vi "4 en linea.vi"() -> ()   [LabVIEW 2021]
panel:
  in  "Restet Marcador":bool
  out "Player Verde":dbl
  out "Player Rojo":dbl
  in  "OK Button":bool
  out "verde":bool
  in  "col7":bool
  in  "col6":bool
  in  "col5":bool
  in  "col4":bool
  in  "col3":bool
  in  "col2":bool
  in  "col1":bool
  in  "Ring 42":u16(ring)
  in  "Ring 41":u16(ring)
  in  "Ring 40":u16(ring)
  in  "Ring 39":u16(ring)
  in  "Ring 38":u16(ring)
  in  "Ring 37":u16(ring)
  in  "Ring 36":u16(ring)
  in  "Ring 35":u16(ring)
  in  "Ring 34":u16(ring)
  in  "Ring 33":u16(ring)
  in  "Ring 32":u16(ring)
  in  "Ring 31":u16(ring)
  in  "Ring 30":u16(ring)
  in  "Ring 29":u16(ring)
  in  "Ring 28":u16(ring)
  in  "Ring 27":u16(ring)
  in  "Ring 26":u16(ring)
  in  "Ring 25":u16(ring)
  in  "Ring 24":u16(ring)
  in  "Ring 23":u16(ring)
  in  "Ring 22":u16(ring)
  in  "Ring 21":u16(ring)
  in  "Ring 20":u16(ring)
  in  "Ring 19":u16(ring)
  in  "Ring 18":u16(ring)
  in  "Ring 17":u16(ring)
  in  "Ring 16":u16(ring)
  in  "Ring 15":u16(ring)
  in  "Ring 14":u16(ring)
  in  "Ring 13":u16(ring)
  in  "Ring 12":u16(ring)
  in  "Ring 11":u16(ring)
  in  "Ring 10":u16(ring)
  in  "Ring 9":u16(ring)
  in  "Ring 8":u16(ring)
  in  "Ring 7":u16(ring)
  in  "Ring 6":u16(ring)
  in  "Ring 5":u16(ring)
  in  "Ring 4":u16(ring)
  in  "Ring 3":u16(ring)
  in  "Ring 2":u16(ring)
  in  "Ring 1":u16(ring)
  # "4 EN LINEA"
  # "TURNO"
  # "MARCADOR"
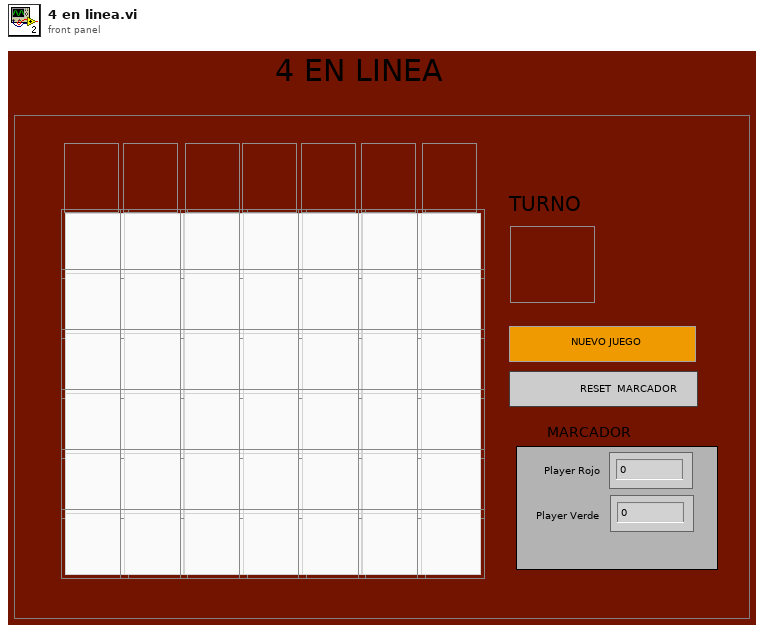
[diagram p1: front panel]
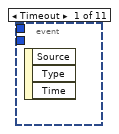
[diagram p12: hidden frame]
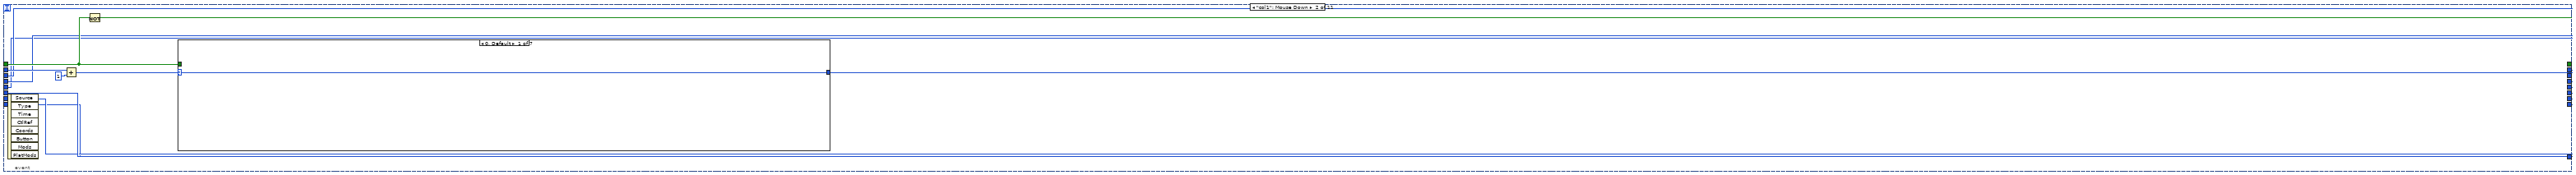
[diagram p13: hidden frame]
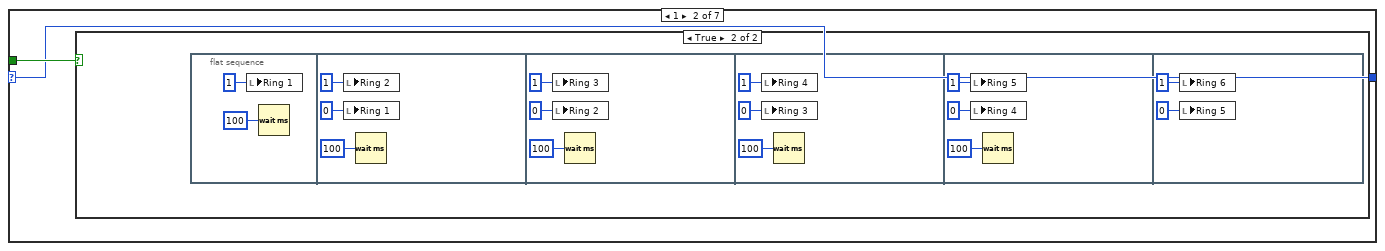
[diagram p14: hidden frame]
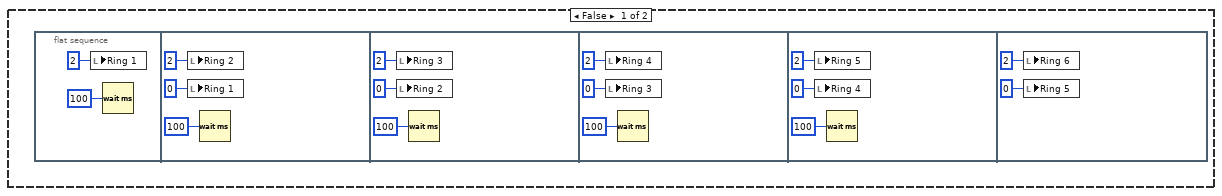
[diagram p15: hidden frame]
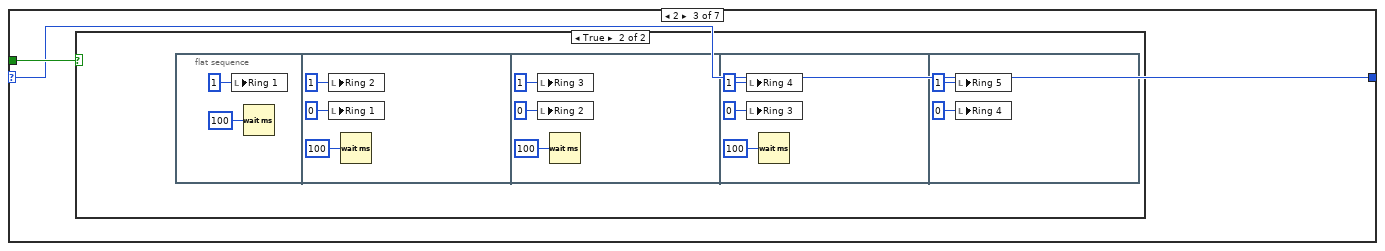
[diagram p16: hidden frame]
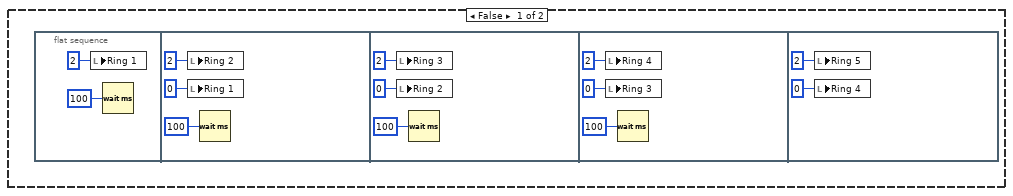
[diagram p17: hidden frame]
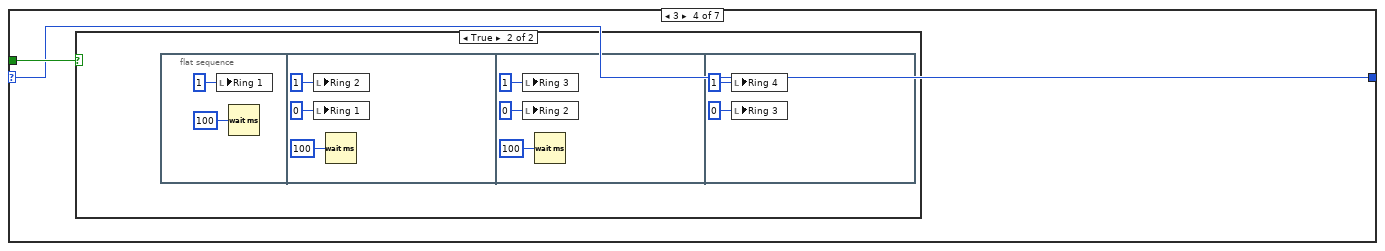
[diagram p18: hidden frame]
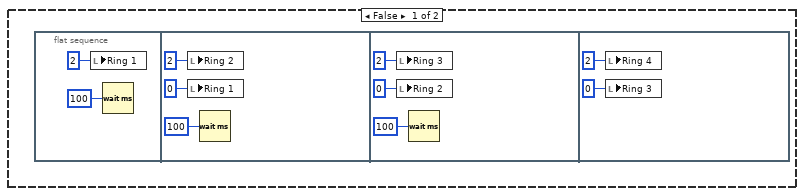
[diagram p19: hidden frame]
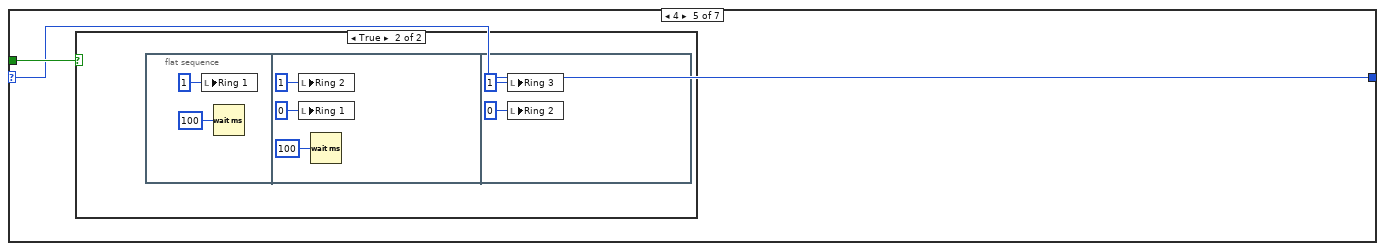
[diagram p20: hidden frame]
diagram:
  w2 = u16 0 ("Ring 42")
  w3 = u16 0 ("Ring 36")
  w4 = u16 0 ("Ring 30")
  w5 = u16 0 ("Ring 24")
  w6 = u16 0 ("Ring 18")
  w7 = u16 0 ("Ring 12")
  w8 = 0
  n1 = local write "Ring 1"(w8) -> ()
  n2 = local write "Ring 6"(w8) -> ()
  n3 = local write "Ring 5"(w8) -> ()
  n4 = local write "Ring 4"(w8) -> ()
  n5 = local write "Ring 3"(w8) -> ()
  n6 = local write "Ring 2"(w8) -> ()
  n7 = local write "Ring 7"(w7) -> ()
  n8 = local write "Ring 12"(w7) -> ()
  n9 = local write "Ring 11"(w7) -> ()
  n10 = local write "Ring 10"(w7) -> ()
  n11 = local write "Ring 9"(w7) -> ()
  n12 = local write "Ring 8"(w7) -> ()
  n13 = local write "Ring 13"(w6) -> ()
  n14 = local write "Ring 18"(w6) -> ()
  n15 = local write "Ring 17"(w6) -> ()
  n16 = local write "Ring 16"(w6) -> ()
  n17 = local write "Ring 15"(w6) -> ()
  n18 = local write "Ring 14"(w6) -> ()
  n19 = local write "Ring 19"(w5) -> ()
  n20 = local write "Ring 24"(w5) -> ()
  n21 = local write "Ring 23"(w5) -> ()
  n22 = local write "Ring 22"(w5) -> ()
  n23 = local write "Ring 21"(w5) -> ()
  n24 = local write "Ring 20"(w5) -> ()
  n25 = local write "Ring 25"(w4) -> ()
  n26 = local write "Ring 30"(w4) -> ()
  n27 = local write "Ring 29"(w4) -> ()
  n28 = local write "Ring 28"(w4) -> ()
  n29 = local write "Ring 27"(w4) -> ()
  n30 = local write "Ring 26"(w4) -> ()
  n31 = local write "Ring 31"(w3) -> ()
  n32 = local write "Ring 36"(w3) -> ()
  n33 = local write "Ring 35"(w3) -> ()
  n34 = local write "Ring 34"(w3) -> ()
  n35 = local write "Ring 33"(w3) -> ()
  n36 = local write "Ring 32"(w3) -> ()
  n37 = local write "Ring 37"(w2) -> ()
  n38 = local write "Ring 42"(w2) -> ()
  n39 = local write "Ring 41"(w2) -> ()
  n40 = local write "Ring 40"(w2) -> ()
  n41 = local write "Ring 39"(w2) -> ()
  n42 = local write "Ring 38"(w2) -> ()
  n43 = while {
    shift-right: [w2185] -> _
    shift-left: FALSE ("verde") -> [w94]
    shift-right: [w2184] -> _
    shift-left: _ -> [w2182]
    shift-right: [w2183] -> _
    shift-left: _ -> [w2181]
    shift-right: [w2180] -> _
    shift-left: _ -> [w2178]
    shift-right: [w2179] -> _
    shift-left: _ -> [w2177]
    shift-right: [w2175] -> _
    shift-left: _ -> [w2176]
    shift-right: [w2173] -> _
    shift-left: _ -> [w2174]
    shift-right: [w2171] -> _
    shift-left: _ -> [w2172]
    stop <- FALSE stop-if-true
    n44 = local write "verde"(w94) -> ()
    n45 = local read "Ring 5"() -> (w2154:u16)
    n46 = local read "Ring 4"() -> (w2152:u16)
    n47 = local read "Ring 3"() -> (w2150:u16)
    n48 = local read "Ring 2"() -> (w2148:u16)
    n49 = local read "Ring 3"() -> (w2167:u16)
    n50 = local read "Ring 4"() -> (w2168:u16)
    n51 = local read "Ring 5"() -> (w2169:u16)
    n52 = local read "Ring 6"() -> (w2170:u16)
    n53 = local read "Ring 4"() -> (w2137:u16)
    n54 = local read "Ring 3"() -> (w2134:u16)
    n55 = local read "Ring 2"() -> (w2135:u16)
    n56 = local read "Ring 1"() -> (w2136:u16)
    n57 = local read "Ring 42"() -> (w1578:u16)
    n58 = local read "Ring 36"() -> (w1577:u16)
    n59 = local read "Ring 30"() -> (w1576:u16)
    n60 = local read "Ring 24"() -> (w1575:u16)
    n61 = local read "Ring 36"() -> (w1582:u16)
    n62 = local read "Ring 30"() -> (w1581:u16)
    n63 = local read "Ring 24"() -> (w1580:u16)
    n64 = local read "Ring 18"() -> (w1579:u16)
    n65 = local read "Ring 30"() -> (w1586:u16)
    n66 = local read "Ring 24"() -> (w1585:u16)
    n67 = local read "Ring 18"() -> (w1584:u16)
    n68 = local read "Ring 12"() -> (w1583:u16)
    n69 = local read "Ring 24"() -> (w1590:u16)
    n70 = local read "Ring 18"() -> (w1589:u16)
    n71 = local read "Ring 12"() -> (w1588:u16)
    n72 = local read "Ring 6"() -> (w1587:u16)
    n73 = event shown="[7] \"col7\": Mouse Down" {
      selector: _ -> [_ _ _ _ _ _ _ _ _ _ _]
      dyn-events: _ -> [_ _ _ _ _ _ _ _ _ _ _]
      timeout: _ -> [_ _ _ _ _ _ _ _ _ _ _]
      tunnel: w94 -> [_ w2225 w2352 w2474 w2600 w2729 w2857 w2977 _ w3106 _]
      tunnel: [_ w2226 w2353 w2475 w2599 w2730 w2856 w2978 _ w3106 w3115] -> w2185
      tunnel: [_ w2224 w2347 w2478 w2603 w2725 w2855 w2984 _ _ _] -> w2184
      tunnel: [_ w2220 w2351 w2479 w2602 w2726 w2854 w2983 _ w3112 _] -> w2183
      tunnel: w2182 -> [_ w2223 w2347 w2478 w2603 w2725 w2855 w2984 _ w3113 _]
      tunnel: w2181 -> [_ w2220 w2350 w2479 w2602 w2726 w2854 w2983 _ w3112 _]
      tunnel: [_ w2219 w2346 w2480 w2601 w2727 w2853 w2982 _ w3111 _] -> w2180
      tunnel: [_ w2218 w2345 w2472 w2605 w2728 w2852 w2981 _ w3110 _] -> w2179
      tunnel: w2178 -> [_ w2219 w2346 w2473 w2601 w2727 w2853 w2982 _ w3111 _]
      tunnel: w2177 -> [_ w2218 w2345 w2472 w2604 w2728 w2852 w2981 _ w3110 _]
      tunnel: w2176 -> [_ w2217 w2344 w2471 w2598 w2733 w2851 w2980 _ w3109 _]
      tunnel: [_ w2217 w2344 w2471 w2598 w2731 w2851 w2980 _ w3109 _] -> w2175
      tunnel: w2174 -> [_ w2216 w2343 w2470 w2597 w2724 w2860 w2979 _ w3108 _]
      tunnel: [_ w2216 w2343 w2470 w2597 w2724 w2858 w2979 _ w3108 _] -> w2173
      tunnel: w2172 -> [_ w2215 w2342 w2469 w2596 w2723 w2850 w2987 _ w3107 _]
      tunnel: [_ w2215 w2342 w2469 w2596 w2723 w2850 w2985 _ w3107 _] -> w2171
      tunnel: [_ _ _ _ _ _ _ _ _ w3113 _] -> _
      event Timeout {
        n74 = event-data() -> ()  [unwired: 1 in, 3 out]
      }
      event "col1": Mouse Down {
        n75 = event-data() -> ()  [unwired: 1 in, 8 out]
        n76 = Add(x=w2223, y=1) -> (x+y=w2222:i32)
        n77 = Not(x=w2225) -> (.not. x?=w2226:bool)
        n78 = case shown="0, Default" w2222 {
          selector: w2222 -> [w2227 w2228 w2262 w2290 w2312 w2328 w2338]
          tunnel: w2225 -> [_ w2229 w2263 w2291 w2313 w2329 w2339]
          tunnel: [w2227 w2228 w2262 w2290 w2312 w2328 w2338] -> w2224
          frame 0, Default {
          }
          frame 1 {
            n79 = case shown="True" w2229 {
              frame False {
                n80 = flat-sequence {
                  frame #0 {
                    n81 = local write "Ring 1"(u16 2 ("Ring 1")) -> ()
                    n82 = Wait (ms)(milliseconds to wait=u32 100) -> ()  [unwired: 1 out]
                  }
                  frame #1 {
                    n83 = local write "Ring 2"(u16 2 ("Ring 2")) -> ()
                    n84 = local write "Ring 1"(u16 0 ("Ring 1")) -> ()
                    n85 = Wait (ms)(milliseconds to wait=u32 100) -> ()  [unwired: 1 out]
                  }
                  frame #2 {
                    n86 = local write "Ring 3"(u16 2 ("Ring 3")) -> ()
                    n87 = local write "Ring 2"(u16 0 ("Ring 2")) -> ()
                    n88 = Wait (ms)(milliseconds to wait=u32 100) -> ()  [unwired: 1 out]
                  }
                  frame #3 {
                    n89 = local write "Ring 4"(u16 2 ("Ring 4")) -> ()
                    n90 = local write "Ring 3"(u16 0 ("Ring 3")) -> ()
                    n91 = Wait (ms)(milliseconds to wait=u32 100) -> ()  [unwired: 1 out]
                  }
                  frame #4 {
                    n92 = local write "Ring 5"(u16 2 ("Ring 5")) -> ()
                    n93 = local write "Ring 4"(u16 0 ("Ring 4")) -> ()
                    n94 = Wait (ms)(milliseconds to wait=u32 100) -> ()  [unwired: 1 out]
                  }
                  frame #5 {
                    n95 = local write "Ring 6"(u16 2 ("Ring 6")) -> ()
                    n96 = local write "Ring 5"(u16 0 ("Ring 5")) -> ()
                  }
                }
              }
              frame True {
                n97 = flat-sequence {
                  frame #0 {
                    n98 = local write "Ring 1"(u16 1 ("Ring 1")) -> ()
                    n99 = Wait (ms)(milliseconds to wait=u32 100) -> ()  [unwired: 1 out]
                  }
                  frame #1 {
                    n100 = local write "Ring 2"(u16 1 ("Ring 2")) -> ()
                    n101 = local write "Ring 1"(u16 0 ("Ring 1")) -> ()
                    n102 = Wait (ms)(milliseconds to wait=u32 100) -> ()  [unwired: 1 out]
                  }
                  frame #2 {
                    n103 = local write "Ring 3"(u16 1 ("Ring 3")) -> ()
                    n104 = local write "Ring 2"(u16 0 ("Ring 2")) -> ()
                    n105 = Wait (ms)(milliseconds to wait=u32 100) -> ()  [unwired: 1 out]
                  }
                  frame #3 {
                    n106 = local write "Ring 4"(u16 1 ("Ring 4")) -> ()
                    n107 = local write "Ring 3"(u16 0 ("Ring 3")) -> ()
                    n108 = Wait (ms)(milliseconds to wait=u32 100) -> ()  [unwired: 1 out]
                  }
                  frame #4 {
                    n109 = local write "Ring 5"(u16 1 ("Ring 5")) -> ()
                    n110 = local write "Ring 4"(u16 0 ("Ring 4")) -> ()
                    n111 = Wait (ms)(milliseconds to wait=u32 100) -> ()  [unwired: 1 out]
                  }
                  frame #5 {
                    n112 = local write "Ring 6"(u16 1 ("Ring 6")) -> ()
                    n113 = local write "Ring 5"(u16 0 ("Ring 5")) -> ()
                  }
                }
              }
            }
          }
          frame 2 {
            n114 = case shown="True" w2263 {
              frame False {
                n115 = flat-sequence {
                  frame #0 {
                    n116 = local write "Ring 1"(u16 2 ("Ring 1")) -> ()
                    n117 = Wait (ms)(milliseconds to wait=u32 100) -> ()  [unwired: 1 out]
                  }
                  frame #1 {
                    n118 = local write "Ring 2"(u16 2 ("Ring 2")) -> ()
                    n119 = local write "Ring 1"(u16 0 ("Ring 1")) -> ()
                    n120 = Wait (ms)(milliseconds to wait=u32 100) -> ()  [unwired: 1 out]
                  }
                  frame #2 {
                    n121 = local write "Ring 3"(u16 2 ("Ring 3")) -> ()
                    n122 = local write "Ring 2"(u16 0 ("Ring 2")) -> ()
                    n123 = Wait (ms)(milliseconds to wait=u32 100) -> ()  [unwired: 1 out]
                  }
                  frame #3 {
                    n124 = local write "Ring 4"(u16 2 ("Ring 4")) -> ()
                    n125 = local write "Ring 3"(u16 0 ("Ring 3")) -> ()
                    n126 = Wait (ms)(milliseconds to wait=u32 100) -> ()  [unwired: 1 out]
                  }
                  frame #4 {
                    n127 = local write "Ring 5"(u16 2 ("Ring 5")) -> ()
                    n128 = local write "Ring 4"(u16 0 ("Ring 4")) -> ()
                  }
                }
              }
              frame True {
                n129 = flat-sequence {
                  frame #0 {
                    n130 = local write "Ring 1"(u16 1 ("Ring 1")) -> ()
                    n131 = Wait (ms)(milliseconds to wait=u32 100) -> ()  [unwired: 1 out]
                  }
                  frame #1 {
                    n132 = local write "Ring 2"(u16 1 ("Ring 2")) -> ()
                    n133 = local write "Ring 1"(u16 0 ("Ring 1")) -> ()
                    n134 = Wait (ms)(milliseconds to wait=u32 100) -> ()  [unwired: 1 out]
                  }
                  frame #2 {
                    n135 = local write "Ring 3"(u16 1 ("Ring 3")) -> ()
                    n136 = local write "Ring 2"(u16 0 ("Ring 2")) -> ()
                    n137 = Wait (ms)(milliseconds to wait=u32 100) -> ()  [unwired: 1 out]
                  }
                  frame #3 {
                    n138 = local write "Ring 4"(u16 1 ("Ring 4")) -> ()
                    n139 = local write "Ring 3"(u16 0 ("Ring 3")) -> ()
                    n140 = Wait (ms)(milliseconds to wait=u32 100) -> ()  [unwired: 1 out]
                  }
                  frame #4 {
                    n141 = local write "Ring 5"(u16 1 ("Ring 5")) -> ()
                    n142 = local write "Ring 4"(u16 0 ("Ring 4")) -> ()
                  }
                }
              }
            }
          }
          frame 3 {
            n143 = case shown="True" w2291 {
              frame False {
                n144 = flat-sequence {
                  frame #0 {
                    n145 = local write "Ring 1"(u16 2 ("Ring 1")) -> ()
                    n146 = Wait (ms)(milliseconds to wait=u32 100) -> ()  [unwired: 1 out]
                  }
                  frame #1 {
                    n147 = local write "Ring 2"(u16 2 ("Ring 2")) -> ()
                    n148 = local write "Ring 1"(u16 0 ("Ring 1")) -> ()
                    n149 = Wait (ms)(milliseconds to wait=u32 100) -> ()  [unwired: 1 out]
                  }
                  frame #2 {
                    n150 = local write "Ring 3"(u16 2 ("Ring 3")) -> ()
                    n151 = local write "Ring 2"(u16 0 ("Ring 2")) -> ()
                    n152 = Wait (ms)(milliseconds to wait=u32 100) -> ()  [unwired: 1 out]
                  }
                  frame #3 {
                    n153 = local write "Ring 4"(u16 2 ("Ring 4")) -> ()
                    n154 = local write "Ring 3"(u16 0 ("Ring 3")) -> ()
                  }
                }
              }
              frame True {
                n155 = flat-sequence {
                  frame #0 {
                    n156 = local write "Ring 1"(u16 1 ("Ring 1")) -> ()
                    n157 = Wait (ms)(milliseconds to wait=u32 100) -> ()  [unwired: 1 out]
                  }
                  frame #1 {
                    n158 = local write "Ring 2"(u16 1 ("Ring 2")) -> ()
                    n159 = local write "Ring 1"(u16 0 ("Ring 1")) -> ()
                    n160 = Wait (ms)(milliseconds to wait=u32 100) -> ()  [unwired: 1 out]
                  }
                  frame #2 {
                    n161 = local write "Ring 3"(u16 1 ("Ring 3")) -> ()
                    n162 = local write "Ring 2"(u16 0 ("Ring 2")) -> ()
                    n163 = Wait (ms)(milliseconds to wait=u32 100) -> ()  [unwired: 1 out]
                  }
                  frame #3 {
                    n164 = local write "Ring 4"(u16 1 ("Ring 4")) -> ()
                    n165 = local write "Ring 3"(u16 0 ("Ring 3")) -> ()
                  }
                }
              }
            }
          }
          frame 4 {
            n166 = case shown="True" w2313 {
              frame False {
                n167 = flat-sequence {
                  frame #0 {
                    n168 = local write "Ring 1"(u16 2 ("Ring 1")) -> ()
                    n169 = Wait (ms)(milliseconds to wait=u32 100) -> ()  [unwired: 1 out]
                  }
                  frame #1 {
                    n170 = local write "Ring 2"(u16 2 ("Ring 2")) -> ()
                    n171 = local write "Ring 1"(u16 0 ("Ring 1")) -> ()
                    n172 = Wait (ms)(milliseconds to wait=u32 100) -> ()  [unwired: 1 out]
                  }
                  frame #2 {
                    n173 = local write "Ring 3"(u16 2 ("Ring 3")) -> ()
                    n174 = local write "Ring 2"(u16 0 ("Ring 2")) -> ()
                  }
                }
              }
              frame True {
                n175 = flat-sequence {
                  frame #0 {
                    n176 = local write "Ring 1"(u16 1 ("Ring 1")) -> ()
                    n177 = Wait (ms)(milliseconds to wait=u32 100) -> ()  [unwired: 1 out]
                  }
                  frame #1 {
                    n178 = local write "Ring 2"(u16 1 ("Ring 2")) -> ()
                    n179 = local write "Ring 1"(u16 0 ("Ring 1")) -> ()
                    n180 = Wait (ms)(milliseconds to wait=u32 100) -> ()  [unwired: 1 out]
                  }
                  frame #2 {
                    n181 = local write "Ring 3"(u16 1 ("Ring 3")) -> ()
                    n182 = local write "Ring 2"(u16 0 ("Ring 2")) -> ()
                  }
                }
              }
            }
          }
          frame 5 {
            n183 = case shown="True" w2329 {
              frame False {
                n184 = flat-sequence {
                  frame #0 {
                    n185 = local write "Ring 1"(u16 2 ("Ring 1")) -> ()
                    n186 = Wait (ms)(milliseconds to wait=u32 100) -> ()  [unwired: 1 out]
                  }
                  frame #1 {
                    n187 = local write "Ring 2"(u16 2 ("Ring 2")) -> ()
                    n188 = local write "Ring 1"(u16 0 ("Ring 1")) -> ()
                  }
                }
              }
              frame True {
                n189 = flat-sequence {
                  frame #0 {
                    n190 = local write "Ring 1"(u16 1 ("Ring 1")) -> ()
                    n191 = Wait (ms)(milliseconds to wait=u32 100) -> ()  [unwired: 1 out]
                  }
                  frame #1 {
                    n192 = local write "Ring 2"(u16 1 ("Ring 2")) -> ()
                    n193 = local write "Ring 1"(u16 0 ("Ring 1")) -> ()
                  }
                }
              }
            }
          }
          frame 6 {
            n194 = case shown="True" w2339 {
              frame False {
                n195 = flat-sequence {
                  frame #0 {
                    n196 = local write "Ring 1"(u16 2 ("Ring 1")) -> ()
                  }
                }
              }
              frame True {
                n197 = flat-sequence {
                  frame #0 {
                    n198 = local write "Ring 1"(u16 1 ("Ring 1")) -> ()
                  }
                }
              }
            }
          }
        }
      }
      event "col2": Mouse Down {
        n199 = event-data() -> ()  [unwired: 1 in, 8 out]
        n200 = Add(x=w2350, y=1) -> (x+y=w2349:i32)
        n201 = Not(x=w2352) -> (.not. x?=w2353:bool)
        n202 = case shown="1" w2349 {
          selector: w2349 -> [w2354 w2355 w2389 w2417 w2439 w2455 w2465]
          tunnel: w2352 -> [_ w2356 w2390 w2418 w2440 w2456 w2466]
          tunnel: [w2354 w2355 w2389 w2417 w2439 w2455 w2465] -> w2351
          frame 0, Default {
          }
          frame 1 {
            n203 = case shown="False" w2356 {
              frame False {
                n204 = flat-sequence {
                  frame #0 {
                    n205 = local write "Ring 7"(u16 2 ("Ring 1")) -> ()
                    n206 = Wait (ms)(milliseconds to wait=u32 100) -> ()  [unwired: 1 out]
                  }
                  frame #1 {
                    n207 = local write "Ring 8"(u16 2 ("Ring 2")) -> ()
                    n208 = local write "Ring 7"(u16 0 ("Ring 1")) -> ()
                    n209 = Wait (ms)(milliseconds to wait=u32 100) -> ()  [unwired: 1 out]
                  }
                  frame #2 {
                    n210 = local write "Ring 9"(u16 2 ("Ring 3")) -> ()
                    n211 = local write "Ring 8"(u16 0 ("Ring 2")) -> ()
                    n212 = Wait (ms)(milliseconds to wait=u32 100) -> ()  [unwired: 1 out]
                  }
                  frame #3 {
                    n213 = local write "Ring 10"(u16 2 ("Ring 4")) -> ()
                    n214 = local write "Ring 9"(u16 0 ("Ring 3")) -> ()
                    n215 = Wait (ms)(milliseconds to wait=u32 100) -> ()  [unwired: 1 out]
                  }
                  frame #4 {
                    n216 = local write "Ring 11"(u16 2 ("Ring 5")) -> ()
                    n217 = local write "Ring 10"(u16 0 ("Ring 4")) -> ()
                    n218 = Wait (ms)(milliseconds to wait=u32 100) -> ()  [unwired: 1 out]
                  }
                  frame #5 {
                    n219 = local write "Ring 12"(u16 2 ("Ring 6")) -> ()
                    n220 = local write "Ring 11"(u16 0 ("Ring 5")) -> ()
                  }
                }
              }
              frame True {
                n221 = flat-sequence {
                  frame #0 {
                    n222 = local write "Ring 7"(u16 1 ("Ring 1")) -> ()
                    n223 = Wait (ms)(milliseconds to wait=u32 100) -> ()  [unwired: 1 out]
                  }
                  frame #1 {
                    n224 = local write "Ring 8"(u16 1 ("Ring 2")) -> ()
                    n225 = local write "Ring 7"(u16 0 ("Ring 1")) -> ()
                    n226 = Wait (ms)(milliseconds to wait=u32 100) -> ()  [unwired: 1 out]
                  }
                  frame #2 {
                    n227 = local write "Ring 9"(u16 1 ("Ring 3")) -> ()
                    n228 = local write "Ring 8"(u16 0 ("Ring 2")) -> ()
                    n229 = Wait (ms)(milliseconds to wait=u32 100) -> ()  [unwired: 1 out]
                  }
                  frame #3 {
                    n230 = local write "Ring 10"(u16 1 ("Ring 4")) -> ()
                    n231 = local write "Ring 9"(u16 0 ("Ring 3")) -> ()
                    n232 = Wait (ms)(milliseconds to wait=u32 100) -> ()  [unwired: 1 out]
                  }
                  frame #4 {
                    n233 = local write "Ring 11"(u16 1 ("Ring 5")) -> ()
                    n234 = local write "Ring 10"(u16 0 ("Ring 4")) -> ()
                    n235 = Wait (ms)(milliseconds to wait=u32 100) -> ()  [unwired: 1 out]
                  }
                  frame #5 {
                    n236 = local write "Ring 12"(u16 1 ("Ring 6")) -> ()
                    n237 = local write "Ring 11"(u16 0 ("Ring 5")) -> ()
                  }
                }
              }
            }
          }
          frame 2 {
            n238 = case shown="True" w2390 {
              frame False {
                n239 = flat-sequence {
                  frame #0 {
                    n240 = local write "Ring 7"(u16 2 ("Ring 1")) -> ()
                    n241 = Wait (ms)(milliseconds to wait=u32 100) -> ()  [unwired: 1 out]
                  }
                  frame #1 {
                    n242 = local write "Ring 8"(u16 2 ("Ring 2")) -> ()
                    n243 = local write "Ring 7"(u16 0 ("Ring 1")) -> ()
                    n244 = Wait (ms)(milliseconds to wait=u32 100) -> ()  [unwired: 1 out]
                  }
                  frame #2 {
                    n245 = local write "Ring 9"(u16 2 ("Ring 3")) -> ()
                    n246 = local write "Ring 8"(u16 0 ("Ring 2")) -> ()
                    n247 = Wait (ms)(milliseconds to wait=u32 100) -> ()  [unwired: 1 out]
                  }
                  frame #3 {
                    n248 = local write "Ring 10"(u16 2 ("Ring 4")) -> ()
                    n249 = local write "Ring 9"(u16 0 ("Ring 3")) -> ()
                    n250 = Wait (ms)(milliseconds to wait=u32 100) -> ()  [unwired: 1 out]
                  }
                  frame #4 {
                    n251 = local write "Ring 11"(u16 2 ("Ring 5")) -> ()
                    n252 = local write "Ring 10"(u16 0 ("Ring 4")) -> ()
                  }
                }
              }
              frame True {
                n253 = flat-sequence {
                  frame #0 {
                    n254 = local write "Ring 7"(u16 1 ("Ring 1")) -> ()
                    n255 = Wait (ms)(milliseconds to wait=u32 100) -> ()  [unwired: 1 out]
                  }
                  frame #1 {
                    n256 = local write "Ring 8"(u16 1 ("Ring 2")) -> ()
                    n257 = local write "Ring 7"(u16 0 ("Ring 1")) -> ()
                    n258 = Wait (ms)(milliseconds to wait=u32 100) -> ()  [unwired: 1 out]
                  }
                  frame #2 {
                    n259 = local write "Ring 9"(u16 1 ("Ring 3")) -> ()
                    n260 = local write "Ring 8"(u16 0 ("Ring 2")) -> ()
                    n261 = Wait (ms)(milliseconds to wait=u32 100) -> ()  [unwired: 1 out]
                  }
                  frame #3 {
                    n262 = local write "Ring 10"(u16 1 ("Ring 4")) -> ()
                    n263 = local write "Ring 9"(u16 0 ("Ring 3")) -> ()
                    n264 = Wait (ms)(milliseconds to wait=u32 100) -> ()  [unwired: 1 out]
                  }
                  frame #4 {
                    n265 = local write "Ring 11"(u16 1 ("Ring 5")) -> ()
                    n266 = local write "Ring 10"(u16 0 ("Ring 4")) -> ()
                  }
                }
              }
            }
          }
          frame 3 {
            n267 = case shown="False" w2418 {
              frame False {
                n268 = flat-sequence {
                  frame #0 {
                    n269 = local write "Ring 7"(u16 2 ("Ring 1")) -> ()
                    n270 = Wait (ms)(milliseconds to wait=u32 100) -> ()  [unwired: 1 out]
                  }
                  frame #1 {
                    n271 = local write "Ring 8"(u16 2 ("Ring 2")) -> ()
                    n272 = local write "Ring 7"(u16 0 ("Ring 1")) -> ()
                    n273 = Wait (ms)(milliseconds to wait=u32 100) -> ()  [unwired: 1 out]
                  }
                  frame #2 {
                    n274 = local write "Ring 9"(u16 2 ("Ring 3")) -> ()
                    n275 = local write "Ring 8"(u16 0 ("Ring 2")) -> ()
                    n276 = Wait (ms)(milliseconds to wait=u32 100) -> ()  [unwired: 1 out]
                  }
                  frame #3 {
                    n277 = local write "Ring 10"(u16 2 ("Ring 4")) -> ()
                    n278 = local write "Ring 9"(u16 0 ("Ring 3")) -> ()
                  }
                }
              }
              frame True {
                n279 = flat-sequence {
                  frame #0 {
                    n280 = local write "Ring 7"(u16 1 ("Ring 1")) -> ()
                    n281 = Wait (ms)(milliseconds to wait=u32 100) -> ()  [unwired: 1 out]
                  }
                  frame #1 {
                    n282 = local write "Ring 8"(u16 1 ("Ring 2")) -> ()
                    n283 = local write "Ring 7"(u16 0 ("Ring 1")) -> ()
                    n284 = Wait (ms)(milliseconds to wait=u32 100) -> ()  [unwired: 1 out]
                  }
                  frame #2 {
                    n285 = local write "Ring 9"(u16 1 ("Ring 3")) -> ()
                    n286 = local write "Ring 8"(u16 0 ("Ring 2")) -> ()
                    n287 = Wait (ms)(milliseconds to wait=u32 100) -> ()  [unwired: 1 out]
                  }
                  frame #3 {
                    n288 = local write "Ring 10"(u16 1 ("Ring 4")) -> ()
                    n289 = local write "Ring 9"(u16 0 ("Ring 3")) -> ()
                  }
                }
              }
            }
          }
          frame 4 {
            n290 = case shown="True" w2440 {
              frame False {
                n291 = flat-sequence {
                  frame #0 {
                    n292 = local write "Ring 7"(u16 2 ("Ring 1")) -> ()
                    n293 = Wait (ms)(milliseconds to wait=u32 100) -> ()  [unwired: 1 out]
                  }
                  frame #1 {
                    n294 = local write "Ring 8"(u16 2 ("Ring 2")) -> ()
                    n295 = local write "Ring 7"(u16 0 ("Ring 1")) -> ()
                    n296 = Wait (ms)(milliseconds to wait=u32 100) -> ()  [unwired: 1 out]
                  }
                  frame #2 {
                    n297 = local write "Ring 9"(u16 2 ("Ring 3")) -> ()
                    n298 = local write "Ring 8"(u16 0 ("Ring 2")) -> ()
                  }
                }
              }
              frame True {
                n299 = flat-sequence {
                  frame #0 {
                    n300 = local write "Ring 7"(u16 1 ("Ring 1")) -> ()
                    n301 = Wait (ms)(milliseconds to wait=u32 100) -> ()  [unwired: 1 out]
                  }
                  frame #1 {
                    n302 = local write "Ring 8"(u16 1 ("Ring 2")) -> ()
                    n303 = local write "Ring 7"(u16 0 ("Ring 1")) -> ()
                    n304 = Wait (ms)(milliseconds to wait=u32 100) -> ()  [unwired: 1 out]
                  }
                  frame #2 {
                    n305 = local write "Ring 9"(u16 1 ("Ring 3")) -> ()
                    n306 = local write "Ring 8"(u16 0 ("Ring 2")) -> ()
                  }
                }
              }
            }
          }
          frame 5 {
            n307 = case shown="True" w2456 {
              frame False {
                n308 = flat-sequence {
                  frame #0 {
                    n309 = local write "Ring 7"(u16 2 ("Ring 1")) -> ()
                    n310 = Wait (ms)(milliseconds to wait=u32 100) -> ()  [unwired: 1 out]
                  }
                  frame #1 {
                    n311 = local write "Ring 8"(u16 2 ("Ring 2")) -> ()
                    n312 = local write "Ring 7"(u16 0 ("Ring 1")) -> ()
                  }
                }
              }
              frame True {
                n313 = flat-sequence {
                  frame #0 {
                    n314 = local write "Ring 7"(u16 1 ("Ring 1")) -> ()
                    n315 = Wait (ms)(milliseconds to wait=u32 100) -> ()  [unwired: 1 out]
                  }
                  frame #1 {
                    n316 = local write "Ring 8"(u16 1 ("Ring 2")) -> ()
                    n317 = local write "Ring 7"(u16 0 ("Ring 1")) -> ()
                  }
                }
              }
            }
          }
          frame 6 {
            n318 = case shown="False" w2466 {
              frame False {
                n319 = flat-sequence {
                  frame #0 {
                    n320 = local write "Ring 7"(u16 2 ("Ring 1")) -> ()
                  }
                }
              }
              frame True {
                n321 = flat-sequence {
                  frame #0 {
                    n322 = local write "Ring 7"(u16 1 ("Ring 1")) -> ()
                  }
                }
              }
            }
          }
        }
      }
      event "col3": Mouse Down {
        n323 = event-data() -> ()  [unwired: 1 in, 8 out]
        n324 = Add(x=w2473, y=1) -> (x+y=w2477:i32)
        n325 = Not(x=w2474) -> (.not. x?=w2475:bool)
        n326 = case shown="1" w2477 {
          selector: w2477 -> [w2481 w2482 w2516 w2544 w2566 w2582 w2592]
          tunnel: w2474 -> [_ w2483 w2517 w2545 w2567 w2583 w2593]
          tunnel: [w2481 w2482 w2516 w2544 w2566 w2582 w2592] -> w2480
          frame 0, Default {
          }
          frame 1 {
            n327 = case shown="False" w2483 {
              frame False {
                n328 = flat-sequence {
                  frame #0 {
                    n329 = local write "Ring 13"(u16 2 ("Ring 1")) -> ()
                    n330 = Wait (ms)(milliseconds to wait=u32 100) -> ()  [unwired: 1 out]
                  }
                  frame #1 {
                    n331 = local write "Ring 14"(u16 2 ("Ring 2")) -> ()
                    n332 = local write "Ring 13"(u16 0 ("Ring 1")) -> ()
                    n333 = Wait (ms)(milliseconds to wait=u32 100) -> ()  [unwired: 1 out]
                  }
                  frame #2 {
                    n334 = local write "Ring 15"(u16 2 ("Ring 3")) -> ()
                    n335 = local write "Ring 14"(u16 0 ("Ring 2")) -> ()
                    n336 = Wait (ms)(milliseconds to wait=u32 100) -> ()  [unwired: 1 out]
                  }
                  frame #3 {
                    n337 = local write "Ring 16"(u16 2 ("Ring 4")) -> ()
                    n338 = local write "Ring 15"(u16 0 ("Ring 3")) -> ()
                    n339 = Wait (ms)(milliseconds to wait=u32 100) -> ()  [unwired: 1 out]
                  }
                  frame #4 {
                    n340 = local write "Ring 17"(u16 2 ("Ring 5")) -> ()
                    n341 = local write "Ring 16"(u16 0 ("Ring 4")) -> ()
                    n342 = Wait (ms)(milliseconds to wait=u32 100) -> ()  [unwired: 1 out]
                  }
                  frame #5 {
                    n343 = local write "Ring 18"(u16 2 ("Ring 6")) -> ()
                    n344 = local write "Ring 17"(u16 0 ("Ring 5")) -> ()
                  }
                }
              }
              frame True {
                n345 = flat-sequence {
                  frame #0 {
                    n346 = local write "Ring 13"(u16 1 ("Ring 1")) -> ()
                    n347 = Wait (ms)(milliseconds to wait=u32 100) -> ()  [unwired: 1 out]
                  }
                  frame #1 {
                    n348 = local write "Ring 14"(u16 1 ("Ring 2")) -> ()
                    n349 = local write "Ring 13"(u16 0 ("Ring 1")) -> ()
                    n350 = Wait (ms)(milliseconds to wait=u32 100) -> ()  [unwired: 1 out]
                  }
                  frame #2 {
                    n351 = local write "Ring 15"(u16 1 ("Ring 3")) -> ()
                    n352 = local write "Ring 14"(u16 0 ("Ring 2")) -> ()
                    n353 = Wait (ms)(milliseconds to wait=u32 100) -> ()  [unwired: 1 out]
                  }
                  frame #3 {
                    n354 = local write "Ring 16"(u16 1 ("Ring 4")) -> ()
                    n355 = local write "Ring 15"(u16 0 ("Ring 3")) -> ()
                    n356 = Wait (ms)(milliseconds to wait=u32 100) -> ()  [unwired: 1 out]
                  }
                  frame #4 {
                    n357 = local write "Ring 17"(u16 1 ("Ring 5")) -> ()
                    n358 = local write "Ring 16"(u16 0 ("Ring 4")) -> ()
                    n359 = Wait (ms)(milliseconds to wait=u32 100) -> ()  [unwired: 1 out]
                  }
                  frame #5 {
                    n360 = local write "Ring 18"(u16 1 ("Ring 6")) -> ()
                    n361 = local write "Ring 17"(u16 0 ("Ring 5")) -> ()
                  }
                }
              }
            }
          }
          frame 2 {
            n362 = case shown="True" w2517 {
              frame False {
                n363 = flat-sequence {
                  frame #0 {
                    n364 = local write "Ring 13"(u16 2 ("Ring 1")) -> ()
                    n365 = Wait (ms)(milliseconds to wait=u32 100) -> ()  [unwired: 1 out]
                  }
                  frame #1 {
                    n366 = local write "Ring 14"(u16 2 ("Ring 2")) -> ()
                    n367 = local write "Ring 13"(u16 0 ("Ring 1")) -> ()
                    n368 = Wait (ms)(milliseconds to wait=u32 100) -> ()  [unwired: 1 out]
                  }
                  frame #2 {
                    n369 = local write "Ring 15"(u16 2 ("Ring 3")) -> ()
                    n370 = local write "Ring 14"(u16 0 ("Ring 2")) -> ()
                    n371 = Wait (ms)(milliseconds to wait=u32 100) -> ()  [unwired: 1 out]
                  }
                  frame #3 {
                    n372 = local write "Ring 16"(u16 2 ("Ring 4")) -> ()
                    n373 = local write "Ring 15"(u16 0 ("Ring 3")) -> ()
                    n374 = Wait (ms)(milliseconds to wait=u32 100) -> ()  [unwired: 1 out]
                  }
                  frame #4 {
                    n375 = local write "Ring 17"(u16 2 ("Ring 5")) -> ()
                    n376 = local write "Ring 16"(u16 0 ("Ring 4")) -> ()
                  }
                }
              }
              frame True {
                n377 = flat-sequence {
                  frame #0 {
                    n378 = local write "Ring 13"(u16 1 ("Ring 1")) -> ()
                    n379 = Wait (ms)(milliseconds to wait=u32 100) -> ()  [unwired: 1 out]
                  }
                  frame #1 {
                    n380 = local write "Ring 14"(u16 1 ("Ring 2")) -> ()
                    n381 = local write "Ring 13"(u16 0 ("Ring 1")) -> ()
                    n382 = Wait (ms)(milliseconds to wait=u32 100) -> ()  [unwired: 1 out]
                  }
                  frame #2 {
                    n383 = local write "Ring 15"(u16 1 ("Ring 3")) -> ()
                    n384 = local write "Ring 14"(u16 0 ("Ring 2")) -> ()
                    n385 = Wait (ms)(milliseconds to wait=u32 100) -> ()  [unwired: 1 out]
                  }
                  frame #3 {
                    n386 = local write "Ring 16"(u16 1 ("Ring 4")) -> ()
                    n387 = local write "Ring 15"(u16 0 ("Ring 3")) -> ()
                    n388 = Wait (ms)(milliseconds to wait=u32 100) -> ()  [unwired: 1 out]
                  }
                  frame #4 {
                    n389 = local write "Ring 17"(u16 1 ("Ring 5")) -> ()
                    n390 = local write "Ring 16"(u16 0 ("Ring 4")) -> ()
                  }
                }
              }
            }
          }
          frame 3 {
            n391 = case shown="True" w2545 {
              frame False {
                n392 = flat-sequence {
                  frame #0 {
                    n393 = local write "Ring 13"(u16 2 ("Ring 1")) -> ()
                    n394 = Wait (ms)(milliseconds to wait=u32 100) -> ()  [unwired: 1 out]
                  }
                  frame #1 {
                    n395 = local write "Ring 14"(u16 2 ("Ring 2")) -> ()
                    n396 = local write "Ring 13"(u16 0 ("Ring 1")) -> ()
                    n397 = Wait (ms)(milliseconds to wait=u32 100) -> ()  [unwired: 1 out]
                  }
                  frame #2 {
                    n398 = local write "Ring 15"(u16 2 ("Ring 3")) -> ()
                    n399 = local write "Ring 14"(u16 0 ("Ring 2")) -> ()
                    n400 = Wait (ms)(milliseconds to wait=u32 100) -> ()  [unwired: 1 out]
                  }
                  frame #3 {
                    n401 = local write "Ring 16"(u16 2 ("Ring 4")) -> ()
                    n402 = local write "Ring 15"(u16 0 ("Ring 3")) -> ()
                  }
                }
              }
              frame True {
                n403 = flat-sequence {
                  frame #0 {
                    n404 = local write "Ring 13"(u16 1 ("Ring 1")) -> ()
                    n405 = Wait (ms)(milliseconds to wait=u32 100) -> ()  [unwired: 1 out]
                  }
                  frame #1 {
                    n406 = local write "Ring 14"(u16 1 ("Ring 2")) -> ()
                    n407 = local write "Ring 13"(u16 0 ("Ring 1")) -> ()
                    n408 = Wait (ms)(milliseconds to wait=u32 100) -> ()  [unwired: 1 out]
                  }
                  frame #2 {
                    n409 = local write "Ring 15"(u16 1 ("Ring 3")) -> ()
                    n410 = local write "Ring 14"(u16 0 ("Ring 2")) -> ()
                    n411 = Wait (ms)(milliseconds to wait=u32 100) -> ()  [unwired: 1 out]
                  }
                  frame #3 {
                    n412 = local write "Ring 16"(u16 1 ("Ring 4")) -> ()
                    n413 = local write "Ring 15"(u16 0 ("Ring 3")) -> ()
                  }
                }
              }
            }
          }
          frame 4 {
            n414 = case shown="False" w2567 {
              frame False {
                n415 = flat-sequence {
                  frame #0 {
                    n416 = local write "Ring 13"(u16 2 ("Ring 1")) -> ()
                    n417 = Wait (ms)(milliseconds to wait=u32 100) -> ()  [unwired: 1 out]
                  }
                  frame #1 {
                    n418 = local write "Ring 14"(u16 2 ("Ring 2")) -> ()
                    n419 = local write "Ring 13"(u16 0 ("Ring 1")) -> ()
                    n420 = Wait (ms)(milliseconds to wait=u32 100) -> ()  [unwired: 1 out]
                  }
                  frame #2 {
                    n421 = local write "Ring 15"(u16 2 ("Ring 3")) -> ()
                    n422 = local write "Ring 14"(u16 0 ("Ring 2")) -> ()
                  }
                }
              }
              frame True {
                n423 = flat-sequence {
                  frame #0 {
                    n424 = local write "Ring 13"(u16 1 ("Ring 1")) -> ()
                    n425 = Wait (ms)(milliseconds to wait=u32 100) -> ()  [unwired: 1 out]
                  }
                  frame #1 {
                    n426 = local write "Ring 14"(u16 1 ("Ring 2")) -> ()
                    n427 = local write "Ring 13"(u16 0 ("Ring 1")) -> ()
                    n428 = Wait (ms)(milliseconds to wait=u32 100) -> ()  [unwired: 1 out]
                  }
                  frame #2 {
                    n429 = local write "Ring 15"(u16 1 ("Ring 3")) -> ()
                    n430 = local write "Ring 14"(u16 0 ("Ring 2")) -> ()
                  }
                }
              }
            }
          }
          frame 5 {
            n431 = case shown="False" w2583 {
              frame False {
                n432 = flat-sequence {
                  frame #0 {
                    n433 = local write "Ring 13"(u16 2 ("Ring 1")) -> ()
                    n434 = Wait (ms)(milliseconds to wait=u32 100) -> ()  [unwired: 1 out]
                  }
                  frame #1 {
                    n435 = local write "Ring 14"(u16 2 ("Ring 2")) -> ()
                    n436 = local write "Ring 13"(u16 0 ("Ring 1")) -> ()
                  }
                }
              }
              frame True {
                n437 = flat-sequence {
                  frame #0 {
                    n438 = local write "Ring 13"(u16 1 ("Ring 1")) -> ()
                    n439 = Wait (ms)(milliseconds to wait=u32 100) -> ()  [unwired: 1 out]
                  }
                  frame #1 {
                    n440 = local write "Ring 14"(u16 1 ("Ring 2")) -> ()
                    n441 = local write "Ring 13"(u16 0 ("Ring 1")) -> ()
                  }
                }
              }
            }
          }
          frame 6 {
            n442 = case shown="True" w2593 {
              frame False {
                n443 = flat-sequence {
                  frame #0 {
                    n444 = local write "Ring 13"(u16 2 ("Ring 1")) -> ()
                  }
                }
              }
              frame True {
                n445 = flat-sequence {
                  frame #0 {
                    n446 = local write "Ring 13"(u16 1 ("Ring 1")) -> ()
                  }
                }
              }
            }
          }
        }
      }
      event "col4": Mouse Down {
        n447 = event-data() -> ()  [unwired: 1 in, 8 out]
        n448 = Add(x=w2604, y=1) -> (x+y=w2606:i32)
        n449 = Not(x=w2600) -> (.not. x?=w2599:bool)
        n450 = case shown="6" w2606 {
          selector: w2606 -> [w2608 w2610 w2644 w2672 w2694 w2710 w2720]
          tunnel: [w2608 w2610 w2644 w2672 w2694 w2710 w2720] -> w2605
          tunnel: w2600 -> [_ w2609 w2643 w2671 w2693 w2709 w2719]
          frame 0, Default {
          }
          frame 1 {
            n451 = case shown="True" w2609 {
              frame False {
                n452 = flat-sequence {
                  frame #0 {
                    n453 = local write "Ring 19"(u16 2 ("Ring 1")) -> ()
                    n454 = Wait (ms)(milliseconds to wait=u32 100) -> ()  [unwired: 1 out]
                  }
                  frame #1 {
                    n455 = local write "Ring 20"(u16 2 ("Ring 2")) -> ()
                    n456 = local write "Ring 19"(u16 0 ("Ring 1")) -> ()
                    n457 = Wait (ms)(milliseconds to wait=u32 100) -> ()  [unwired: 1 out]
                  }
                  frame #2 {
                    n458 = local write "Ring 21"(u16 2 ("Ring 3")) -> ()
                    n459 = local write "Ring 20"(u16 0 ("Ring 2")) -> ()
                    n460 = Wait (ms)(milliseconds to wait=u32 100) -> ()  [unwired: 1 out]
                  }
                  frame #3 {
                    n461 = local write "Ring 22"(u16 2 ("Ring 4")) -> ()
                    n462 = local write "Ring 21"(u16 0 ("Ring 3")) -> ()
                    n463 = Wait (ms)(milliseconds to wait=u32 100) -> ()  [unwired: 1 out]
                  }
                  frame #4 {
                    n464 = local write "Ring 23"(u16 2 ("Ring 5")) -> ()
                    n465 = local write "Ring 22"(u16 0 ("Ring 4")) -> ()
                    n466 = Wait (ms)(milliseconds to wait=u32 100) -> ()  [unwired: 1 out]
                  }
                  frame #5 {
                    n467 = local write "Ring 24"(u16 2 ("Ring 6")) -> ()
                    n468 = local write "Ring 23"(u16 0 ("Ring 5")) -> ()
                  }
                }
              }
              frame True {
                n469 = flat-sequence {
                  frame #0 {
                    n470 = local write "Ring 19"(u16 1 ("Ring 1")) -> ()
                    n471 = Wait (ms)(milliseconds to wait=u32 100) -> ()  [unwired: 1 out]
                  }
                  frame #1 {
                    n472 = local write "Ring 20"(u16 1 ("Ring 2")) -> ()
                    n473 = local write "Ring 19"(u16 0 ("Ring 1")) -> ()
                    n474 = Wait (ms)(milliseconds to wait=u32 100) -> ()  [unwired: 1 out]
                  }
                  frame #2 {
                    n475 = local write "Ring 21"(u16 1 ("Ring 3")) -> ()
                    n476 = local write "Ring 20"(u16 0 ("Ring 2")) -> ()
                    n477 = Wait (ms)(milliseconds to wait=u32 100) -> ()  [unwired: 1 out]
                  }
                  frame #3 {
                    n478 = local write "Ring 22"(u16 1 ("Ring 4")) -> ()
                    n479 = local write "Ring 21"(u16 0 ("Ring 3")) -> ()
                    n480 = Wait (ms)(milliseconds to wait=u32 100) -> ()  [unwired: 1 out]
                  }
                  frame #4 {
                    n481 = local write "Ring 23"(u16 1 ("Ring 5")) -> ()
                    n482 = local write "Ring 22"(u16 0 ("Ring 4")) -> ()
                    n483 = Wait (ms)(milliseconds to wait=u32 100) -> ()  [unwired: 1 out]
                  }
                  frame #5 {
                    n484 = local write "Ring 24"(u16 1 ("Ring 6")) -> ()
                    n485 = local write "Ring 23"(u16 0 ("Ring 5")) -> ()
                  }
                }
              }
            }
          }
          frame 2 {
            n486 = case shown="True" w2643 {
              frame False {
                n487 = flat-sequence {
                  frame #0 {
                    n488 = local write "Ring 19"(u16 2 ("Ring 1")) -> ()
                    n489 = Wait (ms)(milliseconds to wait=u32 100) -> ()  [unwired: 1 out]
                  }
                  frame #1 {
                    n490 = local write "Ring 20"(u16 2 ("Ring 2")) -> ()
                    n491 = local write "Ring 19"(u16 0 ("Ring 1")) -> ()
                    n492 = Wait (ms)(milliseconds to wait=u32 100) -> ()  [unwired: 1 out]
                  }
                  frame #2 {
                    n493 = local write "Ring 21"(u16 2 ("Ring 3")) -> ()
                    n494 = local write "Ring 20"(u16 0 ("Ring 2")) -> ()
                    n495 = Wait (ms)(milliseconds to wait=u32 100) -> ()  [unwired: 1 out]
                  }
                  frame #3 {
                    n496 = local write "Ring 22"(u16 2 ("Ring 4")) -> ()
                    n497 = local write "Ring 21"(u16 0 ("Ring 3")) -> ()
                    n498 = Wait (ms)(milliseconds to wait=u32 100) -> ()  [unwired: 1 out]
                  }
                  frame #4 {
                    n499 = local write "Ring 23"(u16 2 ("Ring 5")) -> ()
                    n500 = local write "Ring 22"(u16 0 ("Ring 4")) -> ()
                  }
                }
              }
              frame True {
                n501 = flat-sequence {
                  frame #0 {
                    n502 = local write "Ring 19"(u16 1 ("Ring 1")) -> ()
                    n503 = Wait (ms)(milliseconds to wait=u32 100) -> ()  [unwired: 1 out]
                  }
                  frame #1 {
                    n504 = local write "Ring 20"(u16 1 ("Ring 2")) -> ()
                    n505 = local write "Ring 19"(u16 0 ("Ring 1")) -> ()
                    n506 = Wait (ms)(milliseconds to wait=u32 100) -> ()  [unwired: 1 out]
                  }
                  frame #2 {
                    n507 = local write "Ring 21"(u16 1 ("Ring 3")) -> ()
                    n508 = local write "Ring 20"(u16 0 ("Ring 2")) -> ()
                    n509 = Wait (ms)(milliseconds to wait=u32 100) -> ()  [unwired: 1 out]
                  }
                  frame #3 {
                    n510 = local write "Ring 22"(u16 1 ("Ring 4")) -> ()
                    n511 = local write "Ring 21"(u16 0 ("Ring 3")) -> ()
                    n512 = Wait (ms)(milliseconds to wait=u32 100) -> ()  [unwired: 1 out]
                  }
                  frame #4 {
                    n513 = local write "Ring 23"(u16 1 ("Ring 5")) -> ()
                    n514 = local write "Ring 22"(u16 0 ("Ring 4")) -> ()
                  }
                }
              }
            }
          }
          frame 3 {
            n515 = case shown="False" w2671 {
              frame False {
                n516 = flat-sequence {
                  frame #0 {
                    n517 = local write "Ring 19"(u16 2 ("Ring 1")) -> ()
                    n518 = Wait (ms)(milliseconds to wait=u32 100) -> ()  [unwired: 1 out]
                  }
                  frame #1 {
                    n519 = local write "Ring 20"(u16 2 ("Ring 2")) -> ()
                    n520 = local write "Ring 19"(u16 0 ("Ring 1")) -> ()
                    n521 = Wait (ms)(milliseconds to wait=u32 100) -> ()  [unwired: 1 out]
                  }
                  frame #2 {
                    n522 = local write "Ring 21"(u16 2 ("Ring 3")) -> ()
                    n523 = local write "Ring 20"(u16 0 ("Ring 2")) -> ()
                    n524 = Wait (ms)(milliseconds to wait=u32 100) -> ()  [unwired: 1 out]
                  }
                  frame #3 {
                    n525 = local write "Ring 22"(u16 2 ("Ring 4")) -> ()
                    n526 = local write "Ring 21"(u16 0 ("Ring 3")) -> ()
                  }
                }
              }
              frame True {
                n527 = flat-sequence {
                  frame #0 {
                    n528 = local write "Ring 19"(u16 1 ("Ring 1")) -> ()
                    n529 = Wait (ms)(milliseconds to wait=u32 100) -> ()  [unwired: 1 out]
                  }
                  frame #1 {
                    n530 = local write "Ring 20"(u16 1 ("Ring 2")) -> ()
                    n531 = local write "Ring 19"(u16 0 ("Ring 1")) -> ()
                    n532 = Wait (ms)(milliseconds to wait=u32 100) -> ()  [unwired: 1 out]
                  }
                  frame #2 {
                    n533 = local write "Ring 21"(u16 1 ("Ring 3")) -> ()
                    n534 = local write "Ring 20"(u16 0 ("Ring 2")) -> ()
                    n535 = Wait (ms)(milliseconds to wait=u32 100) -> ()  [unwired: 1 out]
                  }
                  frame #3 {
                    n536 = local write "Ring 22"(u16 1 ("Ring 4")) -> ()
                    n537 = local write "Ring 21"(u16 0 ("Ring 3")) -> ()
                  }
                }
              }
            }
          }
          frame 4 {
            n538 = case shown="False" w2693 {
              frame False {
                n539 = flat-sequence {
                  frame #0 {
                    n540 = local write "Ring 19"(u16 2 ("Ring 1")) -> ()
                    n541 = Wait (ms)(milliseconds to wait=u32 100) -> ()  [unwired: 1 out]
                  }
                  frame #1 {
                    n542 = local write "Ring 20"(u16 2 ("Ring 2")) -> ()
                    n543 = local write "Ring 19"(u16 0 ("Ring 1")) -> ()
                    n544 = Wait (ms)(milliseconds to wait=u32 100) -> ()  [unwired: 1 out]
                  }
                  frame #2 {
                    n545 = local write "Ring 21"(u16 2 ("Ring 3")) -> ()
                    n546 = local write "Ring 20"(u16 0 ("Ring 2")) -> ()
                  }
                }
              }
              frame True {
                n547 = flat-sequence {
                  frame #0 {
                    n548 = local write "Ring 19"(u16 1 ("Ring 1")) -> ()
                    n549 = Wait (ms)(milliseconds to wait=u32 100) -> ()  [unwired: 1 out]
                  }
                  frame #1 {
                    n550 = local write "Ring 20"(u16 1 ("Ring 2")) -> ()
                    n551 = local write "Ring 19"(u16 0 ("Ring 1")) -> ()
                    n552 = Wait (ms)(milliseconds to wait=u32 100) -> ()  [unwired: 1 out]
                  }
                  frame #2 {
                    n553 = local write "Ring 21"(u16 1 ("Ring 3")) -> ()
                    n554 = local write "Ring 20"(u16 0 ("Ring 2")) -> ()
                  }
                }
              }
            }
          }
          frame 5 {
            n555 = case shown="False" w2709 {
              frame False {
                n556 = flat-sequence {
                  frame #0 {
                    n557 = local write "Ring 19"(u16 2 ("Ring 1")) -> ()
                    n558 = Wait (ms)(milliseconds to wait=u32 100) -> ()  [unwired: 1 out]
                  }
                  frame #1 {
                    n559 = local write "Ring 20"(u16 2 ("Ring 2")) -> ()
                    n560 = local write "Ring 19"(u16 0 ("Ring 1")) -> ()
                  }
                }
              }
              frame True {
                n561 = flat-sequence {
                  frame #0 {
                    n562 = local write "Ring 19"(u16 1 ("Ring 1")) -> ()
                    n563 = Wait (ms)(milliseconds to wait=u32 100) -> ()  [unwired: 1 out]
                  }
                  frame #1 {
                    n564 = local write "Ring 20"(u16 1 ("Ring 2")) -> ()
                    n565 = local write "Ring 19"(u16 0 ("Ring 1")) -> ()
                  }
                }
              }
            }
          }
          frame 6 {
            n566 = case shown="False" w2719 {
              frame False {
                n567 = flat-sequence {
                  frame #0 {
                    n568 = local write "Ring 19"(u16 2 ("Ring 1")) -> ()
                  }
                }
              }
              frame True {
                n569 = flat-sequence {
                  frame #0 {
                    n570 = local write "Ring 19"(u16 1 ("Ring 1")) -> ()
                  }
                }
              }
            }
          }
        }
      }
      event "col5": Mouse Down {
        n571 = event-data() -> ()  [unwired: 1 in, 8 out]
        n572 = Add(x=w2733, y=1) -> (x+y=w2732:i32)
        n573 = Not(x=w2729) -> (.not. x?=w2730:bool)
        n574 = case shown="6" w2732 {
          selector: w2732 -> [w2735 w2737 w2771 w2799 w2821 w2837 w2847]
          tunnel: [w2735 w2737 w2771 w2799 w2821 w2837 w2847] -> w2731
          tunnel: w2729 -> [_ w2736 w2770 w2798 w2820 w2836 w2846]
          frame 0, Default {
          }
          frame 1 {
            n575 = case shown="False" w2736 {
              frame False {
                n576 = flat-sequence {
                  frame #0 {
                    n577 = local write "Ring 25"(u16 2 ("Ring 1")) -> ()
                    n578 = Wait (ms)(milliseconds to wait=u32 100) -> ()  [unwired: 1 out]
                  }
                  frame #1 {
                    n579 = local write "Ring 26"(u16 2 ("Ring 2")) -> ()
                    n580 = local write "Ring 25"(u16 0 ("Ring 1")) -> ()
                    n581 = Wait (ms)(milliseconds to wait=u32 100) -> ()  [unwired: 1 out]
                  }
                  frame #2 {
                    n582 = local write "Ring 27"(u16 2 ("Ring 3")) -> ()
                    n583 = local write "Ring 26"(u16 0 ("Ring 2")) -> ()
                    n584 = Wait (ms)(milliseconds to wait=u32 100) -> ()  [unwired: 1 out]
                  }
                  frame #3 {
                    n585 = local write "Ring 28"(u16 2 ("Ring 4")) -> ()
                    n586 = local write "Ring 27"(u16 0 ("Ring 3")) -> ()
                    n587 = Wait (ms)(milliseconds to wait=u32 100) -> ()  [unwired: 1 out]
                  }
                  frame #4 {
                    n588 = local write "Ring 29"(u16 2 ("Ring 5")) -> ()
                    n589 = local write "Ring 28"(u16 0 ("Ring 4")) -> ()
                    n590 = Wait (ms)(milliseconds to wait=u32 100) -> ()  [unwired: 1 out]
                  }
                  frame #5 {
                    n591 = local write "Ring 30"(u16 2 ("Ring 6")) -> ()
                    n592 = local write "Ring 29"(u16 0 ("Ring 5")) -> ()
                  }
                }
              }
              frame True {
                n593 = flat-sequence {
                  frame #0 {
                    n594 = local write "Ring 25"(u16 1 ("Ring 1")) -> ()
                    n595 = Wait (ms)(milliseconds to wait=u32 100) -> ()  [unwired: 1 out]
                  }
                  frame #1 {
                    n596 = local write "Ring 26"(u16 1 ("Ring 2")) -> ()
                    n597 = local write "Ring 25"(u16 0 ("Ring 1")) -> ()
                    n598 = Wait (ms)(milliseconds to wait=u32 100) -> ()  [unwired: 1 out]
                  }
                  frame #2 {
                    n599 = local write "Ring 27"(u16 1 ("Ring 3")) -> ()
                    n600 = local write "Ring 26"(u16 0 ("Ring 2")) -> ()
                    n601 = Wait (ms)(milliseconds to wait=u32 100) -> ()  [unwired: 1 out]
                  }
                  frame #3 {
                    n602 = local write "Ring 28"(u16 1 ("Ring 4")) -> ()
                    n603 = local write "Ring 27"(u16 0 ("Ring 3")) -> ()
                    n604 = Wait (ms)(milliseconds to wait=u32 100) -> ()  [unwired: 1 out]
                  }
                  frame #4 {
                    n605 = local write "Ring 29"(u16 1 ("Ring 5")) -> ()
                    n606 = local write "Ring 28"(u16 0 ("Ring 4")) -> ()
                    n607 = Wait (ms)(milliseconds to wait=u32 100) -> ()  [unwired: 1 out]
                  }
                  frame #5 {
                    n608 = local write "Ring 30"(u16 1 ("Ring 6")) -> ()
                    n609 = local write "Ring 29"(u16 0 ("Ring 5")) -> ()
                  }
                }
              }
            }
          }
          frame 2 {
            n610 = case shown="False" w2770 {
              frame False {
                n611 = flat-sequence {
                  frame #0 {
                    n612 = local write "Ring 25"(u16 2 ("Ring 1")) -> ()
                    n613 = Wait (ms)(milliseconds to wait=u32 100) -> ()  [unwired: 1 out]
                  }
                  frame #1 {
                    n614 = local write "Ring 26"(u16 2 ("Ring 2")) -> ()
                    n615 = local write "Ring 25"(u16 0 ("Ring 1")) -> ()
                    n616 = Wait (ms)(milliseconds to wait=u32 100) -> ()  [unwired: 1 out]
                  }
                  frame #2 {
                    n617 = local write "Ring 27"(u16 2 ("Ring 3")) -> ()
                    n618 = local write "Ring 26"(u16 0 ("Ring 2")) -> ()
                    n619 = Wait (ms)(milliseconds to wait=u32 100) -> ()  [unwired: 1 out]
                  }
                  frame #3 {
                    n620 = local write "Ring 28"(u16 2 ("Ring 4")) -> ()
                    n621 = local write "Ring 27"(u16 0 ("Ring 3")) -> ()
                    n622 = Wait (ms)(milliseconds to wait=u32 100) -> ()  [unwired: 1 out]
                  }
                  frame #4 {
                    n623 = local write "Ring 29"(u16 2 ("Ring 5")) -> ()
                    n624 = local write "Ring 28"(u16 0 ("Ring 4")) -> ()
                  }
                }
              }
              frame True {
                n625 = flat-sequence {
                  frame #0 {
                    n626 = local write "Ring 25"(u16 1 ("Ring 1")) -> ()
                    n627 = Wait (ms)(milliseconds to wait=u32 100) -> ()  [unwired: 1 out]
                  }
                  frame #1 {
                    n628 = local write "Ring 26"(u16 1 ("Ring 2")) -> ()
                    n629 = local write "Ring 25"(u16 0 ("Ring 1")) -> ()
                    n630 = Wait (ms)(milliseconds to wait=u32 100) -> ()  [unwired: 1 out]
                  }
                  frame #2 {
                    n631 = local write "Ring 27"(u16 1 ("Ring 3")) -> ()
                    n632 = local write "Ring 26"(u16 0 ("Ring 2")) -> ()
                    n633 = Wait (ms)(milliseconds to wait=u32 100) -> ()  [unwired: 1 out]
                  }
                  frame #3 {
                    n634 = local write "Ring 28"(u16 1 ("Ring 4")) -> ()
                    n635 = local write "Ring 27"(u16 0 ("Ring 3")) -> ()
                    n636 = Wait (ms)(milliseconds to wait=u32 100) -> ()  [unwired: 1 out]
                  }
                  frame #4 {
                    n637 = local write "Ring 29"(u16 1 ("Ring 5")) -> ()
                    n638 = local write "Ring 28"(u16 0 ("Ring 4")) -> ()
                  }
                }
              }
            }
          }
          frame 3 {
            n639 = case shown="False" w2798 {
              frame False {
                n640 = flat-sequence {
                  frame #0 {
                    n641 = local write "Ring 25"(u16 2 ("Ring 1")) -> ()
                    n642 = Wait (ms)(milliseconds to wait=u32 100) -> ()  [unwired: 1 out]
                  }
                  frame #1 {
                    n643 = local write "Ring 26"(u16 2 ("Ring 2")) -> ()
                    n644 = local write "Ring 25"(u16 0 ("Ring 1")) -> ()
                    n645 = Wait (ms)(milliseconds to wait=u32 100) -> ()  [unwired: 1 out]
                  }
                  frame #2 {
                    n646 = local write "Ring 27"(u16 2 ("Ring 3")) -> ()
                    n647 = local write "Ring 26"(u16 0 ("Ring 2")) -> ()
                    n648 = Wait (ms)(milliseconds to wait=u32 100) -> ()  [unwired: 1 out]
                  }
                  frame #3 {
                    n649 = local write "Ring 28"(u16 2 ("Ring 4")) -> ()
                    n650 = local write "Ring 27"(u16 0 ("Ring 3")) -> ()
                  }
                }
              }
              frame True {
                n651 = flat-sequence {
                  frame #0 {
                    n652 = local write "Ring 25"(u16 1 ("Ring 1")) -> ()
                    n653 = Wait (ms)(milliseconds to wait=u32 100) -> ()  [unwired: 1 out]
                  }
                  frame #1 {
                    n654 = local write "Ring 26"(u16 1 ("Ring 2")) -> ()
                    n655 = local write "Ring 25"(u16 0 ("Ring 1")) -> ()
                    n656 = Wait (ms)(milliseconds to wait=u32 100) -> ()  [unwired: 1 out]
                  }
                  frame #2 {
                    n657 = local write "Ring 27"(u16 1 ("Ring 3")) -> ()
                    n658 = local write "Ring 26"(u16 0 ("Ring 2")) -> ()
                    n659 = Wait (ms)(milliseconds to wait=u32 100) -> ()  [unwired: 1 out]
                  }
                  frame #3 {
                    n660 = local write "Ring 28"(u16 1 ("Ring 4")) -> ()
                    n661 = local write "Ring 27"(u16 0 ("Ring 3")) -> ()
                  }
                }
              }
            }
          }
          frame 4 {
            n662 = case shown="False" w2820 {
              frame False {
                n663 = flat-sequence {
                  frame #0 {
                    n664 = local write "Ring 25"(u16 2 ("Ring 1")) -> ()
                    n665 = Wait (ms)(milliseconds to wait=u32 100) -> ()  [unwired: 1 out]
                  }
                  frame #1 {
                    n666 = local write "Ring 26"(u16 2 ("Ring 2")) -> ()
                    n667 = local write "Ring 25"(u16 0 ("Ring 1")) -> ()
                    n668 = Wait (ms)(milliseconds to wait=u32 100) -> ()  [unwired: 1 out]
                  }
                  frame #2 {
                    n669 = local write "Ring 27"(u16 2 ("Ring 3")) -> ()
                    n670 = local write "Ring 26"(u16 0 ("Ring 2")) -> ()
                  }
                }
              }
              frame True {
                n671 = flat-sequence {
                  frame #0 {
                    n672 = local write "Ring 25"(u16 1 ("Ring 1")) -> ()
                    n673 = Wait (ms)(milliseconds to wait=u32 100) -> ()  [unwired: 1 out]
                  }
                  frame #1 {
                    n674 = local write "Ring 26"(u16 1 ("Ring 2")) -> ()
                    n675 = local write "Ring 25"(u16 0 ("Ring 1")) -> ()
                    n676 = Wait (ms)(milliseconds to wait=u32 100) -> ()  [unwired: 1 out]
                  }
                  frame #2 {
                    n677 = local write "Ring 27"(u16 1 ("Ring 3")) -> ()
                    n678 = local write "Ring 26"(u16 0 ("Ring 2")) -> ()
                  }
                }
              }
            }
          }
          frame 5 {
            n679 = case shown="True" w2836 {
              frame False {
                n680 = flat-sequence {
                  frame #0 {
                    n681 = local write "Ring 25"(u16 2 ("Ring 1")) -> ()
                    n682 = Wait (ms)(milliseconds to wait=u32 100) -> ()  [unwired: 1 out]
                  }
                  frame #1 {
                    n683 = local write "Ring 26"(u16 2 ("Ring 2")) -> ()
                    n684 = local write "Ring 25"(u16 0 ("Ring 1")) -> ()
                  }
                }
              }
              frame True {
                n685 = flat-sequence {
                  frame #0 {
                    n686 = local write "Ring 25"(u16 1 ("Ring 1")) -> ()
                    n687 = Wait (ms)(milliseconds to wait=u32 100) -> ()  [unwired: 1 out]
                  }
                  frame #1 {
                    n688 = local write "Ring 26"(u16 1 ("Ring 2")) -> ()
                    n689 = local write "Ring 25"(u16 0 ("Ring 1")) -> ()
                  }
                }
              }
            }
          }
          frame 6 {
            n690 = case shown="True" w2846 {
              frame False {
                n691 = flat-sequence {
                  frame #0 {
                    n692 = local write "Ring 25"(u16 2 ("Ring 1")) -> ()
                  }
                }
              }
              frame True {
                n693 = flat-sequence {
                  frame #0 {
                    n694 = local write "Ring 25"(u16 1 ("Ring 1")) -> ()
                  }
                }
              }
            }
          }
        }
      }
      event "col6": Mouse Down {
        n695 = event-data() -> ()  [unwired: 1 in, 8 out]
        n696 = Add(x=w2860, y=1) -> (x+y=w2859:i32)
        n697 = Not(x=w2857) -> (.not. x?=w2856:bool)
        n698 = case shown="4" w2859 {
          selector: w2859 -> [w2862 w2864 w2898 w2926 w2948 w2964 w2974]
          tunnel: [w2862 w2864 w2898 w2926 w2948 w2964 w2974] -> w2858
          tunnel: w2857 -> [_ w2863 w2897 w2925 w2947 w2963 w2973]
          frame 0, Default {
          }
          frame 1 {
            n699 = case shown="True" w2863 {
              frame False {
                n700 = flat-sequence {
                  frame #0 {
                    n701 = local write "Ring 31"(u16 2 ("Ring 1")) -> ()
                    n702 = Wait (ms)(milliseconds to wait=u32 100) -> ()  [unwired: 1 out]
                  }
                  frame #1 {
                    n703 = local write "Ring 32"(u16 2 ("Ring 2")) -> ()
                    n704 = local write "Ring 31"(u16 0 ("Ring 1")) -> ()
                    n705 = Wait (ms)(milliseconds to wait=u32 100) -> ()  [unwired: 1 out]
                  }
                  frame #2 {
                    n706 = local write "Ring 33"(u16 2 ("Ring 3")) -> ()
                    n707 = local write "Ring 32"(u16 0 ("Ring 2")) -> ()
                    n708 = Wait (ms)(milliseconds to wait=u32 100) -> ()  [unwired: 1 out]
                  }
                  frame #3 {
                    n709 = local write "Ring 34"(u16 2 ("Ring 4")) -> ()
                    n710 = local write "Ring 33"(u16 0 ("Ring 3")) -> ()
                    n711 = Wait (ms)(milliseconds to wait=u32 100) -> ()  [unwired: 1 out]
                  }
                  frame #4 {
                    n712 = local write "Ring 35"(u16 2 ("Ring 5")) -> ()
                    n713 = local write "Ring 34"(u16 0 ("Ring 4")) -> ()
                    n714 = Wait (ms)(milliseconds to wait=u32 100) -> ()  [unwired: 1 out]
                  }
                  frame #5 {
                    n715 = local write "Ring 36"(u16 2 ("Ring 6")) -> ()
                    n716 = local write "Ring 35"(u16 0 ("Ring 5")) -> ()
                  }
                }
              }
              frame True {
                n717 = flat-sequence {
                  frame #0 {
                    n718 = local write "Ring 31"(u16 1 ("Ring 1")) -> ()
                    n719 = Wait (ms)(milliseconds to wait=u32 100) -> ()  [unwired: 1 out]
                  }
                  frame #1 {
                    n720 = local write "Ring 32"(u16 1 ("Ring 2")) -> ()
                    n721 = local write "Ring 31"(u16 0 ("Ring 1")) -> ()
                    n722 = Wait (ms)(milliseconds to wait=u32 100) -> ()  [unwired: 1 out]
                  }
                  frame #2 {
                    n723 = local write "Ring 33"(u16 1 ("Ring 3")) -> ()
                    n724 = local write "Ring 32"(u16 0 ("Ring 2")) -> ()
                    n725 = Wait (ms)(milliseconds to wait=u32 100) -> ()  [unwired: 1 out]
                  }
                  frame #3 {
                    n726 = local write "Ring 34"(u16 1 ("Ring 4")) -> ()
                    n727 = local write "Ring 33"(u16 0 ("Ring 3")) -> ()
                    n728 = Wait (ms)(milliseconds to wait=u32 100) -> ()  [unwired: 1 out]
                  }
                  frame #4 {
                    n729 = local write "Ring 35"(u16 1 ("Ring 5")) -> ()
                    n730 = local write "Ring 34"(u16 0 ("Ring 4")) -> ()
                    n731 = Wait (ms)(milliseconds to wait=u32 100) -> ()  [unwired: 1 out]
                  }
                  frame #5 {
                    n732 = local write "Ring 36"(u16 1 ("Ring 6")) -> ()
                    n733 = local write "Ring 35"(u16 0 ("Ring 5")) -> ()
                  }
                }
              }
            }
          }
          frame 2 {
            n734 = case shown="True" w2897 {
              frame False {
                n735 = flat-sequence {
                  frame #0 {
                    n736 = local write "Ring 31"(u16 2 ("Ring 1")) -> ()
                    n737 = Wait (ms)(milliseconds to wait=u32 100) -> ()  [unwired: 1 out]
                  }
                  frame #1 {
                    n738 = local write "Ring 32"(u16 2 ("Ring 2")) -> ()
                    n739 = local write "Ring 31"(u16 0 ("Ring 1")) -> ()
                    n740 = Wait (ms)(milliseconds to wait=u32 100) -> ()  [unwired: 1 out]
                  }
                  frame #2 {
                    n741 = local write "Ring 33"(u16 2 ("Ring 3")) -> ()
                    n742 = local write "Ring 32"(u16 0 ("Ring 2")) -> ()
                    n743 = Wait (ms)(milliseconds to wait=u32 100) -> ()  [unwired: 1 out]
                  }
                  frame #3 {
                    n744 = local write "Ring 34"(u16 2 ("Ring 4")) -> ()
                    n745 = local write "Ring 33"(u16 0 ("Ring 3")) -> ()
                    n746 = Wait (ms)(milliseconds to wait=u32 100) -> ()  [unwired: 1 out]
                  }
                  frame #4 {
                    n747 = local write "Ring 35"(u16 2 ("Ring 5")) -> ()
                    n748 = local write "Ring 34"(u16 0 ("Ring 4")) -> ()
                  }
                }
              }
              frame True {
                n749 = flat-sequence {
                  frame #0 {
                    n750 = local write "Ring 31"(u16 1 ("Ring 1")) -> ()
                    n751 = Wait (ms)(milliseconds to wait=u32 100) -> ()  [unwired: 1 out]
                  }
                  frame #1 {
                    n752 = local write "Ring 32"(u16 1 ("Ring 2")) -> ()
                    n753 = local write "Ring 31"(u16 0 ("Ring 1")) -> ()
                    n754 = Wait (ms)(milliseconds to wait=u32 100) -> ()  [unwired: 1 out]
                  }
                  frame #2 {
                    n755 = local write "Ring 33"(u16 1 ("Ring 3")) -> ()
                    n756 = local write "Ring 32"(u16 0 ("Ring 2")) -> ()
                    n757 = Wait (ms)(milliseconds to wait=u32 100) -> ()  [unwired: 1 out]
                  }
                  frame #3 {
                    n758 = local write "Ring 34"(u16 1 ("Ring 4")) -> ()
                    n759 = local write "Ring 33"(u16 0 ("Ring 3")) -> ()
                    n760 = Wait (ms)(milliseconds to wait=u32 100) -> ()  [unwired: 1 out]
                  }
                  frame #4 {
                    n761 = local write "Ring 35"(u16 1 ("Ring 5")) -> ()
                    n762 = local write "Ring 34"(u16 0 ("Ring 4")) -> ()
                  }
                }
              }
            }
          }
          frame 3 {
            n763 = case shown="True" w2925 {
              frame False {
                n764 = flat-sequence {
                  frame #0 {
                    n765 = local write "Ring 31"(u16 2 ("Ring 1")) -> ()
                    n766 = Wait (ms)(milliseconds to wait=u32 100) -> ()  [unwired: 1 out]
                  }
                  frame #1 {
                    n767 = local write "Ring 32"(u16 2 ("Ring 2")) -> ()
                    n768 = local write "Ring 31"(u16 0 ("Ring 1")) -> ()
                    n769 = Wait (ms)(milliseconds to wait=u32 100) -> ()  [unwired: 1 out]
                  }
                  frame #2 {
                    n770 = local write "Ring 33"(u16 2 ("Ring 3")) -> ()
                    n771 = local write "Ring 32"(u16 0 ("Ring 2")) -> ()
                    n772 = Wait (ms)(milliseconds to wait=u32 100) -> ()  [unwired: 1 out]
                  }
                  frame #3 {
                    n773 = local write "Ring 34"(u16 2 ("Ring 4")) -> ()
                    n774 = local write "Ring 33"(u16 0 ("Ring 3")) -> ()
                  }
                }
              }
              frame True {
                n775 = flat-sequence {
                  frame #0 {
                    n776 = local write "Ring 31"(u16 1 ("Ring 1")) -> ()
                    n777 = Wait (ms)(milliseconds to wait=u32 100) -> ()  [unwired: 1 out]
                  }
                  frame #1 {
                    n778 = local write "Ring 32"(u16 1 ("Ring 2")) -> ()
                    n779 = local write "Ring 31"(u16 0 ("Ring 1")) -> ()
                    n780 = Wait (ms)(milliseconds to wait=u32 100) -> ()  [unwired: 1 out]
                  }
                  frame #2 {
                    n781 = local write "Ring 33"(u16 1 ("Ring 3")) -> ()
                    n782 = local write "Ring 32"(u16 0 ("Ring 2")) -> ()
                    n783 = Wait (ms)(milliseconds to wait=u32 100) -> ()  [unwired: 1 out]
                  }
                  frame #3 {
                    n784 = local write "Ring 34"(u16 1 ("Ring 4")) -> ()
                    n785 = local write "Ring 33"(u16 0 ("Ring 3")) -> ()
                  }
                }
              }
            }
          }
          frame 4 {
            n786 = case shown="False" w2947 {
              frame False {
                n787 = flat-sequence {
                  frame #0 {
                    n788 = local write "Ring 31"(u16 2 ("Ring 1")) -> ()
                    n789 = Wait (ms)(milliseconds to wait=u32 100) -> ()  [unwired: 1 out]
                  }
                  frame #1 {
                    n790 = local write "Ring 32"(u16 2 ("Ring 2")) -> ()
                    n791 = local write "Ring 31"(u16 0 ("Ring 1")) -> ()
                    n792 = Wait (ms)(milliseconds to wait=u32 100) -> ()  [unwired: 1 out]
                  }
                  frame #2 {
                    n793 = local write "Ring 33"(u16 2 ("Ring 3")) -> ()
                    n794 = local write "Ring 32"(u16 0 ("Ring 2")) -> ()
                  }
                }
              }
              frame True {
                n795 = flat-sequence {
                  frame #0 {
                    n796 = local write "Ring 31"(u16 1 ("Ring 1")) -> ()
                    n797 = Wait (ms)(milliseconds to wait=u32 100) -> ()  [unwired: 1 out]
                  }
                  frame #1 {
                    n798 = local write "Ring 32"(u16 1 ("Ring 2")) -> ()
                    n799 = local write "Ring 31"(u16 0 ("Ring 1")) -> ()
                    n800 = Wait (ms)(milliseconds to wait=u32 100) -> ()  [unwired: 1 out]
                  }
                  frame #2 {
                    n801 = local write "Ring 33"(u16 1 ("Ring 3")) -> ()
                    n802 = local write "Ring 32"(u16 0 ("Ring 2")) -> ()
                  }
                }
              }
            }
          }
          frame 5 {
            n803 = case shown="False" w2963 {
              frame False {
                n804 = flat-sequence {
                  frame #0 {
                    n805 = local write "Ring 31"(u16 2 ("Ring 1")) -> ()
                    n806 = Wait (ms)(milliseconds to wait=u32 100) -> ()  [unwired: 1 out]
                  }
                  frame #1 {
                    n807 = local write "Ring 32"(u16 2 ("Ring 2")) -> ()
                    n808 = local write "Ring 31"(u16 0 ("Ring 1")) -> ()
                  }
                }
              }
              frame True {
                n809 = flat-sequence {
                  frame #0 {
                    n810 = local write "Ring 31"(u16 1 ("Ring 1")) -> ()
                    n811 = Wait (ms)(milliseconds to wait=u32 100) -> ()  [unwired: 1 out]
                  }
                  frame #1 {
                    n812 = local write "Ring 32"(u16 1 ("Ring 2")) -> ()
                    n813 = local write "Ring 31"(u16 0 ("Ring 1")) -> ()
                  }
                }
              }
            }
          }
          frame 6 {
            n814 = case shown="False" w2973 {
              frame False {
                n815 = flat-sequence {
                  frame #0 {
                    n816 = local write "Ring 31"(u16 2 ("Ring 1")) -> ()
                  }
                }
              }
              frame True {
                n817 = flat-sequence {
                  frame #0 {
                    n818 = local write "Ring 31"(u16 1 ("Ring 1")) -> ()
                  }
                }
              }
            }
          }
        }
      }
      event "col7": Mouse Down {
        n819 = event-data() -> ()  [unwired: 1 in, 8 out]
        n820 = Add(x=w2987, y=1) -> (x+y=w2986:i32)
        n821 = Not(x=w2977) -> (.not. x?=w2978:bool)
        n822 = case shown="1" w2986 {
          selector: w2986 -> [w2989 w2991 w3025 w3053 w3075 w3091 w3101]
          tunnel: [w2989 w2991 w3025 w3053 w3075 w3091 w3101] -> w2985
          tunnel: w2977 -> [_ w2990 w3024 w3052 w3074 w3090 w3100]
          frame 0, Default {
          }
          frame 1 {
            n823 = case shown="False" w2990 {
              frame False {
                n824 = flat-sequence {
                  frame #0 {
                    n825 = local write "Ring 37"(u16 2 ("Ring 1")) -> ()
                    n826 = Wait (ms)(milliseconds to wait=u32 100) -> ()  [unwired: 1 out]
                  }
                  frame #1 {
                    n827 = local write "Ring 38"(u16 2 ("Ring 2")) -> ()
                    n828 = local write "Ring 37"(u16 0 ("Ring 1")) -> ()
                    n829 = Wait (ms)(milliseconds to wait=u32 100) -> ()  [unwired: 1 out]
                  }
                  frame #2 {
                    n830 = local write "Ring 39"(u16 2 ("Ring 3")) -> ()
                    n831 = local write "Ring 38"(u16 0 ("Ring 2")) -> ()
                    n832 = Wait (ms)(milliseconds to wait=u32 100) -> ()  [unwired: 1 out]
                  }
                  frame #3 {
                    n833 = local write "Ring 40"(u16 2 ("Ring 4")) -> ()
                    n834 = local write "Ring 39"(u16 0 ("Ring 3")) -> ()
                    n835 = Wait (ms)(milliseconds to wait=u32 100) -> ()  [unwired: 1 out]
                  }
                  frame #4 {
                    n836 = local write "Ring 41"(u16 2 ("Ring 5")) -> ()
                    n837 = local write "Ring 40"(u16 0 ("Ring 4")) -> ()
                    n838 = Wait (ms)(milliseconds to wait=u32 100) -> ()  [unwired: 1 out]
                  }
                  frame #5 {
                    n839 = local write "Ring 42"(u16 2 ("Ring 6")) -> ()
                    n840 = local write "Ring 41"(u16 0 ("Ring 5")) -> ()
                  }
                }
              }
              frame True {
                n841 = flat-sequence {
                  frame #0 {
                    n842 = local write "Ring 37"(u16 1 ("Ring 1")) -> ()
                    n843 = Wait (ms)(milliseconds to wait=u32 100) -> ()  [unwired: 1 out]
                  }
                  frame #1 {
                    n844 = local write "Ring 38"(u16 1 ("Ring 2")) -> ()
                    n845 = local write "Ring 37"(u16 0 ("Ring 1")) -> ()
                    n846 = Wait (ms)(milliseconds to wait=u32 100) -> ()  [unwired: 1 out]
                  }
                  frame #2 {
                    n847 = local write "Ring 39"(u16 1 ("Ring 3")) -> ()
                    n848 = local write "Ring 38"(u16 0 ("Ring 2")) -> ()
                    n849 = Wait (ms)(milliseconds to wait=u32 100) -> ()  [unwired: 1 out]
                  }
                  frame #3 {
                    n850 = local write "Ring 40"(u16 1 ("Ring 4")) -> ()
                    n851 = local write "Ring 39"(u16 0 ("Ring 3")) -> ()
                    n852 = Wait (ms)(milliseconds to wait=u32 100) -> ()  [unwired: 1 out]
                  }
                  frame #4 {
                    n853 = local write "Ring 41"(u16 1 ("Ring 5")) -> ()
                    n854 = local write "Ring 40"(u16 0 ("Ring 4")) -> ()
                    n855 = Wait (ms)(milliseconds to wait=u32 100) -> ()  [unwired: 1 out]
                  }
                  frame #5 {
                    n856 = local write "Ring 42"(u16 1 ("Ring 6")) -> ()
                    n857 = local write "Ring 41"(u16 0 ("Ring 5")) -> ()
                  }
                }
              }
            }
          }
          frame 2 {
            n858 = case shown="False" w3024 {
              frame False {
                n859 = flat-sequence {
                  frame #0 {
                    n860 = local write "Ring 37"(u16 2 ("Ring 1")) -> ()
                    n861 = Wait (ms)(milliseconds to wait=u32 100) -> ()  [unwired: 1 out]
                  }
                  frame #1 {
                    n862 = local write "Ring 38"(u16 2 ("Ring 2")) -> ()
                    n863 = local write "Ring 37"(u16 0 ("Ring 1")) -> ()
                    n864 = Wait (ms)(milliseconds to wait=u32 100) -> ()  [unwired: 1 out]
                  }
                  frame #2 {
                    n865 = local write "Ring 39"(u16 2 ("Ring 3")) -> ()
                    n866 = local write "Ring 38"(u16 0 ("Ring 2")) -> ()
                    n867 = Wait (ms)(milliseconds to wait=u32 100) -> ()  [unwired: 1 out]
                  }
                  frame #3 {
                    n868 = local write "Ring 40"(u16 2 ("Ring 4")) -> ()
                    n869 = local write "Ring 39"(u16 0 ("Ring 3")) -> ()
                    n870 = Wait (ms)(milliseconds to wait=u32 100) -> ()  [unwired: 1 out]
                  }
                  frame #4 {
                    n871 = local write "Ring 41"(u16 2 ("Ring 5")) -> ()
                    n872 = local write "Ring 40"(u16 0 ("Ring 4")) -> ()
                  }
                }
              }
              frame True {
                n873 = flat-sequence {
                  frame #0 {
                    n874 = local write "Ring 37"(u16 1 ("Ring 1")) -> ()
                    n875 = Wait (ms)(milliseconds to wait=u32 100) -> ()  [unwired: 1 out]
                  }
                  frame #1 {
                    n876 = local write "Ring 38"(u16 1 ("Ring 2")) -> ()
                    n877 = local write "Ring 37"(u16 0 ("Ring 1")) -> ()
                    n878 = Wait (ms)(milliseconds to wait=u32 100) -> ()  [unwired: 1 out]
                  }
                  frame #2 {
                    n879 = local write "Ring 39"(u16 1 ("Ring 3")) -> ()
                    n880 = local write "Ring 38"(u16 0 ("Ring 2")) -> ()
                    n881 = Wait (ms)(milliseconds to wait=u32 100) -> ()  [unwired: 1 out]
                  }
                  frame #3 {
                    n882 = local write "Ring 40"(u16 1 ("Ring 4")) -> ()
                    n883 = local write "Ring 39"(u16 0 ("Ring 3")) -> ()
                    n884 = Wait (ms)(milliseconds to wait=u32 100) -> ()  [unwired: 1 out]
                  }
                  frame #4 {
                    n885 = local write "Ring 41"(u16 1 ("Ring 5")) -> ()
                    n886 = local write "Ring 40"(u16 0 ("Ring 4")) -> ()
                  }
                }
              }
            }
          }
          frame 3 {
            n887 = case shown="False" w3052 {
              frame False {
                n888 = flat-sequence {
                  frame #0 {
                    n889 = local write "Ring 37"(u16 2 ("Ring 1")) -> ()
                    n890 = Wait (ms)(milliseconds to wait=u32 100) -> ()  [unwired: 1 out]
                  }
                  frame #1 {
                    n891 = local write "Ring 38"(u16 2 ("Ring 2")) -> ()
                    n892 = local write "Ring 37"(u16 0 ("Ring 1")) -> ()
                    n893 = Wait (ms)(milliseconds to wait=u32 100) -> ()  [unwired: 1 out]
                  }
                  frame #2 {
                    n894 = local write "Ring 39"(u16 2 ("Ring 3")) -> ()
                    n895 = local write "Ring 38"(u16 0 ("Ring 2")) -> ()
                    n896 = Wait (ms)(milliseconds to wait=u32 100) -> ()  [unwired: 1 out]
                  }
                  frame #3 {
                    n897 = local write "Ring 40"(u16 2 ("Ring 4")) -> ()
                    n898 = local write "Ring 39"(u16 0 ("Ring 3")) -> ()
                  }
                }
              }
              frame True {
                n899 = flat-sequence {
                  frame #0 {
                    n900 = local write "Ring 37"(u16 1 ("Ring 1")) -> ()
                    n901 = Wait (ms)(milliseconds to wait=u32 100) -> ()  [unwired: 1 out]
                  }
                  frame #1 {
                    n902 = local write "Ring 38"(u16 1 ("Ring 2")) -> ()
                    n903 = local write "Ring 37"(u16 0 ("Ring 1")) -> ()
                    n904 = Wait (ms)(milliseconds to wait=u32 100) -> ()  [unwired: 1 out]
                  }
                  frame #2 {
                    n905 = local write "Ring 39"(u16 1 ("Ring 3")) -> ()
                    n906 = local write "Ring 38"(u16 0 ("Ring 2")) -> ()
                    n907 = Wait (ms)(milliseconds to wait=u32 100) -> ()  [unwired: 1 out]
                  }
                  frame #3 {
                    n908 = local write "Ring 40"(u16 1 ("Ring 4")) -> ()
                    n909 = local write "Ring 39"(u16 0 ("Ring 3")) -> ()
                  }
                }
              }
            }
          }
          frame 4 {
            n910 = case shown="True" w3074 {
              frame False {
                n911 = flat-sequence {
                  frame #0 {
                    n912 = local write "Ring 37"(u16 2 ("Ring 1")) -> ()
                    n913 = Wait (ms)(milliseconds to wait=u32 100) -> ()  [unwired: 1 out]
                  }
                  frame #1 {
                    n914 = local write "Ring 38"(u16 2 ("Ring 2")) -> ()
                    n915 = local write "Ring 37"(u16 0 ("Ring 1")) -> ()
                    n916 = Wait (ms)(milliseconds to wait=u32 100) -> ()  [unwired: 1 out]
                  }
                  frame #2 {
                    n917 = local write "Ring 39"(u16 2 ("Ring 3")) -> ()
                    n918 = local write "Ring 38"(u16 0 ("Ring 2")) -> ()
                  }
                }
              }
              frame True {
                n919 = flat-sequence {
                  frame #0 {
                    n920 = local write "Ring 37"(u16 1 ("Ring 1")) -> ()
                    n921 = Wait (ms)(milliseconds to wait=u32 100) -> ()  [unwired: 1 out]
                  }
                  frame #1 {
                    n922 = local write "Ring 38"(u16 1 ("Ring 2")) -> ()
                    n923 = local write "Ring 37"(u16 0 ("Ring 1")) -> ()
                    n924 = Wait (ms)(milliseconds to wait=u32 100) -> ()  [unwired: 1 out]
                  }
                  frame #2 {
                    n925 = local write "Ring 39"(u16 1 ("Ring 3")) -> ()
                    n926 = local write "Ring 38"(u16 0 ("Ring 2")) -> ()
                  }
                }
              }
            }
          }
          frame 5 {
            n927 = case shown="True" w3090 {
              frame False {
                n928 = flat-sequence {
                  frame #0 {
                    n929 = local write "Ring 37"(u16 2 ("Ring 1")) -> ()
                    n930 = Wait (ms)(milliseconds to wait=u32 100) -> ()  [unwired: 1 out]
                  }
                  frame #1 {
                    n931 = local write "Ring 38"(u16 2 ("Ring 2")) -> ()
                    n932 = local write "Ring 37"(u16 0 ("Ring 1")) -> ()
                  }
                }
              }
              frame True {
                n933 = flat-sequence {
                  frame #0 {
                    n934 = local write "Ring 37"(u16 1 ("Ring 1")) -> ()
                    n935 = Wait (ms)(milliseconds to wait=u32 100) -> ()  [unwired: 1 out]
                  }
                  frame #1 {
                    n936 = local write "Ring 38"(u16 1 ("Ring 2")) -> ()
                    n937 = local write "Ring 37"(u16 0 ("Ring 1")) -> ()
                  }
                }
              }
            }
          }
          frame 6 {
            n938 = case shown="True" w3100 {
              frame False {
                n939 = flat-sequence {
                  frame #0 {
                    n940 = local write "Ring 37"(u16 2 ("Ring 1")) -> ()
                  }
                }
              }
              frame True {
                n941 = flat-sequence {
                  frame #0 {
                    n942 = local write "Ring 37"(u16 1 ("Ring 1")) -> ()
                  }
                }
              }
            }
          }
        }
      }
      event "Restet Marcador": Value Change {
        n943 = event-data() -> ()  [unwired: 1 in, 6 out]
        n944 = property on="Player Verde" class="DigNum (strict)"("Value"=0.0 ("Player Verde")) -> ()  [unwired: 2 in, 2 out]
        n945 = property on="Player Rojo" class="DigNum (strict)"("Value"=0.0 ("Player Rojo")) -> ()  [unwired: 2 in, 2 out]
      }
      event "Ring 1", "Ring 2", "Ring 3", "Ring 4", "Ring 5", "Ring 6", "Ring 7", "Ring 8", "Ring 9", "Ring 10", "Ring 11", "Ring 12", "Ring 13", "Ring 14", "Ring 15", "Ring 16", "Ring 17", "Ring 18", "Ring 19", "Ring 20", "Ring 21", "Ring 22", "Ring 23", "Ring 24", "Ring 25", "Ring 26", "Ring 27", "Ring 28", "Ring 29", "Ring 30", "Ring 31", "Ring 32", "Ring 33", "Ring 34", "Ring 35", "Ring 36", "Ring 37", "Ring 38", "Ring 39", "Ring 40", "Ring 41", "Ring 42": Mouse Down? {
        n946 = event-data() -> ()  [unwired: 1 in, 8 out]
        n947 = event-data("Discard?"=TRUE) -> ()  [unwired: 4 in, 1 out]
      }
      event "OK Button": Value Change {
        w3122 = u16 0 ("Ring 42")
        w3121 = u16 0 ("Ring 36")
        w3120 = u16 0 ("Ring 30")
        w3119 = u16 0 ("Ring 24")
        w3118 = u16 0 ("Ring 18")
        w3117 = u16 0 ("Ring 12")
        w3116 = 0
        n948 = event-data() -> ()  [unwired: 1 in, 6 out]
        n949 = local write "Ring 6"(w3116) -> ()
        n950 = local write "Ring 5"(w3116) -> ()
        n951 = local write "Ring 4"(w3116) -> ()
        n952 = local write "Ring 3"(w3116) -> ()
        n953 = local write "Ring 2"(w3116) -> ()
        n954 = local write "Ring 1"(w3116) -> ()
        n955 = local write "Ring 42"(w3122) -> ()
        n956 = local write "Ring 41"(w3122) -> ()
        n957 = local write "Ring 40"(w3122) -> ()
        n958 = local write "Ring 39"(w3122) -> ()
        n959 = local write "Ring 38"(w3122) -> ()
        n960 = local write "Ring 37"(w3122) -> ()
        n961 = local write "Ring 36"(w3121) -> ()
        n962 = local write "Ring 35"(w3121) -> ()
        n963 = local write "Ring 34"(w3121) -> ()
        n964 = local write "Ring 33"(w3121) -> ()
        n965 = local write "Ring 32"(w3121) -> ()
        n966 = local write "Ring 31"(w3121) -> ()
        n967 = local write "Ring 30"(w3120) -> ()
        n968 = local write "Ring 29"(w3120) -> ()
        n969 = local write "Ring 28"(w3120) -> ()
        n970 = local write "Ring 27"(w3120) -> ()
        n971 = local write "Ring 26"(w3120) -> ()
        n972 = local write "Ring 25"(w3120) -> ()
        n973 = local write "Ring 24"(w3119) -> ()
        n974 = local write "Ring 23"(w3119) -> ()
        n975 = local write "Ring 22"(w3119) -> ()
        n976 = local write "Ring 21"(w3119) -> ()
        n977 = local write "Ring 20"(w3119) -> ()
        n978 = local write "Ring 19"(w3119) -> ()
        n979 = local write "Ring 18"(w3118) -> ()
        n980 = local write "Ring 17"(w3118) -> ()
        n981 = local write "Ring 16"(w3118) -> ()
        n982 = local write "Ring 15"(w3118) -> ()
        n983 = local write "Ring 14"(w3118) -> ()
        n984 = local write "Ring 13"(w3118) -> ()
        n985 = local write "Ring 11"(w3117) -> ()
        n986 = local write "Ring 10"(w3117) -> ()
        n987 = local write "Ring 12"(w3117) -> ()
        n988 = local write "Ring 9"(w3117) -> ()
        n989 = local write "Ring 8"(w3117) -> ()
        n990 = local write "Ring 7"(w3117) -> ()
        n991 = local read "verde"() -> (w3115:bool)
      }
    }
    n992 = Equal?(x=w2154, y=u16 1) -> (x = y?=w2155:bool)
    n993 = Equal?(x=w2152, y=u16 1) -> (x = y?=w2156:bool)
    n994 = Equal?(x=w2150, y=u16 1) -> (x = y?=w2157:bool)
    n995 = Equal?(x=w2148, y=u16 1) -> (x = y?=w2158:bool)
    n996 = Equal?(x=w2167, y=u16 1) -> (x = y?=w2163:bool)
    n997 = Equal?(x=w2168, y=u16 1) -> (x = y?=w2164:bool)
    n998 = Equal?(x=w2169, y=u16 1) -> (x = y?=w2165:bool)
    n999 = Equal?(x=w2170, y=u16 1) -> (x = y?=w2166:bool)
    n1000 = Equal?(x=w2137, y=u16 1) -> (x = y?=w2141:bool)
    n1001 = Equal?(x=w2134, y=u16 1) -> (x = y?=w2140:bool)
    n1002 = Equal?(x=w2135, y=u16 1) -> (x = y?=w2139:bool)
    n1003 = Equal?(x=w2136, y=u16 1) -> (x = y?=w2138:bool)
    n1004 = Equal?(x=w1578, y=u16 1) -> (x = y?=w1594:bool)
    n1005 = Equal?(x=w1577, y=u16 1) -> (x = y?=w1593:bool)
    n1006 = Equal?(x=w1576, y=u16 1) -> (x = y?=w1592:bool)
    n1007 = Equal?(x=w1575, y=u16 1) -> (x = y?=w1591:bool)
    n1008 = Equal?(x=w1582, y=u16 1) -> (x = y?=w1602:bool)
    n1009 = Equal?(x=w1581, y=u16 1) -> (x = y?=w1601:bool)
    n1010 = Equal?(x=w1580, y=u16 1) -> (x = y?=w1600:bool)
    n1011 = Equal?(x=w1579, y=u16 1) -> (x = y?=w1599:bool)
    n1012 = Equal?(x=w1586, y=u16 1) -> (x = y?=w1610:bool)
    n1013 = Equal?(x=w1585, y=u16 1) -> (x = y?=w1609:bool)
    n1014 = Equal?(x=w1584, y=u16 1) -> (x = y?=w1608:bool)
    n1015 = Equal?(x=w1583, y=u16 1) -> (x = y?=w1607:bool)
    n1016 = Equal?(x=w1590, y=u16 1) -> (x = y?=w1618:bool)
    n1017 = Equal?(x=w1589, y=u16 1) -> (x = y?=w1617:bool)
    n1018 = Equal?(x=w1588, y=u16 1) -> (x = y?=w1616:bool)
    n1019 = Equal?(x=w1587, y=u16 1) -> (x = y?=w1615:bool)
    n1020 = Compound Arithmetic op=AND(w2155, w2156, w2157, w2158) -> (w1917:bool)
    n1021 = Compound Arithmetic op=AND(w2163, w2164, w2165, w2166) -> (w1916:bool)
    n1022 = Compound Arithmetic op=AND(w2141, w2140, w2139, w2138) -> (w1915:bool)
    n1023 = Compound Arithmetic op=AND(w1618, w1617, w1616, w1615) -> (w1332:bool)
    n1024 = Compound Arithmetic op=AND(w1602, w1601, w1600, w1599) -> (w1334:bool)
    n1025 = Compound Arithmetic op=AND(w1610, w1609, w1608, w1607) -> (w1333:bool)
    n1026 = Compound Arithmetic op=AND(w1594, w1593, w1592, w1591) -> (w1335:bool)
    n1027 = local read "Ring 10"() -> (w2102:u16)
    n1028 = local read "Ring 11"() -> (w2113:u16)
    n1029 = local read "Ring 10"() -> (w2112:u16)
    n1030 = local read "Ring 12"() -> (w2125:u16)
    n1031 = local read "Ring 11"() -> (w2124:u16)
    n1032 = local read "Ring 10"() -> (w2123:u16)
    n1033 = local read "Ring 9"() -> (w2101:u16)
    n1034 = local read "Ring 8"() -> (w2100:u16)
    n1035 = local read "Ring 7"() -> (w2099:u16)
    n1036 = local read "Ring 9"() -> (w2111:u16)
    n1037 = local read "Ring 8"() -> (w2110:u16)
    n1038 = local read "Ring 9"() -> (w2122:u16)
    n1039 = local read "Ring 11"() -> (w1572:u16)
    n1040 = local read "Ring 17"() -> (w1573:u16)
    n1041 = local read "Ring 23"() -> (w1574:u16)
    n1042 = local read "Ring 11"() -> (w1567:u16)
    n1043 = local read "Ring 17"() -> (w1568:u16)
    n1044 = local read "Ring 23"() -> (w1569:u16)
    n1045 = local read "Ring 29"() -> (w1570:u16)
    n1046 = local read "Ring 17"() -> (w1563:u16)
    n1047 = local read "Ring 23"() -> (w1564:u16)
    n1048 = local read "Ring 29"() -> (w1565:u16)
    n1049 = local read "Ring 35"() -> (w1566:u16)
    n1050 = local read "Ring 23"() -> (w1559:u16)
    n1051 = local read "Ring 29"() -> (w1560:u16)
    n1052 = local read "Ring 35"() -> (w1561:u16)
    n1053 = local read "Ring 5"() -> (w1571:u16)
    n1054 = local read "Ring 41"() -> (w1562:u16)
    n1055 = Equal?(x=w2102, y=u16 1) -> (x = y?=w2098:bool)
    n1056 = Equal?(x=w2101, y=u16 1) -> (x = y?=w2105:bool)
    n1057 = Equal?(x=w2100, y=u16 1) -> (x = y?=w2104:bool)
    n1058 = Equal?(x=w2099, y=u16 1) -> (x = y?=w2103:bool)
    n1059 = Equal?(x=w2113, y=u16 1) -> (x = y?=w2118:bool)
    n1060 = Equal?(x=w2112, y=u16 1) -> (x = y?=w2119:bool)
    n1061 = Equal?(x=w2111, y=u16 1) -> (x = y?=w2120:bool)
    n1062 = Equal?(x=w2110, y=u16 1) -> (x = y?=w2121:bool)
    n1063 = Equal?(x=w2125, y=u16 1) -> (x = y?=w2129:bool)
    n1064 = Equal?(x=w2124, y=u16 1) -> (x = y?=w2128:bool)
    n1065 = Equal?(x=w2123, y=u16 1) -> (x = y?=w2127:bool)
    n1066 = Equal?(x=w2122, y=u16 1) -> (x = y?=w2126:bool)
    n1067 = Equal?(x=w1571, y=u16 1) -> (x = y?=w1555:bool)
    n1068 = Equal?(x=w1572, y=u16 1) -> (x = y?=w1556:bool)
    n1069 = Equal?(x=w1573, y=u16 1) -> (x = y?=w1557:bool)
    n1070 = Equal?(x=w1574, y=u16 1) -> (x = y?=w1558:bool)
    n1071 = Equal?(x=w1567, y=u16 1) -> (x = y?=w1547:bool)
    n1072 = Equal?(x=w1568, y=u16 1) -> (x = y?=w1548:bool)
    n1073 = Equal?(x=w1569, y=u16 1) -> (x = y?=w1549:bool)
    n1074 = Equal?(x=w1570, y=u16 1) -> (x = y?=w1550:bool)
    n1075 = Equal?(x=w1563, y=u16 1) -> (x = y?=w1539:bool)
    n1076 = Equal?(x=w1564, y=u16 1) -> (x = y?=w1540:bool)
    n1077 = Equal?(x=w1565, y=u16 1) -> (x = y?=w1541:bool)
    n1078 = Equal?(x=w1566, y=u16 1) -> (x = y?=w1542:bool)
    n1079 = Equal?(x=w1559, y=u16 1) -> (x = y?=w1531:bool)
    n1080 = Equal?(x=w1560, y=u16 1) -> (x = y?=w1532:bool)
    n1081 = Equal?(x=w1561, y=u16 1) -> (x = y?=w1533:bool)
    n1082 = Equal?(x=w1562, y=u16 1) -> (x = y?=w1534:bool)
    n1083 = Compound Arithmetic op=AND(w2098, w2105, w2104, w2103) -> (w1914:bool)
    n1084 = Compound Arithmetic op=AND(w2118, w2119, w2120, w2121) -> (w1913:bool)
    n1085 = Compound Arithmetic op=AND(w2129, w2128, w2127, w2126) -> (w1912:bool)
    n1086 = Compound Arithmetic op=AND(w1555, w1556, w1557, w1558) -> (w1331:bool)
    n1087 = Compound Arithmetic op=AND(w1547, w1548, w1549, w1550) -> (w1330:bool)
    n1088 = Compound Arithmetic op=AND(w1539, w1540, w1541, w1542) -> (w1329:bool)
    n1089 = Compound Arithmetic op=AND(w1531, w1532, w1533, w1534) -> (w1320:bool)
    n1090 = local read "Ring 16"() -> (w2077:u16)
    n1091 = local read "Ring 15"() -> (w2076:u16)
    n1092 = local read "Ring 14"() -> (w2075:u16)
    n1093 = local read "Ring 13"() -> (w2074:u16)
    n1094 = local read "Ring 17"() -> (w2081:u16)
    n1095 = local read "Ring 16"() -> (w2080:u16)
    n1096 = local read "Ring 15"() -> (w2079:u16)
    n1097 = local read "Ring 14"() -> (w2078:u16)
    n1098 = local read "Ring 18"() -> (w2085:u16)
    n1099 = local read "Ring 17"() -> (w2084:u16)
    n1100 = local read "Ring 16"() -> (w2083:u16)
    n1101 = local read "Ring 15"() -> (w2082:u16)
    n1102 = local read "Ring 10"() -> (w1525:u16)
    n1103 = local read "Ring 16"() -> (w1526:u16)
    n1104 = local read "Ring 22"() -> (w1527:u16)
    n1105 = local read "Ring 10"() -> (w1520:u16)
    n1106 = local read "Ring 16"() -> (w1521:u16)
    n1107 = local read "Ring 22"() -> (w1522:u16)
    n1108 = local read "Ring 28"() -> (w1523:u16)
    n1109 = local read "Ring 16"() -> (w1516:u16)
    n1110 = local read "Ring 22"() -> (w1517:u16)
    n1111 = local read "Ring 28"() -> (w1518:u16)
    n1112 = local read "Ring 34"() -> (w1519:u16)
    n1113 = local read "Ring 22"() -> (w1512:u16)
    n1114 = local read "Ring 28"() -> (w1513:u16)
    n1115 = local read "Ring 34"() -> (w1514:u16)
    n1116 = local read "Ring 4"() -> (w1524:u16)
    n1117 = local read "Ring 40"() -> (w1515:u16)
    n1118 = Equal?(x=w2077, y=u16 1) -> (x = y?=w2089:bool)
    n1119 = Equal?(x=w2076, y=u16 1) -> (x = y?=w2086:bool)
    n1120 = Equal?(x=w2075, y=u16 1) -> (x = y?=w2087:bool)
    n1121 = Equal?(x=w2074, y=u16 1) -> (x = y?=w2088:bool)
    n1122 = Equal?(x=w2081, y=u16 1) -> (x = y?=w2090:bool)
    n1123 = Equal?(x=w2080, y=u16 1) -> (x = y?=w2093:bool)
    n1124 = Equal?(x=w2079, y=u16 1) -> (x = y?=w2092:bool)
    n1125 = Equal?(x=w2078, y=u16 1) -> (x = y?=w2091:bool)
    n1126 = Equal?(x=w2085, y=u16 1) -> (x = y?=w2097:bool)
    n1127 = Equal?(x=w2084, y=u16 1) -> (x = y?=w2094:bool)
    n1128 = Equal?(x=w2083, y=u16 1) -> (x = y?=w2095:bool)
    n1129 = Equal?(x=w2082, y=u16 1) -> (x = y?=w2096:bool)
    n1130 = Compound Arithmetic op=AND(w2089, w2086, w2087, w2088) -> (w1910:bool)
    n1131 = Compound Arithmetic op=AND(w2090, w2093, w2092, w2091) -> (w1909:bool)
    n1132 = Compound Arithmetic op=AND(w2097, w2094, w2095, w2096) -> (w1911:bool)
    n1133 = Equal?(x=w1524, y=u16 1) -> (x = y?=w1508:bool)
    n1134 = Equal?(x=w1525, y=u16 1) -> (x = y?=w1509:bool)
    n1135 = Equal?(x=w1526, y=u16 1) -> (x = y?=w1510:bool)
    n1136 = Equal?(x=w1527, y=u16 1) -> (x = y?=w1511:bool)
    n1137 = Equal?(x=w1520, y=u16 1) -> (x = y?=w1500:bool)
    n1138 = Equal?(x=w1521, y=u16 1) -> (x = y?=w1501:bool)
    n1139 = Equal?(x=w1522, y=u16 1) -> (x = y?=w1502:bool)
    n1140 = Equal?(x=w1523, y=u16 1) -> (x = y?=w1503:bool)
    n1141 = Equal?(x=w1516, y=u16 1) -> (x = y?=w1492:bool)
    n1142 = Equal?(x=w1517, y=u16 1) -> (x = y?=w1493:bool)
    n1143 = Equal?(x=w1518, y=u16 1) -> (x = y?=w1494:bool)
    n1144 = Equal?(x=w1519, y=u16 1) -> (x = y?=w1495:bool)
    n1145 = Equal?(x=w1512, y=u16 1) -> (x = y?=w1484:bool)
    n1146 = Equal?(x=w1513, y=u16 1) -> (x = y?=w1485:bool)
    n1147 = Equal?(x=w1514, y=u16 1) -> (x = y?=w1486:bool)
    n1148 = Equal?(x=w1515, y=u16 1) -> (x = y?=w1487:bool)
    n1149 = Compound Arithmetic op=AND(w1508, w1509, w1510, w1511) -> (w1328:bool)
    n1150 = Compound Arithmetic op=AND(w1500, w1501, w1502, w1503) -> (w1327:bool)
    n1151 = Compound Arithmetic op=AND(w1492, w1493, w1494, w1495) -> (w1326:bool)
    n1152 = Compound Arithmetic op=AND(w1484, w1485, w1486, w1487) -> (w1325:bool)
    n1153 = local read "Ring 22"() -> (w2029:u16)
    n1154 = local read "Ring 21"() -> (w2028:u16)
    n1155 = local read "Ring 20"() -> (w2027:u16)
    n1156 = local read "Ring 19"() -> (w2026:u16)
    n1157 = local read "Ring 23"() -> (w2033:u16)
    n1158 = local read "Ring 22"() -> (w2032:u16)
    n1159 = local read "Ring 21"() -> (w2031:u16)
    n1160 = local read "Ring 20"() -> (w2030:u16)
    n1161 = local read "Ring 24"() -> (w2037:u16)
    n1162 = local read "Ring 23"() -> (w2036:u16)
    n1163 = local read "Ring 22"() -> (w2035:u16)
    n1164 = local read "Ring 21"() -> (w2034:u16)
    n1165 = local read "Ring 15"() -> (w1479:u16)
    n1166 = local read "Ring 21"() -> (w1480:u16)
    n1167 = local read "Ring 15"() -> (w1474:u16)
    n1168 = local read "Ring 21"() -> (w1475:u16)
    n1169 = local read "Ring 27"() -> (w1476:u16)
    n1170 = local read "Ring 15"() -> (w1469:u16)
    n1171 = local read "Ring 21"() -> (w1470:u16)
    n1172 = local read "Ring 27"() -> (w1471:u16)
    n1173 = local read "Ring 33"() -> (w1472:u16)
    n1174 = local read "Ring 21"() -> (w1465:u16)
    n1175 = local read "Ring 27"() -> (w1466:u16)
    n1176 = local read "Ring 33"() -> (w1467:u16)
    n1177 = local read "Ring 3"() -> (w1477:u16)
    n1178 = local read "Ring 9"() -> (w1478:u16)
    n1179 = local read "Ring 9"() -> (w1473:u16)
    n1180 = local read "Ring 39"() -> (w1468:u16)
    n1181 = Equal?(x=w2029, y=u16 1) -> (x = y?=w2045:bool)
    n1182 = Equal?(x=w2028, y=u16 1) -> (x = y?=w2042:bool)
    n1183 = Equal?(x=w2027, y=u16 1) -> (x = y?=w2043:bool)
    n1184 = Equal?(x=w2026, y=u16 1) -> (x = y?=w2044:bool)
    n1185 = Equal?(x=w2033, y=u16 1) -> (x = y?=w2053:bool)
    n1186 = Equal?(x=w2032, y=u16 1) -> (x = y?=w2050:bool)
    n1187 = Equal?(x=w2031, y=u16 1) -> (x = y?=w2051:bool)
    n1188 = Equal?(x=w2030, y=u16 1) -> (x = y?=w2052:bool)
    n1189 = Equal?(x=w2037, y=u16 1) -> (x = y?=w2061:bool)
    n1190 = Equal?(x=w2036, y=u16 1) -> (x = y?=w2058:bool)
    n1191 = Equal?(x=w2035, y=u16 1) -> (x = y?=w2059:bool)
    n1192 = Equal?(x=w2034, y=u16 1) -> (x = y?=w2060:bool)
    n1193 = Compound Arithmetic op=AND(w2045, w2042, w2043, w2044) -> (w1908:bool)
    n1194 = Compound Arithmetic op=AND(w2053, w2050, w2051, w2052) -> (w1907:bool)
    n1195 = Compound Arithmetic op=AND(w2061, w2058, w2059, w2060) -> (w1906:bool)
    n1196 = Equal?(x=w1477, y=u16 1) -> (x = y?=w1461:bool)
    n1197 = Equal?(x=w1478, y=u16 1) -> (x = y?=w1462:bool)
    n1198 = Equal?(x=w1479, y=u16 1) -> (x = y?=w1463:bool)
    n1199 = Equal?(x=w1480, y=u16 1) -> (x = y?=w1464:bool)
    n1200 = Equal?(x=w1473, y=u16 1) -> (x = y?=w1453:bool)
    n1201 = Equal?(x=w1474, y=u16 1) -> (x = y?=w1454:bool)
    n1202 = Equal?(x=w1475, y=u16 1) -> (x = y?=w1455:bool)
    n1203 = Equal?(x=w1476, y=u16 1) -> (x = y?=w1456:bool)
    n1204 = Equal?(x=w1469, y=u16 1) -> (x = y?=w1445:bool)
    n1205 = Equal?(x=w1470, y=u16 1) -> (x = y?=w1446:bool)
    n1206 = Equal?(x=w1471, y=u16 1) -> (x = y?=w1447:bool)
    n1207 = Equal?(x=w1472, y=u16 1) -> (x = y?=w1448:bool)
    n1208 = Equal?(x=w1465, y=u16 1) -> (x = y?=w1437:bool)
    n1209 = Equal?(x=w1466, y=u16 1) -> (x = y?=w1438:bool)
    n1210 = Equal?(x=w1467, y=u16 1) -> (x = y?=w1439:bool)
    n1211 = Equal?(x=w1468, y=u16 1) -> (x = y?=w1440:bool)
    n1212 = Compound Arithmetic op=AND(w1461, w1462, w1463, w1464) -> (w1324:bool)
    n1213 = Compound Arithmetic op=AND(w1453, w1454, w1455, w1456) -> (w1323:bool)
    n1214 = Compound Arithmetic op=AND(w1445, w1446, w1447, w1448) -> (w1322:bool)
    n1215 = Compound Arithmetic op=AND(w1437, w1438, w1439, w1440) -> (w1321:bool)
    n1216 = local read "Ring 28"() -> (w1993:u16)
    n1217 = local read "Ring 27"() -> (w1992:u16)
    n1218 = local read "Ring 26"() -> (w1991:u16)
    n1219 = local read "Ring 25"() -> (w1990:u16)
    n1220 = local read "Ring 29"() -> (w1997:u16)
    n1221 = local read "Ring 28"() -> (w1996:u16)
    n1222 = local read "Ring 27"() -> (w1995:u16)
    n1223 = local read "Ring 26"() -> (w1994:u16)
    n1224 = local read "Ring 30"() -> (w2001:u16)
    n1225 = local read "Ring 29"() -> (w2000:u16)
    n1226 = local read "Ring 28"() -> (w1999:u16)
    n1227 = local read "Ring 27"() -> (w1998:u16)
    n1228 = Equal?(x=w1993, y=u16 1) -> (x = y?=w2009:bool)
    n1229 = Equal?(x=w1992, y=u16 1) -> (x = y?=w2006:bool)
    n1230 = Equal?(x=w1991, y=u16 1) -> (x = y?=w2007:bool)
    n1231 = Equal?(x=w1990, y=u16 1) -> (x = y?=w2008:bool)
    n1232 = Equal?(x=w1997, y=u16 1) -> (x = y?=w2017:bool)
    n1233 = Equal?(x=w1996, y=u16 1) -> (x = y?=w2014:bool)
    n1234 = Equal?(x=w1995, y=u16 1) -> (x = y?=w2015:bool)
    n1235 = Equal?(x=w1994, y=u16 1) -> (x = y?=w2016:bool)
    n1236 = Equal?(x=w2001, y=u16 1) -> (x = y?=w2025:bool)
    n1237 = Equal?(x=w2000, y=u16 1) -> (x = y?=w2022:bool)
    n1238 = Equal?(x=w1999, y=u16 1) -> (x = y?=w2023:bool)
    n1239 = Equal?(x=w1998, y=u16 1) -> (x = y?=w2024:bool)
    n1240 = local read "Ring 14"() -> (w1432:u16)
    n1241 = local read "Ring 20"() -> (w1433:u16)
    n1242 = local read "Ring 14"() -> (w1427:u16)
    n1243 = local read "Ring 20"() -> (w1428:u16)
    n1244 = local read "Ring 26"() -> (w1429:u16)
    n1245 = local read "Ring 14"() -> (w1422:u16)
    n1246 = local read "Ring 20"() -> (w1423:u16)
    n1247 = local read "Ring 26"() -> (w1424:u16)
    n1248 = local read "Ring 32"() -> (w1425:u16)
    n1249 = local read "Ring 20"() -> (w1418:u16)
    n1250 = local read "Ring 26"() -> (w1419:u16)
    n1251 = local read "Ring 32"() -> (w1420:u16)
    n1252 = local read "Ring 2"() -> (w1430:u16)
    n1253 = local read "Ring 8"() -> (w1431:u16)
    n1254 = local read "Ring 8"() -> (w1426:u16)
    n1255 = local read "Ring 38"() -> (w1421:u16)
    n1256 = Compound Arithmetic op=AND(w2009, w2006, w2007, w2008) -> (w1905:bool)
    n1257 = Compound Arithmetic op=AND(w2017, w2014, w2015, w2016) -> (w1904:bool)
    n1258 = Compound Arithmetic op=AND(w2025, w2022, w2023, w2024) -> (w1903:bool)
    n1259 = local read "Ring 34"() -> (w1957:u16)
    n1260 = local read "Ring 33"() -> (w1956:u16)
    n1261 = local read "Ring 32"() -> (w1955:u16)
    n1262 = local read "Ring 31"() -> (w1954:u16)
    n1263 = local read "Ring 35"() -> (w1961:u16)
    n1264 = local read "Ring 34"() -> (w1960:u16)
    n1265 = local read "Ring 33"() -> (w1959:u16)
    n1266 = local read "Ring 32"() -> (w1958:u16)
    n1267 = local read "Ring 36"() -> (w1965:u16)
    n1268 = local read "Ring 35"() -> (w1964:u16)
    n1269 = local read "Ring 34"() -> (w1963:u16)
    n1270 = local read "Ring 33"() -> (w1962:u16)
    n1271 = Equal?(x=w1430, y=u16 1) -> (x = y?=w1414:bool)
    n1272 = Equal?(x=w1431, y=u16 1) -> (x = y?=w1415:bool)
    n1273 = Equal?(x=w1432, y=u16 1) -> (x = y?=w1416:bool)
    n1274 = Equal?(x=w1433, y=u16 1) -> (x = y?=w1417:bool)
    n1275 = Equal?(x=w1426, y=u16 1) -> (x = y?=w1406:bool)
    n1276 = Equal?(x=w1427, y=u16 1) -> (x = y?=w1407:bool)
    n1277 = Equal?(x=w1428, y=u16 1) -> (x = y?=w1408:bool)
    n1278 = Equal?(x=w1429, y=u16 1) -> (x = y?=w1409:bool)
    n1279 = Equal?(x=w1422, y=u16 1) -> (x = y?=w1398:bool)
    n1280 = Equal?(x=w1423, y=u16 1) -> (x = y?=w1399:bool)
    n1281 = Equal?(x=w1424, y=u16 1) -> (x = y?=w1400:bool)
    n1282 = Equal?(x=w1425, y=u16 1) -> (x = y?=w1401:bool)
    n1283 = Equal?(x=w1418, y=u16 1) -> (x = y?=w1390:bool)
    n1284 = Equal?(x=w1419, y=u16 1) -> (x = y?=w1391:bool)
    n1285 = Equal?(x=w1420, y=u16 1) -> (x = y?=w1392:bool)
    n1286 = Equal?(x=w1421, y=u16 1) -> (x = y?=w1393:bool)
    n1287 = Compound Arithmetic op=AND(w1414, w1415, w1416, w1417) -> (w1319:bool)
    n1288 = Compound Arithmetic op=AND(w1406, w1407, w1408, w1409) -> (w1318:bool)
    n1289 = Compound Arithmetic op=AND(w1398, w1399, w1400, w1401) -> (w1317:bool)
    n1290 = Compound Arithmetic op=AND(w1390, w1391, w1392, w1393) -> (w1316:bool)
    n1291 = Equal?(x=w1957, y=u16 1) -> (x = y?=w1973:bool)
    n1292 = Equal?(x=w1956, y=u16 1) -> (x = y?=w1970:bool)
    n1293 = Equal?(x=w1955, y=u16 1) -> (x = y?=w1971:bool)
    n1294 = Equal?(x=w1954, y=u16 1) -> (x = y?=w1972:bool)
    n1295 = Equal?(x=w1961, y=u16 1) -> (x = y?=w1981:bool)
    n1296 = Equal?(x=w1960, y=u16 1) -> (x = y?=w1978:bool)
    n1297 = Equal?(x=w1959, y=u16 1) -> (x = y?=w1979:bool)
    n1298 = Equal?(x=w1958, y=u16 1) -> (x = y?=w1980:bool)
    n1299 = Equal?(x=w1965, y=u16 1) -> (x = y?=w1989:bool)
    n1300 = Equal?(x=w1964, y=u16 1) -> (x = y?=w1986:bool)
    n1301 = Equal?(x=w1963, y=u16 1) -> (x = y?=w1987:bool)
    n1302 = Equal?(x=w1962, y=u16 1) -> (x = y?=w1988:bool)
    n1303 = local read "Ring 13"() -> (w1385:u16)
    n1304 = local read "Ring 19"() -> (w1386:u16)
    n1305 = local read "Ring 13"() -> (w1380:u16)
    n1306 = local read "Ring 19"() -> (w1381:u16)
    n1307 = local read "Ring 25"() -> (w1382:u16)
    n1308 = local read "Ring 13"() -> (w1375:u16)
    n1309 = local read "Ring 19"() -> (w1376:u16)
    n1310 = local read "Ring 25"() -> (w1377:u16)
    n1311 = local read "Ring 31"() -> (w1378:u16)
    n1312 = local read "Ring 19"() -> (w1371:u16)
    n1313 = local read "Ring 25"() -> (w1372:u16)
    n1314 = local read "Ring 31"() -> (w1373:u16)
    n1315 = local read "Ring 1"() -> (w1383:u16)
    n1316 = local read "Ring 7"() -> (w1384:u16)
    n1317 = local read "Ring 7"() -> (w1379:u16)
    n1318 = local read "Ring 37"() -> (w1374:u16)
    n1319 = Compound Arithmetic op=AND(w1973, w1970, w1971, w1972) -> (w1902:bool)
    n1320 = Compound Arithmetic op=AND(w1981, w1978, w1979, w1980) -> (w1901:bool)
    n1321 = Compound Arithmetic op=AND(w1989, w1986, w1987, w1988) -> (w1900:bool)
    n1322 = local read "Ring 40"() -> (w1921:u16)
    n1323 = local read "Ring 39"() -> (w1920:u16)
    n1324 = local read "Ring 38"() -> (w1919:u16)
    n1325 = local read "Ring 37"() -> (w1918:u16)
    n1326 = local read "Ring 41"() -> (w1925:u16)
    n1327 = local read "Ring 40"() -> (w1924:u16)
    n1328 = local read "Ring 39"() -> (w1923:u16)
    n1329 = local read "Ring 38"() -> (w1922:u16)
    n1330 = local read "Ring 42"() -> (w1929:u16)
    n1331 = local read "Ring 41"() -> (w1928:u16)
    n1332 = local read "Ring 40"() -> (w1927:u16)
    n1333 = local read "Ring 39"() -> (w1926:u16)
    n1334 = Equal?(x=w1383, y=u16 1) -> (x = y?=w1367:bool)
    n1335 = Equal?(x=w1384, y=u16 1) -> (x = y?=w1368:bool)
    n1336 = Equal?(x=w1385, y=u16 1) -> (x = y?=w1369:bool)
    n1337 = Equal?(x=w1386, y=u16 1) -> (x = y?=w1370:bool)
    n1338 = Equal?(x=w1379, y=u16 1) -> (x = y?=w1359:bool)
    n1339 = Equal?(x=w1380, y=u16 1) -> (x = y?=w1360:bool)
    n1340 = Equal?(x=w1381, y=u16 1) -> (x = y?=w1361:bool)
    n1341 = Equal?(x=w1382, y=u16 1) -> (x = y?=w1362:bool)
    n1342 = Equal?(x=w1375, y=u16 1) -> (x = y?=w1351:bool)
    n1343 = Equal?(x=w1376, y=u16 1) -> (x = y?=w1352:bool)
    n1344 = Equal?(x=w1377, y=u16 1) -> (x = y?=w1353:bool)
    n1345 = Equal?(x=w1378, y=u16 1) -> (x = y?=w1354:bool)
    n1346 = Equal?(x=w1371, y=u16 1) -> (x = y?=w1343:bool)
    n1347 = Equal?(x=w1372, y=u16 1) -> (x = y?=w1344:bool)
    n1348 = Equal?(x=w1373, y=u16 1) -> (x = y?=w1345:bool)
    n1349 = Equal?(x=w1374, y=u16 1) -> (x = y?=w1346:bool)
    n1350 = Compound Arithmetic op=AND(w1367, w1368, w1369, w1370) -> (w1315:bool)
    n1351 = Compound Arithmetic op=AND(w1359, w1360, w1361, w1362) -> (w1314:bool)
    n1352 = Compound Arithmetic op=AND(w1351, w1352, w1353, w1354) -> (w1313:bool)
    n1353 = Compound Arithmetic op=AND(w1343, w1344, w1345, w1346) -> (w1312:bool)
    n1354 = Equal?(x=w1921, y=u16 1) -> (x = y?=w1937:bool)
    n1355 = Equal?(x=w1920, y=u16 1) -> (x = y?=w1934:bool)
    n1356 = Equal?(x=w1919, y=u16 1) -> (x = y?=w1935:bool)
    n1357 = Equal?(x=w1918, y=u16 1) -> (x = y?=w1936:bool)
    n1358 = Equal?(x=w1925, y=u16 1) -> (x = y?=w1945:bool)
    n1359 = Equal?(x=w1924, y=u16 1) -> (x = y?=w1942:bool)
    n1360 = Equal?(x=w1923, y=u16 1) -> (x = y?=w1943:bool)
    n1361 = Equal?(x=w1922, y=u16 1) -> (x = y?=w1944:bool)
    n1362 = Equal?(x=w1929, y=u16 1) -> (x = y?=w1953:bool)
    n1363 = Equal?(x=w1928, y=u16 1) -> (x = y?=w1950:bool)
    n1364 = Equal?(x=w1927, y=u16 1) -> (x = y?=w1951:bool)
    n1365 = Equal?(x=w1926, y=u16 1) -> (x = y?=w1952:bool)
    n1366 = Compound Arithmetic op=AND(w1937, w1934, w1935, w1936) -> (w1899:bool)
    n1367 = Compound Arithmetic op=AND(w1945, w1942, w1943, w1944) -> (w1898:bool)
    n1368 = Compound Arithmetic op=AND(w1953, w1950, w1951, w1952) -> (w1897:bool)
    n1369 = local read "Ring 37"() -> (w57:u16)
    n1370 = local read "Ring 38"() -> (w56:u16)
    n1371 = local read "Ring 39"() -> (w55:u16)
    n1372 = local read "Ring 40"() -> (w54:u16)
    n1373 = local read "Ring 41"() -> (w53:u16)
    n1374 = local read "Ring 42"() -> (w52:u16)
    n1375 = local read "Ring 30"() -> (w72:u16)
    n1376 = local read "Ring 29"() -> (w93:u16)
    n1377 = local read "Ring 28"() -> (w71:u16)
    n1378 = local read "Ring 27"() -> (w70:u16)
    n1379 = local read "Ring 26"() -> (w69:u16)
    n1380 = local read "Ring 10"() -> (w73:u16)
    n1381 = local read "Ring 20"() -> (w92:u16)
    n1382 = local read "Ring 19"() -> (w91:u16)
    n1383 = local read "Ring 18"() -> (w90:u16)
    n1384 = local read "Ring 17"() -> (w89:u16)
    n1385 = local read "Ring 16"() -> (w88:u16)
    n1386 = local read "Ring 15"() -> (w87:u16)
    n1387 = local read "Ring 14"() -> (w86:u16)
    n1388 = local read "Ring 13"() -> (w85:u16)
    n1389 = local read "Ring 12"() -> (w84:u16)
    n1390 = local read "Ring 11"() -> (w83:u16)
    n1391 = local read "Ring 25"() -> (w68:u16)
    n1392 = local read "Ring 24"() -> (w67:u16)
    n1393 = local read "Ring 23"() -> (w66:u16)
    n1394 = local read "Ring 22"() -> (w65:u16)
    n1395 = local read "Ring 21"() -> (w64:u16)
    n1396 = local read "Ring 36"() -> (w58:u16)
    n1397 = local read "Ring 35"() -> (w59:u16)
    n1398 = local read "Ring 34"() -> (w60:u16)
    n1399 = local read "Ring 33"() -> (w61:u16)
    n1400 = local read "Ring 32"() -> (w62:u16)
    n1401 = local read "Ring 31"() -> (w63:u16)
    n1402 = local read "Ring 9"() -> (w74:u16)
    n1403 = local read "Ring 8"() -> (w75:u16)
    n1404 = local read "Ring 7"() -> (w76:u16)
    n1405 = local read "Ring 6"() -> (w77:u16)
    n1406 = local read "Ring 5"() -> (w78:u16)
    n1407 = local read "Ring 4"() -> (w79:u16)
    n1408 = local read "Ring 3"() -> (w80:u16)
    n1409 = local read "Ring 2"() -> (w81:u16)
    n1410 = local read "Ring 1"() -> (w82:u16)
    n1411 = Compound Arithmetic op=OR(w1335, w1334, w1333, w1332, w1331, w1330, w1329, w1320, w1328, w1327, w1326, w1325, w1324, w1323, w1322, w1321, w1319, w1318, w1317, w1316, w1315, w1314, w1313, w1312) -> (w1311:bool)
    n1412 = Not Equal To 0?(x=w57) -> (x != 0?=w16:bool)
    n1413 = Not Equal To 0?(x=w56) -> (x != 0?=w17:bool)
    n1414 = Not Equal To 0?(x=w55) -> (x != 0?=w18:bool)
    n1415 = Not Equal To 0?(x=w54) -> (x != 0?=w19:bool)
    n1416 = Not Equal To 0?(x=w53) -> (x != 0?=w20:bool)
    n1417 = Not Equal To 0?(x=w52) -> (x != 0?=w21:bool)
    n1418 = Not Equal To 0?(x=w72) -> (x != 0?=w22:bool)
    n1419 = Not Equal To 0?(x=w93) -> (x != 0?=w23:bool)
    n1420 = Not Equal To 0?(x=w71) -> (x != 0?=w24:bool)
    n1421 = Not Equal To 0?(x=w70) -> (x != 0?=w25:bool)
    n1422 = Not Equal To 0?(x=w69) -> (x != 0?=w26:bool)
    n1423 = Not Equal To 0?(x=w73) -> (x != 0?=w32:bool)
    n1424 = Not Equal To 0?(x=w74) -> (x != 0?=w33:bool)
    n1425 = Not Equal To 0?(x=w75) -> (x != 0?=w34:bool)
    n1426 = Not Equal To 0?(x=w76) -> (x != 0?=w35:bool)
    n1427 = Not Equal To 0?(x=w77) -> (x != 0?=w36:bool)
    n1428 = Not Equal To 0?(x=w92) -> (x != 0?=w46:bool)
    n1429 = Not Equal To 0?(x=w91) -> (x != 0?=w47:bool)
    n1430 = Not Equal To 0?(x=w90) -> (x != 0?=w48:bool)
    n1431 = Not Equal To 0?(x=w89) -> (x != 0?=w49:bool)
    n1432 = Not Equal To 0?(x=w88) -> (x != 0?=w51:bool)
    n1433 = Not Equal To 0?(x=w87) -> (x != 0?=w50:bool)
    n1434 = Not Equal To 0?(x=w86) -> (x != 0?=w45:bool)
    n1435 = Not Equal To 0?(x=w85) -> (x != 0?=w44:bool)
    n1436 = Not Equal To 0?(x=w84) -> (x != 0?=w43:bool)
    n1437 = Not Equal To 0?(x=w83) -> (x != 0?=w42:bool)
    n1438 = Not Equal To 0?(x=w78) -> (x != 0?=w41:bool)
    n1439 = Not Equal To 0?(x=w79) -> (x != 0?=w40:bool)
    n1440 = Not Equal To 0?(x=w80) -> (x != 0?=w39:bool)
    n1441 = Not Equal To 0?(x=w81) -> (x != 0?=w38:bool)
    n1442 = Not Equal To 0?(x=w82) -> (x != 0?=w37:bool)
    n1443 = Not Equal To 0?(x=w68) -> (x != 0?=w31:bool)
    n1444 = Not Equal To 0?(x=w67) -> (x != 0?=w30:bool)
    n1445 = Not Equal To 0?(x=w66) -> (x != 0?=w29:bool)
    n1446 = Not Equal To 0?(x=w65) -> (x != 0?=w28:bool)
    n1447 = Not Equal To 0?(x=w64) -> (x != 0?=w27:bool)
    n1448 = Not Equal To 0?(x=w58) -> (x != 0?=w15:bool)
    n1449 = Not Equal To 0?(x=w59) -> (x != 0?=w14:bool)
    n1450 = Not Equal To 0?(x=w60) -> (x != 0?=w13:bool)
    n1451 = Not Equal To 0?(x=w61) -> (x != 0?=w12:bool)
    n1452 = Not Equal To 0?(x=w62) -> (x != 0?=w11:bool)
    n1453 = Not Equal To 0?(x=w63) -> (x != 0?=w10:bool)
    n1454 = Compound Arithmetic op=OR(w1917, w1916, w1915, w1914, w1913, w1912, w1911, w1910, w1909, w1908, w1907, w1906, w1905, w1904, w1903, w1902, w1901, w1900, w1899, w1898, w1897) -> (w2146:bool)
    n1455 = Compound Arithmetic op=AND(w16, w17, w18, w19, w20, w21, w22, w23, w24, w25, w26, w32, w33, w34, w35, w36, w46, w47, w48, w49, w51, w50, w45, w44, w43, w42, w41, w40, w39, w38, w37, w31, w30, w29, w28, w27, w15, w14, w13, w12, w11, w10) -> (w9:bool)
    n1456 = case shown="True" w1311 {
      selector: w1311 -> [_ w2206]
      frame False {
      }
      frame True {
        n1457 = property on="Player Verde" class="DigNum (strict)"() -> ("Value"=w2208:dbl)  [unwired: 2 in, 2 out]
        n1458 = Increment(x=w2208) -> (x+1=w2207:dbl)
        n1459 = call "Display Message to User3"("Enable"=w2206) -> ()  [unwired: 9 in, 2 out]
        n1460 = property on="Player Verde" class="DigNum (strict)"("Value"=w2207) -> ()  [unwired: 2 in, 2 out]
      }
    }
    n1461 = case shown="True" w9 {
      selector: w9 -> [_ w2187]
      frame False {
      }
      frame True {
        n1462 = call "Display Message to User10"("Enable"=w2187) -> ()  [unwired: 9 in, 2 out]
      }
    }
    n1463 = case shown="True" w2146 {
      selector: w2146 -> [_ w2212]
      frame False {
      }
      frame True {
        n1464 = property on="Player Verde" class="DigNum (strict)"() -> ("Value"=w2214:dbl)  [unwired: 2 in, 2 out]
        n1465 = Increment(x=w2214) -> (x+1=w2213:dbl)
        n1466 = call "Display Message to User"("Enable"=w2212) -> ()  [unwired: 9 in, 2 out]
        n1467 = property on="Player Verde" class="DigNum (strict)"("Value"=w2213) -> ()  [unwired: 2 in, 2 out]
      }
    }
    n1468 = local read "Ring 42"() -> (w1041:u16)
    n1469 = local read "Ring 36"() -> (w1042:u16)
    n1470 = local read "Ring 30"() -> (w1043:u16)
    n1471 = local read "Ring 24"() -> (w1044:u16)
    n1472 = local read "Ring 36"() -> (w1037:u16)
    n1473 = local read "Ring 30"() -> (w1038:u16)
    n1474 = local read "Ring 24"() -> (w1039:u16)
    n1475 = local read "Ring 18"() -> (w1040:u16)
    n1476 = local read "Ring 30"() -> (w1033:u16)
    n1477 = local read "Ring 24"() -> (w1034:u16)
    n1478 = local read "Ring 18"() -> (w1035:u16)
    n1479 = local read "Ring 12"() -> (w1036:u16)
    n1480 = local read "Ring 24"() -> (w1029:u16)
    n1481 = local read "Ring 18"() -> (w1030:u16)
    n1482 = local read "Ring 12"() -> (w1031:u16)
    n1483 = local read "Ring 5"() -> (w980:u16)
    n1484 = local read "Ring 5"() -> (w1639:u16)
    n1485 = local read "Ring 4"() -> (w978:u16)
    n1486 = local read "Ring 4"() -> (w1641:u16)
    n1487 = local read "Ring 3"() -> (w976:u16)
    n1488 = local read "Ring 3"() -> (w1643:u16)
    n1489 = local read "Ring 2"() -> (w974:u16)
    n1490 = local read "Ring 2"() -> (w1645:u16)
    n1491 = local read "Ring 3"() -> (w993:u16)
    n1492 = local read "Ring 3"() -> (w1626:u16)
    n1493 = local read "Ring 4"() -> (w994:u16)
    n1494 = local read "Ring 4"() -> (w1625:u16)
    n1495 = local read "Ring 5"() -> (w995:u16)
    n1496 = local read "Ring 5"() -> (w1624:u16)
    n1497 = local read "Ring 6"() -> (w996:u16)
    n1498 = local read "Ring 6"() -> (w1623:u16)
    n1499 = local read "Ring 4"() -> (w963:u16)
    n1500 = local read "Ring 4"() -> (w1656:u16)
    n1501 = local read "Ring 3"() -> (w960:u16)
    n1502 = local read "Ring 3"() -> (w1659:u16)
    n1503 = local read "Ring 2"() -> (w961:u16)
    n1504 = local read "Ring 2"() -> (w1658:u16)
    n1505 = local read "Ring 1"() -> (w962:u16)
    n1506 = local read "Ring 1"() -> (w1657:u16)
    n1507 = local read "Ring 6"() -> (w1032:u16)
    n1508 = Equal?(x=w980, y=u16 2) -> (x = y?=w981:bool)
    n1509 = Equal?(x=w1639, y=u16 2) -> (x = y?=w1638:bool)
    n1510 = Equal?(x=w978, y=u16 2) -> (x = y?=w982:bool)
    n1511 = Equal?(x=w1641, y=u16 2) -> (x = y?=w1637:bool)
    n1512 = Equal?(x=w976, y=u16 2) -> (x = y?=w983:bool)
    n1513 = Equal?(x=w1643, y=u16 2) -> (x = y?=w1636:bool)
    n1514 = Equal?(x=w974, y=u16 2) -> (x = y?=w984:bool)
    n1515 = Equal?(x=w1645, y=u16 2) -> (x = y?=w1635:bool)
    n1516 = Equal?(x=w993, y=u16 2) -> (x = y?=w989:bool)
    n1517 = Equal?(x=w1626, y=u16 2) -> (x = y?=w1630:bool)
    n1518 = Equal?(x=w994, y=u16 2) -> (x = y?=w990:bool)
    n1519 = Equal?(x=w1625, y=u16 2) -> (x = y?=w1629:bool)
    n1520 = Equal?(x=w995, y=u16 2) -> (x = y?=w991:bool)
    n1521 = Equal?(x=w1624, y=u16 2) -> (x = y?=w1628:bool)
    n1522 = Equal?(x=w996, y=u16 2) -> (x = y?=w992:bool)
    n1523 = Equal?(x=w1623, y=u16 2) -> (x = y?=w1627:bool)
    n1524 = Equal?(x=w963, y=u16 2) -> (x = y?=w967:bool)
    n1525 = Equal?(x=w1656, y=u16 2) -> (x = y?=w1652:bool)
    n1526 = Equal?(x=w960, y=u16 2) -> (x = y?=w966:bool)
    n1527 = Equal?(x=w1659, y=u16 2) -> (x = y?=w1653:bool)
    n1528 = Equal?(x=w961, y=u16 2) -> (x = y?=w965:bool)
    n1529 = Equal?(x=w1658, y=u16 2) -> (x = y?=w1654:bool)
    n1530 = Equal?(x=w962, y=u16 2) -> (x = y?=w964:bool)
    n1531 = Equal?(x=w1657, y=u16 2) -> (x = y?=w1655:bool)
    n1532 = Equal?(x=w1041, y=u16 2) -> (x = y?=w1025:bool)
    n1533 = Equal?(x=w1042, y=u16 2) -> (x = y?=w1026:bool)
    n1534 = Equal?(x=w1043, y=u16 2) -> (x = y?=w1027:bool)
    n1535 = Equal?(x=w1044, y=u16 2) -> (x = y?=w1028:bool)
    n1536 = Equal?(x=w1037, y=u16 2) -> (x = y?=w1017:bool)
    n1537 = Equal?(x=w1038, y=u16 2) -> (x = y?=w1018:bool)
    n1538 = Equal?(x=w1039, y=u16 2) -> (x = y?=w1019:bool)
    n1539 = Equal?(x=w1040, y=u16 2) -> (x = y?=w1020:bool)
    n1540 = Equal?(x=w1033, y=u16 2) -> (x = y?=w1009:bool)
    n1541 = Equal?(x=w1034, y=u16 2) -> (x = y?=w1010:bool)
    n1542 = Equal?(x=w1035, y=u16 2) -> (x = y?=w1011:bool)
    n1543 = Equal?(x=w1036, y=u16 2) -> (x = y?=w1012:bool)
    n1544 = Equal?(x=w1029, y=u16 2) -> (x = y?=w1001:bool)
    n1545 = Equal?(x=w1030, y=u16 2) -> (x = y?=w1002:bool)
    n1546 = Equal?(x=w1031, y=u16 2) -> (x = y?=w1003:bool)
    n1547 = Equal?(x=w1032, y=u16 2) -> (x = y?=w1004:bool)
    n1548 = Compound Arithmetic op=AND(w1001, w1002, w1003, w1004) -> (w1287:bool)
    n1549 = Compound Arithmetic op=AND(w981, w982, w983, w984) -> (w743:bool)
    n1550 = Compound Arithmetic op=AND(w1638, w1637, w1636, w1635) -> (w1876:bool)
    n1551 = Compound Arithmetic op=AND(w989, w990, w991, w992) -> (w742:bool)
    n1552 = Compound Arithmetic op=AND(w1630, w1629, w1628, w1627) -> (w1877:bool)
    n1553 = Compound Arithmetic op=AND(w967, w966, w965, w964) -> (w741:bool)
    n1554 = Compound Arithmetic op=AND(w1652, w1653, w1654, w1655) -> (w1878:bool)
    n1555 = Compound Arithmetic op=AND(w1017, w1018, w1019, w1020) -> (w1285:bool)
    n1556 = Compound Arithmetic op=AND(w1009, w1010, w1011, w1012) -> (w1286:bool)
    n1557 = Compound Arithmetic op=AND(w1025, w1026, w1027, w1028) -> (w1284:bool)
    n1558 = local read "Ring 10"() -> (w928:u16)
    n1559 = local read "Ring 10"() -> (w1691:u16)
    n1560 = local read "Ring 11"() -> (w939:u16)
    n1561 = local read "Ring 11"() -> (w1680:u16)
    n1562 = local read "Ring 10"() -> (w938:u16)
    n1563 = local read "Ring 10"() -> (w1681:u16)
    n1564 = local read "Ring 12"() -> (w951:u16)
    n1565 = local read "Ring 12"() -> (w1668:u16)
    n1566 = local read "Ring 11"() -> (w950:u16)
    n1567 = local read "Ring 11"() -> (w1669:u16)
    n1568 = local read "Ring 10"() -> (w949:u16)
    n1569 = local read "Ring 10"() -> (w1670:u16)
    n1570 = local read "Ring 9"() -> (w927:u16)
    n1571 = local read "Ring 9"() -> (w1692:u16)
    n1572 = local read "Ring 8"() -> (w926:u16)
    n1573 = local read "Ring 8"() -> (w1693:u16)
    n1574 = local read "Ring 7"() -> (w925:u16)
    n1575 = local read "Ring 7"() -> (w1694:u16)
    n1576 = local read "Ring 9"() -> (w937:u16)
    n1577 = local read "Ring 9"() -> (w1682:u16)
    n1578 = local read "Ring 8"() -> (w936:u16)
    n1579 = local read "Ring 8"() -> (w1683:u16)
    n1580 = local read "Ring 9"() -> (w948:u16)
    n1581 = local read "Ring 9"() -> (w1671:u16)
    n1582 = local read "Ring 11"() -> (w1047:u16)
    n1583 = local read "Ring 17"() -> (w1046:u16)
    n1584 = local read "Ring 23"() -> (w1045:u16)
    n1585 = local read "Ring 11"() -> (w1052:u16)
    n1586 = local read "Ring 17"() -> (w1051:u16)
    n1587 = local read "Ring 23"() -> (w1050:u16)
    n1588 = local read "Ring 29"() -> (w1049:u16)
    n1589 = local read "Ring 17"() -> (w1056:u16)
    n1590 = local read "Ring 23"() -> (w1055:u16)
    n1591 = local read "Ring 29"() -> (w1054:u16)
    n1592 = local read "Ring 35"() -> (w1053:u16)
    n1593 = local read "Ring 23"() -> (w1060:u16)
    n1594 = local read "Ring 29"() -> (w1059:u16)
    n1595 = local read "Ring 35"() -> (w1058:u16)
    n1596 = local read "Ring 5"() -> (w1048:u16)
    n1597 = local read "Ring 41"() -> (w1057:u16)
    n1598 = Equal?(x=w928, y=u16 2) -> (x = y?=w924:bool)
    n1599 = Equal?(x=w1691, y=u16 2) -> (x = y?=w1695:bool)
    n1600 = Equal?(x=w927, y=u16 2) -> (x = y?=w931:bool)
    n1601 = Equal?(x=w1692, y=u16 2) -> (x = y?=w1688:bool)
    n1602 = Equal?(x=w926, y=u16 2) -> (x = y?=w930:bool)
    n1603 = Equal?(x=w1693, y=u16 2) -> (x = y?=w1689:bool)
    n1604 = Equal?(x=w925, y=u16 2) -> (x = y?=w929:bool)
    n1605 = Equal?(x=w1694, y=u16 2) -> (x = y?=w1690:bool)
    n1606 = Equal?(x=w939, y=u16 2) -> (x = y?=w944:bool)
    n1607 = Equal?(x=w1680, y=u16 2) -> (x = y?=w1675:bool)
    n1608 = Equal?(x=w938, y=u16 2) -> (x = y?=w945:bool)
    n1609 = Equal?(x=w1681, y=u16 2) -> (x = y?=w1674:bool)
    n1610 = Equal?(x=w937, y=u16 2) -> (x = y?=w946:bool)
    n1611 = Equal?(x=w1682, y=u16 2) -> (x = y?=w1673:bool)
    n1612 = Equal?(x=w936, y=u16 2) -> (x = y?=w947:bool)
    n1613 = Equal?(x=w1683, y=u16 2) -> (x = y?=w1672:bool)
    n1614 = Equal?(x=w951, y=u16 2) -> (x = y?=w955:bool)
    n1615 = Equal?(x=w1668, y=u16 2) -> (x = y?=w1664:bool)
    n1616 = Equal?(x=w950, y=u16 2) -> (x = y?=w954:bool)
    n1617 = Equal?(x=w1669, y=u16 2) -> (x = y?=w1665:bool)
    n1618 = Equal?(x=w949, y=u16 2) -> (x = y?=w953:bool)
    n1619 = Equal?(x=w1670, y=u16 2) -> (x = y?=w1666:bool)
    n1620 = Equal?(x=w948, y=u16 2) -> (x = y?=w952:bool)
    n1621 = Equal?(x=w1671, y=u16 2) -> (x = y?=w1667:bool)
    n1622 = Equal?(x=w1048, y=u16 2) -> (x = y?=w1064:bool)
    n1623 = Equal?(x=w1047, y=u16 2) -> (x = y?=w1063:bool)
    n1624 = Equal?(x=w1046, y=u16 2) -> (x = y?=w1062:bool)
    n1625 = Equal?(x=w1045, y=u16 2) -> (x = y?=w1061:bool)
    n1626 = Equal?(x=w1052, y=u16 2) -> (x = y?=w1072:bool)
    n1627 = Equal?(x=w1051, y=u16 2) -> (x = y?=w1071:bool)
    n1628 = Equal?(x=w1050, y=u16 2) -> (x = y?=w1070:bool)
    n1629 = Equal?(x=w1049, y=u16 2) -> (x = y?=w1069:bool)
    n1630 = Equal?(x=w1056, y=u16 2) -> (x = y?=w1080:bool)
    n1631 = Equal?(x=w1055, y=u16 2) -> (x = y?=w1079:bool)
    n1632 = Equal?(x=w1054, y=u16 2) -> (x = y?=w1078:bool)
    n1633 = Equal?(x=w1053, y=u16 2) -> (x = y?=w1077:bool)
    n1634 = Equal?(x=w1060, y=u16 2) -> (x = y?=w1088:bool)
    n1635 = Equal?(x=w1059, y=u16 2) -> (x = y?=w1087:bool)
    n1636 = Equal?(x=w1058, y=u16 2) -> (x = y?=w1086:bool)
    n1637 = Equal?(x=w1057, y=u16 2) -> (x = y?=w1085:bool)
    n1638 = Compound Arithmetic op=AND(w924, w931, w930, w929) -> (w740:bool)
    n1639 = Compound Arithmetic op=AND(w1695, w1688, w1689, w1690) -> (w1879:bool)
    n1640 = Compound Arithmetic op=AND(w944, w945, w946, w947) -> (w739:bool)
    n1641 = Compound Arithmetic op=AND(w1675, w1674, w1673, w1672) -> (w1880:bool)
    n1642 = Compound Arithmetic op=AND(w955, w954, w953, w952) -> (w738:bool)
    n1643 = Compound Arithmetic op=AND(w1664, w1665, w1666, w1667) -> (w1881:bool)
    n1644 = Compound Arithmetic op=AND(w1064, w1063, w1062, w1061) -> (w1288:bool)
    n1645 = Compound Arithmetic op=AND(w1072, w1071, w1070, w1069) -> (w1289:bool)
    n1646 = Compound Arithmetic op=AND(w1080, w1079, w1078, w1077) -> (w1290:bool)
    n1647 = Compound Arithmetic op=AND(w1088, w1087, w1086, w1085) -> (w1299:bool)
    n1648 = local read "Ring 16"() -> (w903:u16)
    n1649 = local read "Ring 16"() -> (w1716:u16)
    n1650 = local read "Ring 15"() -> (w902:u16)
    n1651 = local read "Ring 15"() -> (w1717:u16)
    n1652 = local read "Ring 14"() -> (w901:u16)
    n1653 = local read "Ring 14"() -> (w1718:u16)
    n1654 = local read "Ring 13"() -> (w900:u16)
    n1655 = local read "Ring 13"() -> (w1719:u16)
    n1656 = local read "Ring 17"() -> (w907:u16)
    n1657 = local read "Ring 17"() -> (w1712:u16)
    n1658 = local read "Ring 16"() -> (w906:u16)
    n1659 = local read "Ring 16"() -> (w1713:u16)
    n1660 = local read "Ring 15"() -> (w905:u16)
    n1661 = local read "Ring 15"() -> (w1714:u16)
    n1662 = local read "Ring 14"() -> (w904:u16)
    n1663 = local read "Ring 14"() -> (w1715:u16)
    n1664 = local read "Ring 18"() -> (w911:u16)
    n1665 = local read "Ring 18"() -> (w1708:u16)
    n1666 = local read "Ring 17"() -> (w910:u16)
    n1667 = local read "Ring 17"() -> (w1709:u16)
    n1668 = local read "Ring 16"() -> (w909:u16)
    n1669 = local read "Ring 16"() -> (w1710:u16)
    n1670 = local read "Ring 15"() -> (w908:u16)
    n1671 = local read "Ring 15"() -> (w1711:u16)
    n1672 = local read "Ring 10"() -> (w1094:u16)
    n1673 = local read "Ring 16"() -> (w1093:u16)
    n1674 = local read "Ring 22"() -> (w1092:u16)
    n1675 = local read "Ring 10"() -> (w1099:u16)
    n1676 = local read "Ring 16"() -> (w1098:u16)
    n1677 = local read "Ring 22"() -> (w1097:u16)
    n1678 = local read "Ring 28"() -> (w1096:u16)
    n1679 = local read "Ring 16"() -> (w1103:u16)
    n1680 = local read "Ring 22"() -> (w1102:u16)
    n1681 = local read "Ring 28"() -> (w1101:u16)
    n1682 = local read "Ring 34"() -> (w1100:u16)
    n1683 = local read "Ring 22"() -> (w1107:u16)
    n1684 = local read "Ring 28"() -> (w1106:u16)
    n1685 = local read "Ring 34"() -> (w1105:u16)
    n1686 = local read "Ring 4"() -> (w1095:u16)
    n1687 = local read "Ring 40"() -> (w1104:u16)
    n1688 = Equal?(x=w903, y=u16 2) -> (x = y?=w915:bool)
    n1689 = Equal?(x=w1716, y=u16 2) -> (x = y?=w1704:bool)
    n1690 = Equal?(x=w902, y=u16 2) -> (x = y?=w912:bool)
    n1691 = Equal?(x=w1717, y=u16 2) -> (x = y?=w1707:bool)
    n1692 = Equal?(x=w901, y=u16 2) -> (x = y?=w913:bool)
    n1693 = Equal?(x=w1718, y=u16 2) -> (x = y?=w1706:bool)
    n1694 = Equal?(x=w900, y=u16 2) -> (x = y?=w914:bool)
    n1695 = Equal?(x=w1719, y=u16 2) -> (x = y?=w1705:bool)
    n1696 = Equal?(x=w907, y=u16 2) -> (x = y?=w916:bool)
    n1697 = Equal?(x=w1712, y=u16 2) -> (x = y?=w1703:bool)
    n1698 = Equal?(x=w906, y=u16 2) -> (x = y?=w919:bool)
    n1699 = Equal?(x=w1713, y=u16 2) -> (x = y?=w1700:bool)
    n1700 = Equal?(x=w905, y=u16 2) -> (x = y?=w918:bool)
    n1701 = Equal?(x=w1714, y=u16 2) -> (x = y?=w1701:bool)
    n1702 = Equal?(x=w904, y=u16 2) -> (x = y?=w917:bool)
    n1703 = Equal?(x=w1715, y=u16 2) -> (x = y?=w1702:bool)
    n1704 = Equal?(x=w911, y=u16 2) -> (x = y?=w923:bool)
    n1705 = Equal?(x=w1708, y=u16 2) -> (x = y?=w1696:bool)
    n1706 = Equal?(x=w910, y=u16 2) -> (x = y?=w920:bool)
    n1707 = Equal?(x=w1709, y=u16 2) -> (x = y?=w1699:bool)
    n1708 = Equal?(x=w909, y=u16 2) -> (x = y?=w921:bool)
    n1709 = Equal?(x=w1710, y=u16 2) -> (x = y?=w1698:bool)
    n1710 = Equal?(x=w908, y=u16 2) -> (x = y?=w922:bool)
    n1711 = Equal?(x=w1711, y=u16 2) -> (x = y?=w1697:bool)
    n1712 = Equal?(x=w1095, y=u16 2) -> (x = y?=w1111:bool)
    n1713 = Equal?(x=w1094, y=u16 2) -> (x = y?=w1110:bool)
    n1714 = Equal?(x=w1093, y=u16 2) -> (x = y?=w1109:bool)
    n1715 = Equal?(x=w1092, y=u16 2) -> (x = y?=w1108:bool)
    n1716 = Equal?(x=w1099, y=u16 2) -> (x = y?=w1119:bool)
    n1717 = Equal?(x=w1098, y=u16 2) -> (x = y?=w1118:bool)
    n1718 = Equal?(x=w1097, y=u16 2) -> (x = y?=w1117:bool)
    n1719 = Equal?(x=w1096, y=u16 2) -> (x = y?=w1116:bool)
    n1720 = Equal?(x=w1103, y=u16 2) -> (x = y?=w1127:bool)
    n1721 = Equal?(x=w1102, y=u16 2) -> (x = y?=w1126:bool)
    n1722 = Equal?(x=w1101, y=u16 2) -> (x = y?=w1125:bool)
    n1723 = Equal?(x=w1100, y=u16 2) -> (x = y?=w1124:bool)
    n1724 = Equal?(x=w1107, y=u16 2) -> (x = y?=w1135:bool)
    n1725 = Equal?(x=w1106, y=u16 2) -> (x = y?=w1134:bool)
    n1726 = Equal?(x=w1105, y=u16 2) -> (x = y?=w1133:bool)
    n1727 = Equal?(x=w1104, y=u16 2) -> (x = y?=w1132:bool)
    n1728 = Compound Arithmetic op=AND(w915, w912, w913, w914) -> (w736:bool)
    n1729 = Compound Arithmetic op=AND(w1704, w1707, w1706, w1705) -> (w1883:bool)
    n1730 = Compound Arithmetic op=AND(w916, w919, w918, w917) -> (w735:bool)
    n1731 = Compound Arithmetic op=AND(w1703, w1700, w1701, w1702) -> (w1884:bool)
    n1732 = Compound Arithmetic op=AND(w923, w920, w921, w922) -> (w737:bool)
    n1733 = Compound Arithmetic op=AND(w1696, w1699, w1698, w1697) -> (w1882:bool)
    n1734 = Compound Arithmetic op=AND(w1111, w1110, w1109, w1108) -> (w1291:bool)
    n1735 = Compound Arithmetic op=AND(w1119, w1118, w1117, w1116) -> (w1292:bool)
    n1736 = Compound Arithmetic op=AND(w1127, w1126, w1125, w1124) -> (w1293:bool)
    n1737 = Compound Arithmetic op=AND(w1135, w1134, w1133, w1132) -> (w1294:bool)
    n1738 = local read "Ring 22"() -> (w855:u16)
    n1739 = local read "Ring 22"() -> (w1764:u16)
    n1740 = local read "Ring 21"() -> (w854:u16)
    n1741 = local read "Ring 21"() -> (w1765:u16)
    n1742 = local read "Ring 20"() -> (w853:u16)
    n1743 = local read "Ring 20"() -> (w1766:u16)
    n1744 = local read "Ring 19"() -> (w852:u16)
    n1745 = local read "Ring 19"() -> (w1767:u16)
    n1746 = local read "Ring 23"() -> (w859:u16)
    n1747 = local read "Ring 23"() -> (w1760:u16)
    n1748 = local read "Ring 22"() -> (w858:u16)
    n1749 = local read "Ring 22"() -> (w1761:u16)
    n1750 = local read "Ring 21"() -> (w857:u16)
    n1751 = local read "Ring 21"() -> (w1762:u16)
    n1752 = local read "Ring 20"() -> (w856:u16)
    n1753 = local read "Ring 20"() -> (w1763:u16)
    n1754 = local read "Ring 24"() -> (w863:u16)
    n1755 = local read "Ring 24"() -> (w1756:u16)
    n1756 = local read "Ring 23"() -> (w862:u16)
    n1757 = local read "Ring 23"() -> (w1757:u16)
    n1758 = local read "Ring 22"() -> (w861:u16)
    n1759 = local read "Ring 22"() -> (w1758:u16)
    n1760 = local read "Ring 21"() -> (w860:u16)
    n1761 = local read "Ring 21"() -> (w1759:u16)
    n1762 = local read "Ring 15"() -> (w1140:u16)
    n1763 = local read "Ring 21"() -> (w1139:u16)
    n1764 = local read "Ring 15"() -> (w1145:u16)
    n1765 = local read "Ring 21"() -> (w1144:u16)
    n1766 = local read "Ring 27"() -> (w1143:u16)
    n1767 = local read "Ring 15"() -> (w1150:u16)
    n1768 = local read "Ring 21"() -> (w1149:u16)
    n1769 = local read "Ring 27"() -> (w1148:u16)
    n1770 = local read "Ring 33"() -> (w1147:u16)
    n1771 = local read "Ring 21"() -> (w1154:u16)
    n1772 = local read "Ring 27"() -> (w1153:u16)
    n1773 = local read "Ring 33"() -> (w1152:u16)
    n1774 = local read "Ring 3"() -> (w1142:u16)
    n1775 = local read "Ring 9"() -> (w1141:u16)
    n1776 = local read "Ring 9"() -> (w1146:u16)
    n1777 = local read "Ring 39"() -> (w1151:u16)
    n1778 = Equal?(x=w855, y=u16 2) -> (x = y?=w871:bool)
    n1779 = Equal?(x=w1764, y=u16 2) -> (x = y?=w1748:bool)
    n1780 = Equal?(x=w854, y=u16 2) -> (x = y?=w868:bool)
    n1781 = Equal?(x=w1765, y=u16 2) -> (x = y?=w1751:bool)
    n1782 = Equal?(x=w853, y=u16 2) -> (x = y?=w869:bool)
    n1783 = Equal?(x=w1766, y=u16 2) -> (x = y?=w1750:bool)
    n1784 = Equal?(x=w852, y=u16 2) -> (x = y?=w870:bool)
    n1785 = Equal?(x=w1767, y=u16 2) -> (x = y?=w1749:bool)
    n1786 = Equal?(x=w859, y=u16 2) -> (x = y?=w879:bool)
    n1787 = Equal?(x=w1760, y=u16 2) -> (x = y?=w1740:bool)
    n1788 = Equal?(x=w858, y=u16 2) -> (x = y?=w876:bool)
    n1789 = Equal?(x=w1761, y=u16 2) -> (x = y?=w1743:bool)
    n1790 = Equal?(x=w857, y=u16 2) -> (x = y?=w877:bool)
    n1791 = Equal?(x=w1762, y=u16 2) -> (x = y?=w1742:bool)
    n1792 = Equal?(x=w856, y=u16 2) -> (x = y?=w878:bool)
    n1793 = Equal?(x=w1763, y=u16 2) -> (x = y?=w1741:bool)
    n1794 = Equal?(x=w863, y=u16 2) -> (x = y?=w887:bool)
    n1795 = Equal?(x=w1756, y=u16 2) -> (x = y?=w1732:bool)
    n1796 = Equal?(x=w862, y=u16 2) -> (x = y?=w884:bool)
    n1797 = Equal?(x=w1757, y=u16 2) -> (x = y?=w1735:bool)
    n1798 = Equal?(x=w861, y=u16 2) -> (x = y?=w885:bool)
    n1799 = Equal?(x=w1758, y=u16 2) -> (x = y?=w1734:bool)
    n1800 = Equal?(x=w860, y=u16 2) -> (x = y?=w886:bool)
    n1801 = Equal?(x=w1759, y=u16 2) -> (x = y?=w1733:bool)
    n1802 = Compound Arithmetic op=AND(w871, w868, w869, w870) -> (w734:bool)
    n1803 = Compound Arithmetic op=AND(w1748, w1751, w1750, w1749) -> (w1885:bool)
    n1804 = Compound Arithmetic op=AND(w879, w876, w877, w878) -> (w733:bool)
    n1805 = Compound Arithmetic op=AND(w1740, w1743, w1742, w1741) -> (w1886:bool)
    n1806 = Compound Arithmetic op=AND(w887, w884, w885, w886) -> (w732:bool)
    n1807 = Compound Arithmetic op=AND(w1732, w1735, w1734, w1733) -> (w1887:bool)
    n1808 = Equal?(x=w1142, y=u16 2) -> (x = y?=w1158:bool)
    n1809 = Equal?(x=w1141, y=u16 2) -> (x = y?=w1157:bool)
    n1810 = Equal?(x=w1140, y=u16 2) -> (x = y?=w1156:bool)
    n1811 = Equal?(x=w1139, y=u16 2) -> (x = y?=w1155:bool)
    n1812 = Equal?(x=w1146, y=u16 2) -> (x = y?=w1166:bool)
    n1813 = Equal?(x=w1145, y=u16 2) -> (x = y?=w1165:bool)
    n1814 = Equal?(x=w1144, y=u16 2) -> (x = y?=w1164:bool)
    n1815 = Equal?(x=w1143, y=u16 2) -> (x = y?=w1163:bool)
    n1816 = Equal?(x=w1150, y=u16 2) -> (x = y?=w1174:bool)
    n1817 = Equal?(x=w1149, y=u16 2) -> (x = y?=w1173:bool)
    n1818 = Equal?(x=w1148, y=u16 2) -> (x = y?=w1172:bool)
    n1819 = Equal?(x=w1147, y=u16 2) -> (x = y?=w1171:bool)
    n1820 = Equal?(x=w1154, y=u16 2) -> (x = y?=w1182:bool)
    n1821 = Equal?(x=w1153, y=u16 2) -> (x = y?=w1181:bool)
    n1822 = Equal?(x=w1152, y=u16 2) -> (x = y?=w1180:bool)
    n1823 = Equal?(x=w1151, y=u16 2) -> (x = y?=w1179:bool)
    n1824 = Compound Arithmetic op=AND(w1158, w1157, w1156, w1155) -> (w1295:bool)
    n1825 = Compound Arithmetic op=AND(w1166, w1165, w1164, w1163) -> (w1296:bool)
    n1826 = Compound Arithmetic op=AND(w1174, w1173, w1172, w1171) -> (w1297:bool)
    n1827 = Compound Arithmetic op=AND(w1182, w1181, w1180, w1179) -> (w1298:bool)
    n1828 = local read "Ring 28"() -> (w819:u16)
    n1829 = local read "Ring 28"() -> (w1800:u16)
    n1830 = local read "Ring 27"() -> (w818:u16)
    n1831 = local read "Ring 27"() -> (w1801:u16)
    n1832 = local read "Ring 26"() -> (w817:u16)
    n1833 = local read "Ring 26"() -> (w1802:u16)
    n1834 = local read "Ring 25"() -> (w816:u16)
    n1835 = local read "Ring 25"() -> (w1803:u16)
    n1836 = local read "Ring 29"() -> (w823:u16)
    n1837 = local read "Ring 29"() -> (w1796:u16)
    n1838 = local read "Ring 28"() -> (w822:u16)
    n1839 = local read "Ring 28"() -> (w1797:u16)
    n1840 = local read "Ring 27"() -> (w821:u16)
    n1841 = local read "Ring 27"() -> (w1798:u16)
    n1842 = local read "Ring 26"() -> (w820:u16)
    n1843 = local read "Ring 26"() -> (w1799:u16)
    n1844 = local read "Ring 30"() -> (w827:u16)
    n1845 = local read "Ring 30"() -> (w1792:u16)
    n1846 = local read "Ring 29"() -> (w826:u16)
    n1847 = local read "Ring 29"() -> (w1793:u16)
    n1848 = local read "Ring 28"() -> (w825:u16)
    n1849 = local read "Ring 28"() -> (w1794:u16)
    n1850 = local read "Ring 27"() -> (w824:u16)
    n1851 = local read "Ring 27"() -> (w1795:u16)
    n1852 = local read "Ring 14"() -> (w1187:u16)
    n1853 = local read "Ring 20"() -> (w1186:u16)
    n1854 = local read "Ring 14"() -> (w1192:u16)
    n1855 = local read "Ring 20"() -> (w1191:u16)
    n1856 = local read "Ring 26"() -> (w1190:u16)
    n1857 = local read "Ring 14"() -> (w1197:u16)
    n1858 = local read "Ring 20"() -> (w1196:u16)
    n1859 = local read "Ring 26"() -> (w1195:u16)
    n1860 = local read "Ring 32"() -> (w1194:u16)
    n1861 = local read "Ring 20"() -> (w1201:u16)
    n1862 = local read "Ring 26"() -> (w1200:u16)
    n1863 = local read "Ring 32"() -> (w1199:u16)
    n1864 = Equal?(x=w819, y=u16 2) -> (x = y?=w835:bool)
    n1865 = Equal?(x=w1800, y=u16 2) -> (x = y?=w1784:bool)
    n1866 = Equal?(x=w818, y=u16 2) -> (x = y?=w832:bool)
    n1867 = Equal?(x=w1801, y=u16 2) -> (x = y?=w1787:bool)
    n1868 = Equal?(x=w817, y=u16 2) -> (x = y?=w833:bool)
    n1869 = Equal?(x=w1802, y=u16 2) -> (x = y?=w1786:bool)
    n1870 = Equal?(x=w816, y=u16 2) -> (x = y?=w834:bool)
    n1871 = Equal?(x=w1803, y=u16 2) -> (x = y?=w1785:bool)
    n1872 = Equal?(x=w823, y=u16 2) -> (x = y?=w843:bool)
    n1873 = Equal?(x=w1796, y=u16 2) -> (x = y?=w1776:bool)
    n1874 = Equal?(x=w822, y=u16 2) -> (x = y?=w840:bool)
    n1875 = Equal?(x=w1797, y=u16 2) -> (x = y?=w1779:bool)
    n1876 = Equal?(x=w821, y=u16 2) -> (x = y?=w841:bool)
    n1877 = Equal?(x=w1798, y=u16 2) -> (x = y?=w1778:bool)
    n1878 = Equal?(x=w820, y=u16 2) -> (x = y?=w842:bool)
    n1879 = Equal?(x=w1799, y=u16 2) -> (x = y?=w1777:bool)
    n1880 = Equal?(x=w827, y=u16 2) -> (x = y?=w851:bool)
    n1881 = Equal?(x=w1792, y=u16 2) -> (x = y?=w1768:bool)
    n1882 = Equal?(x=w826, y=u16 2) -> (x = y?=w848:bool)
    n1883 = Equal?(x=w1793, y=u16 2) -> (x = y?=w1771:bool)
    n1884 = Equal?(x=w825, y=u16 2) -> (x = y?=w849:bool)
    n1885 = Equal?(x=w1794, y=u16 2) -> (x = y?=w1770:bool)
    n1886 = Equal?(x=w824, y=u16 2) -> (x = y?=w850:bool)
    n1887 = Equal?(x=w1795, y=u16 2) -> (x = y?=w1769:bool)
    n1888 = local read "Ring 2"() -> (w1189:u16)
    n1889 = local read "Ring 8"() -> (w1188:u16)
    n1890 = local read "Ring 8"() -> (w1193:u16)
    n1891 = local read "Ring 38"() -> (w1198:u16)
    n1892 = Compound Arithmetic op=AND(w835, w832, w833, w834) -> (w731:bool)
    n1893 = Compound Arithmetic op=AND(w1784, w1787, w1786, w1785) -> (w1888:bool)
    n1894 = Compound Arithmetic op=AND(w843, w840, w841, w842) -> (w730:bool)
    n1895 = Compound Arithmetic op=AND(w1776, w1779, w1778, w1777) -> (w1889:bool)
    n1896 = Compound Arithmetic op=AND(w851, w848, w849, w850) -> (w729:bool)
    n1897 = Compound Arithmetic op=AND(w1768, w1771, w1770, w1769) -> (w1890:bool)
    n1898 = Equal?(x=w1189, y=u16 2) -> (x = y?=w1205:bool)
    n1899 = Equal?(x=w1188, y=u16 2) -> (x = y?=w1204:bool)
    n1900 = Equal?(x=w1187, y=u16 2) -> (x = y?=w1203:bool)
    n1901 = Equal?(x=w1186, y=u16 2) -> (x = y?=w1202:bool)
    n1902 = Equal?(x=w1193, y=u16 2) -> (x = y?=w1213:bool)
    n1903 = Equal?(x=w1192, y=u16 2) -> (x = y?=w1212:bool)
    n1904 = Equal?(x=w1191, y=u16 2) -> (x = y?=w1211:bool)
    n1905 = Equal?(x=w1190, y=u16 2) -> (x = y?=w1210:bool)
    n1906 = Equal?(x=w1197, y=u16 2) -> (x = y?=w1221:bool)
    n1907 = Equal?(x=w1196, y=u16 2) -> (x = y?=w1220:bool)
    n1908 = Equal?(x=w1195, y=u16 2) -> (x = y?=w1219:bool)
    n1909 = Equal?(x=w1194, y=u16 2) -> (x = y?=w1218:bool)
    n1910 = Equal?(x=w1201, y=u16 2) -> (x = y?=w1229:bool)
    n1911 = Equal?(x=w1200, y=u16 2) -> (x = y?=w1228:bool)
    n1912 = Equal?(x=w1199, y=u16 2) -> (x = y?=w1227:bool)
    n1913 = Equal?(x=w1198, y=u16 2) -> (x = y?=w1226:bool)
    n1914 = local read "Ring 34"() -> (w783:u16)
    n1915 = local read "Ring 34"() -> (w1836:u16)
    n1916 = local read "Ring 33"() -> (w782:u16)
    n1917 = local read "Ring 33"() -> (w1837:u16)
    n1918 = local read "Ring 32"() -> (w781:u16)
    n1919 = local read "Ring 32"() -> (w1838:u16)
    n1920 = local read "Ring 31"() -> (w780:u16)
    n1921 = local read "Ring 31"() -> (w1839:u16)
    n1922 = local read "Ring 35"() -> (w787:u16)
    n1923 = local read "Ring 35"() -> (w1832:u16)
    n1924 = local read "Ring 34"() -> (w786:u16)
    n1925 = local read "Ring 34"() -> (w1833:u16)
    n1926 = local read "Ring 33"() -> (w785:u16)
    n1927 = local read "Ring 33"() -> (w1834:u16)
    n1928 = local read "Ring 32"() -> (w784:u16)
    n1929 = local read "Ring 32"() -> (w1835:u16)
    n1930 = local read "Ring 36"() -> (w791:u16)
    n1931 = local read "Ring 36"() -> (w1828:u16)
    n1932 = local read "Ring 35"() -> (w790:u16)
    n1933 = local read "Ring 35"() -> (w1829:u16)
    n1934 = local read "Ring 34"() -> (w789:u16)
    n1935 = local read "Ring 34"() -> (w1830:u16)
    n1936 = local read "Ring 33"() -> (w788:u16)
    n1937 = local read "Ring 33"() -> (w1831:u16)
    n1938 = Compound Arithmetic op=AND(w1205, w1204, w1203, w1202) -> (w1300:bool)
    n1939 = Compound Arithmetic op=AND(w1213, w1212, w1211, w1210) -> (w1301:bool)
    n1940 = Compound Arithmetic op=AND(w1221, w1220, w1219, w1218) -> (w1302:bool)
    n1941 = Compound Arithmetic op=AND(w1229, w1228, w1227, w1226) -> (w1303:bool)
    n1942 = Equal?(x=w783, y=u16 2) -> (x = y?=w799:bool)
    n1943 = Equal?(x=w1836, y=u16 2) -> (x = y?=w1820:bool)
    n1944 = Equal?(x=w782, y=u16 2) -> (x = y?=w796:bool)
    n1945 = Equal?(x=w1837, y=u16 2) -> (x = y?=w1823:bool)
    n1946 = Equal?(x=w781, y=u16 2) -> (x = y?=w797:bool)
    n1947 = Equal?(x=w1838, y=u16 2) -> (x = y?=w1822:bool)
    n1948 = Equal?(x=w780, y=u16 2) -> (x = y?=w798:bool)
    n1949 = Equal?(x=w1839, y=u16 2) -> (x = y?=w1821:bool)
    n1950 = Equal?(x=w787, y=u16 2) -> (x = y?=w807:bool)
    n1951 = Equal?(x=w1832, y=u16 2) -> (x = y?=w1812:bool)
    n1952 = Equal?(x=w786, y=u16 2) -> (x = y?=w804:bool)
    n1953 = Equal?(x=w1833, y=u16 2) -> (x = y?=w1815:bool)
    n1954 = Equal?(x=w785, y=u16 2) -> (x = y?=w805:bool)
    n1955 = Equal?(x=w1834, y=u16 2) -> (x = y?=w1814:bool)
    n1956 = Equal?(x=w784, y=u16 2) -> (x = y?=w806:bool)
    n1957 = Equal?(x=w1835, y=u16 2) -> (x = y?=w1813:bool)
    n1958 = Equal?(x=w791, y=u16 2) -> (x = y?=w815:bool)
    n1959 = Equal?(x=w1828, y=u16 2) -> (x = y?=w1804:bool)
    n1960 = Equal?(x=w790, y=u16 2) -> (x = y?=w812:bool)
    n1961 = Equal?(x=w1829, y=u16 2) -> (x = y?=w1807:bool)
    n1962 = Equal?(x=w789, y=u16 2) -> (x = y?=w813:bool)
    n1963 = Equal?(x=w1830, y=u16 2) -> (x = y?=w1806:bool)
    n1964 = Equal?(x=w788, y=u16 2) -> (x = y?=w814:bool)
    n1965 = Equal?(x=w1831, y=u16 2) -> (x = y?=w1805:bool)
    n1966 = Compound Arithmetic op=AND(w799, w796, w797, w798) -> (w728:bool)
    n1967 = Compound Arithmetic op=AND(w1820, w1823, w1822, w1821) -> (w1891:bool)
    n1968 = Compound Arithmetic op=AND(w807, w804, w805, w806) -> (w727:bool)
    n1969 = Compound Arithmetic op=AND(w1812, w1815, w1814, w1813) -> (w1892:bool)
    n1970 = Compound Arithmetic op=AND(w815, w812, w813, w814) -> (w726:bool)
    n1971 = Compound Arithmetic op=AND(w1804, w1807, w1806, w1805) -> (w1893:bool)
    n1972 = local read "Ring 13"() -> (w1234:u16)
    n1973 = local read "Ring 19"() -> (w1233:u16)
    n1974 = local read "Ring 13"() -> (w1239:u16)
    n1975 = local read "Ring 19"() -> (w1238:u16)
    n1976 = local read "Ring 25"() -> (w1237:u16)
    n1977 = local read "Ring 13"() -> (w1244:u16)
    n1978 = local read "Ring 19"() -> (w1243:u16)
    n1979 = local read "Ring 25"() -> (w1242:u16)
    n1980 = local read "Ring 31"() -> (w1241:u16)
    n1981 = local read "Ring 19"() -> (w1248:u16)
    n1982 = local read "Ring 25"() -> (w1247:u16)
    n1983 = local read "Ring 31"() -> (w1246:u16)
    n1984 = local read "Ring 1"() -> (w1236:u16)
    n1985 = local read "Ring 7"() -> (w1235:u16)
    n1986 = local read "Ring 7"() -> (w1240:u16)
    n1987 = local read "Ring 37"() -> (w1245:u16)
    n1988 = local read "Ring 40"() -> (w747:u16)
    n1989 = local read "Ring 40"() -> (w1872:u16)
    n1990 = local read "Ring 39"() -> (w746:u16)
    n1991 = local read "Ring 39"() -> (w1873:u16)
    n1992 = local read "Ring 38"() -> (w745:u16)
    n1993 = local read "Ring 38"() -> (w1874:u16)
    n1994 = local read "Ring 37"() -> (w744:u16)
    n1995 = local read "Ring 37"() -> (w1875:u16)
    n1996 = local read "Ring 41"() -> (w751:u16)
    n1997 = local read "Ring 41"() -> (w1868:u16)
    n1998 = local read "Ring 40"() -> (w750:u16)
    n1999 = local read "Ring 40"() -> (w1869:u16)
    n2000 = local read "Ring 39"() -> (w749:u16)
    n2001 = local read "Ring 39"() -> (w1870:u16)
    n2002 = local read "Ring 38"() -> (w748:u16)
    n2003 = local read "Ring 38"() -> (w1871:u16)
    n2004 = local read "Ring 42"() -> (w755:u16)
    n2005 = local read "Ring 42"() -> (w1864:u16)
    n2006 = local read "Ring 41"() -> (w754:u16)
    n2007 = local read "Ring 41"() -> (w1865:u16)
    n2008 = local read "Ring 40"() -> (w753:u16)
    n2009 = local read "Ring 40"() -> (w1866:u16)
    n2010 = local read "Ring 39"() -> (w752:u16)
    n2011 = local read "Ring 39"() -> (w1867:u16)
    n2012 = Equal?(x=w1236, y=u16 2) -> (x = y?=w1252:bool)
    n2013 = Equal?(x=w1235, y=u16 2) -> (x = y?=w1251:bool)
    n2014 = Equal?(x=w1234, y=u16 2) -> (x = y?=w1250:bool)
    n2015 = Equal?(x=w1233, y=u16 2) -> (x = y?=w1249:bool)
    n2016 = Equal?(x=w1240, y=u16 2) -> (x = y?=w1260:bool)
    n2017 = Equal?(x=w1239, y=u16 2) -> (x = y?=w1259:bool)
    n2018 = Equal?(x=w1238, y=u16 2) -> (x = y?=w1258:bool)
    n2019 = Equal?(x=w1237, y=u16 2) -> (x = y?=w1257:bool)
    n2020 = Equal?(x=w1244, y=u16 2) -> (x = y?=w1268:bool)
    n2021 = Equal?(x=w1243, y=u16 2) -> (x = y?=w1267:bool)
    n2022 = Equal?(x=w1242, y=u16 2) -> (x = y?=w1266:bool)
    n2023 = Equal?(x=w1241, y=u16 2) -> (x = y?=w1265:bool)
    n2024 = Equal?(x=w1248, y=u16 2) -> (x = y?=w1276:bool)
    n2025 = Equal?(x=w1247, y=u16 2) -> (x = y?=w1275:bool)
    n2026 = Equal?(x=w1246, y=u16 2) -> (x = y?=w1274:bool)
    n2027 = Equal?(x=w1245, y=u16 2) -> (x = y?=w1273:bool)
    n2028 = Compound Arithmetic op=AND(w1252, w1251, w1250, w1249) -> (w1304:bool)
    n2029 = Compound Arithmetic op=AND(w1260, w1259, w1258, w1257) -> (w1305:bool)
    n2030 = Compound Arithmetic op=AND(w1268, w1267, w1266, w1265) -> (w1306:bool)
    n2031 = Compound Arithmetic op=AND(w1276, w1275, w1274, w1273) -> (w1307:bool)
    n2032 = Equal?(x=w747, y=u16 2) -> (x = y?=w763:bool)
    n2033 = Equal?(x=w1872, y=u16 2) -> (x = y?=w1856:bool)
    n2034 = Equal?(x=w746, y=u16 2) -> (x = y?=w760:bool)
    n2035 = Equal?(x=w1873, y=u16 2) -> (x = y?=w1859:bool)
    n2036 = Equal?(x=w745, y=u16 2) -> (x = y?=w761:bool)
    n2037 = Equal?(x=w1874, y=u16 2) -> (x = y?=w1858:bool)
    n2038 = Equal?(x=w744, y=u16 2) -> (x = y?=w762:bool)
    n2039 = Equal?(x=w1875, y=u16 2) -> (x = y?=w1857:bool)
    n2040 = Equal?(x=w751, y=u16 2) -> (x = y?=w771:bool)
    n2041 = Equal?(x=w1868, y=u16 2) -> (x = y?=w1848:bool)
    n2042 = Equal?(x=w750, y=u16 2) -> (x = y?=w768:bool)
    n2043 = Equal?(x=w1869, y=u16 2) -> (x = y?=w1851:bool)
    n2044 = Equal?(x=w749, y=u16 2) -> (x = y?=w769:bool)
    n2045 = Equal?(x=w1870, y=u16 2) -> (x = y?=w1850:bool)
    n2046 = Equal?(x=w748, y=u16 2) -> (x = y?=w770:bool)
    n2047 = Equal?(x=w1871, y=u16 2) -> (x = y?=w1849:bool)
    n2048 = Equal?(x=w755, y=u16 2) -> (x = y?=w779:bool)
    n2049 = Equal?(x=w1864, y=u16 2) -> (x = y?=w1840:bool)
    n2050 = Equal?(x=w754, y=u16 2) -> (x = y?=w776:bool)
    n2051 = Equal?(x=w1865, y=u16 2) -> (x = y?=w1843:bool)
    n2052 = Equal?(x=w753, y=u16 2) -> (x = y?=w777:bool)
    n2053 = Equal?(x=w1866, y=u16 2) -> (x = y?=w1842:bool)
    n2054 = Equal?(x=w752, y=u16 2) -> (x = y?=w778:bool)
    n2055 = Equal?(x=w1867, y=u16 2) -> (x = y?=w1841:bool)
    n2056 = Compound Arithmetic op=AND(w763, w760, w761, w762) -> (w725:bool)
    n2057 = Compound Arithmetic op=AND(w1856, w1859, w1858, w1857) -> (w1894:bool)
    n2058 = Compound Arithmetic op=AND(w771, w768, w769, w770) -> (w724:bool)
    n2059 = Compound Arithmetic op=AND(w1848, w1851, w1850, w1849) -> (w1895:bool)
    n2060 = Compound Arithmetic op=AND(w779, w776, w777, w778) -> (w723:bool)
    n2061 = Compound Arithmetic op=AND(w1840, w1843, w1842, w1841) -> (w1896:bool)
    n2062 = Compound Arithmetic op=OR(w1284, w1285, w1286, w1287, w1288, w1289, w1290, w1299, w1291, w1292, w1293, w1294, w1295, w1296, w1297, w1298, w1300, w1301, w1302, w1303, w1304, w1305, w1306, w1307) -> (w1308:bool)
    n2063 = Compound Arithmetic op=OR(w743, w742, w741, w740, w739, w738, w737, w736, w735, w734, w733, w732, w731, w730, w729, w728, w727, w726, w725, w724, w723) -> (w972:bool)
    n2064 = Compound Arithmetic op=OR(w1876, w1877, w1878, w1879, w1880, w1881, w1882, w1883, w1884, w1885, w1886, w1887, w1888, w1889, w1890, w1891, w1892, w1893, w1894, w1895, w1896) -> (w1647:bool)
    n2065 = case shown="True" w972 {
      selector: w972 -> [_ w2200]
      frame False {
      }
      frame True {
        n2066 = property on="Player Rojo" class="DigNum (strict)"() -> ("Value"=w2202:dbl)  [unwired: 2 in, 2 out]
        n2067 = Increment(x=w2202) -> (x+1=w2201:dbl)
        n2068 = call "Display Message to User5"("Enable"=w2200) -> ()  [unwired: 9 in, 2 out]
        n2069 = property on="Player Rojo" class="DigNum (strict)"("Value"=w2201) -> ()  [unwired: 2 in, 2 out]
      }
    }
    n2070 = case shown="True" w1647 {
      selector: w1647 -> [_ w2209]
      frame False {
      }
      frame True {
        n2071 = property on="Player Rojo" class="DigNum (strict)"() -> ("Value"=w2211:dbl)  [unwired: 2 in, 2 out]
        n2072 = Increment(x=w2211) -> (x+1=w2210:dbl)
        n2073 = call "Display Message to User2"("Enable"=w2209) -> ()  [unwired: 9 in, 2 out]
        n2074 = property on="Player Rojo" class="DigNum (strict)"("Value"=w2210) -> ()  [unwired: 2 in, 2 out]
      }
    }
    n2075 = case shown="True" w1308 {
      selector: w1308 -> [_ w2203]
      frame False {
      }
      frame True {
        n2076 = property on="Player Rojo" class="DigNum (strict)"() -> ("Value"=w2205:dbl)  [unwired: 2 in, 2 out]
        n2077 = Increment(x=w2205) -> (x+1=w2204:dbl)
        n2078 = call "Display Message to User4"("Enable"=w2203) -> ()  [unwired: 9 in, 2 out]
        n2079 = property on="Player Rojo" class="DigNum (strict)"("Value"=w2204) -> ()  [unwired: 2 in, 2 out]
      }
    }
    n2080 = local read "Ring 19"() -> (w582:u16)
    n2081 = local read "Ring 14"() -> (w584:u16)
    n2082 = local read "Ring 10"() -> (w568:u16)
    n2083 = local read "Ring 15"() -> (w567:u16)
    n2084 = local read "Ring 20"() -> (w566:u16)
    n2085 = local read "Ring 10"() -> (w599:u16)
    n2086 = local read "Ring 15"() -> (w602:u16)
    n2087 = local read "Ring 20"() -> (w601:u16)
    n2088 = local read "Ring 25"() -> (w600:u16)
    n2089 = local read "Ring 9"() -> (w586:u16)
    n2090 = local read "Ring 4"() -> (w588:u16)
    n2091 = local read "Ring 5"() -> (w569:u16)
    n2092 = Equal?(x=w582, y=u16 2) -> (x = y?=w581:bool)
    n2093 = Equal?(x=w584, y=u16 2) -> (x = y?=w580:bool)
    n2094 = Equal?(x=w586, y=u16 2) -> (x = y?=w579:bool)
    n2095 = Equal?(x=w588, y=u16 2) -> (x = y?=w578:bool)
    n2096 = Equal?(x=w569, y=u16 2) -> (x = y?=w573:bool)
    n2097 = Equal?(x=w568, y=u16 2) -> (x = y?=w572:bool)
    n2098 = Equal?(x=w567, y=u16 2) -> (x = y?=w571:bool)
    n2099 = Equal?(x=w566, y=u16 2) -> (x = y?=w570:bool)
    n2100 = Equal?(x=w599, y=u16 2) -> (x = y?=w595:bool)
    n2101 = Equal?(x=w602, y=u16 2) -> (x = y?=w596:bool)
    n2102 = Equal?(x=w601, y=u16 2) -> (x = y?=w597:bool)
    n2103 = Equal?(x=w600, y=u16 2) -> (x = y?=w598:bool)
    n2104 = local read "Ring 10"() -> (w547:u16)
    n2105 = local read "Ring 17"() -> (w545:u16)
    n2106 = local read "Ring 24"() -> (w543:u16)
    n2107 = local read "Ring 16"() -> (w564:u16)
    n2108 = local read "Ring 23"() -> (w565:u16)
    n2109 = local read "Ring 16"() -> (w529:u16)
    n2110 = local read "Ring 23"() -> (w530:u16)
    n2111 = local read "Ring 30"() -> (w531:u16)
    n2112 = local read "Ring 3"() -> (w549:u16)
    n2113 = local read "Ring 2"() -> (w562:u16)
    n2114 = local read "Ring 9"() -> (w563:u16)
    n2115 = local read "Ring 9"() -> (w532:u16)
    n2116 = Compound Arithmetic op=AND(w581, w580, w579, w578) -> (w711:bool)
    n2117 = Compound Arithmetic op=AND(w573, w572, w571, w570) -> (w712:bool)
    n2118 = Compound Arithmetic op=AND(w595, w596, w597, w598) -> (w713:bool)
    n2119 = Equal?(x=w549, y=u16 2) -> (x = y?=w550:bool)
    n2120 = Equal?(x=w547, y=u16 2) -> (x = y?=w551:bool)
    n2121 = Equal?(x=w545, y=u16 2) -> (x = y?=w552:bool)
    n2122 = Equal?(x=w543, y=u16 2) -> (x = y?=w553:bool)
    n2123 = Equal?(x=w562, y=u16 2) -> (x = y?=w558:bool)
    n2124 = Equal?(x=w563, y=u16 2) -> (x = y?=w559:bool)
    n2125 = Equal?(x=w564, y=u16 2) -> (x = y?=w560:bool)
    n2126 = Equal?(x=w565, y=u16 2) -> (x = y?=w561:bool)
    n2127 = Equal?(x=w532, y=u16 2) -> (x = y?=w536:bool)
    n2128 = Equal?(x=w529, y=u16 2) -> (x = y?=w535:bool)
    n2129 = Equal?(x=w530, y=u16 2) -> (x = y?=w534:bool)
    n2130 = Equal?(x=w531, y=u16 2) -> (x = y?=w533:bool)
    n2131 = local read "Ring 11"() -> (w623:u16)
    n2132 = local read "Ring 16"() -> (w624:u16)
    n2133 = local read "Ring 16"() -> (w611:u16)
    n2134 = local read "Ring 21"() -> (w612:u16)
    n2135 = local read "Ring 26"() -> (w613:u16)
    n2136 = local read "Ring 6"() -> (w634:u16)
    n2137 = local read "Ring 11"() -> (w635:u16)
    n2138 = local read "Ring 16"() -> (w636:u16)
    n2139 = local read "Ring 21"() -> (w637:u16)
    n2140 = local read "Ring 21"() -> (w625:u16)
    n2141 = local read "Ring 26"() -> (w626:u16)
    n2142 = local read "Ring 31"() -> (w614:u16)
    n2143 = Compound Arithmetic op=AND(w550, w551, w552, w553) -> (w420:bool)
    n2144 = Compound Arithmetic op=AND(w558, w559, w560, w561) -> (w419:bool)
    n2145 = Compound Arithmetic op=AND(w536, w535, w534, w533) -> (w418:bool)
    n2146 = Equal?(x=w634, y=u16 2) -> (x = y?=w638:bool)
    n2147 = Equal?(x=w635, y=u16 2) -> (x = y?=w631:bool)
    n2148 = Equal?(x=w636, y=u16 2) -> (x = y?=w632:bool)
    n2149 = Equal?(x=w637, y=u16 2) -> (x = y?=w633:bool)
    n2150 = Equal?(x=w623, y=u16 2) -> (x = y?=w618:bool)
    n2151 = Equal?(x=w624, y=u16 2) -> (x = y?=w617:bool)
    n2152 = Equal?(x=w625, y=u16 2) -> (x = y?=w616:bool)
    n2153 = Equal?(x=w626, y=u16 2) -> (x = y?=w615:bool)
    n2154 = Equal?(x=w611, y=u16 2) -> (x = y?=w607:bool)
    n2155 = Equal?(x=w612, y=u16 2) -> (x = y?=w608:bool)
    n2156 = Equal?(x=w613, y=u16 2) -> (x = y?=w609:bool)
    n2157 = Equal?(x=w614, y=u16 2) -> (x = y?=w610:bool)
    n2158 = local read "Ring 15"() -> (w507:u16)
    n2159 = local read "Ring 15"() -> (w520:u16)
    n2160 = local read "Ring 22"() -> (w519:u16)
    n2161 = local read "Ring 29"() -> (w518:u16)
    n2162 = local read "Ring 1"() -> (w497:u16)
    n2163 = local read "Ring 15"() -> (w495:u16)
    n2164 = local read "Ring 22"() -> (w494:u16)
    n2165 = local read "Ring 8"() -> (w508:u16)
    n2166 = local read "Ring 22"() -> (w506:u16)
    n2167 = local read "Ring 29"() -> (w505:u16)
    n2168 = local read "Ring 36"() -> (w517:u16)
    n2169 = local read "Ring 8"() -> (w496:u16)
    n2170 = Compound Arithmetic op=AND(w638, w631, w632, w633) -> (w714:bool)
    n2171 = Compound Arithmetic op=AND(w618, w617, w616, w615) -> (w715:bool)
    n2172 = Compound Arithmetic op=AND(w607, w608, w609, w610) -> (w716:bool)
    n2173 = Equal?(x=w497, y=u16 2) -> (x = y?=w493:bool)
    n2174 = Equal?(x=w496, y=u16 2) -> (x = y?=w500:bool)
    n2175 = Equal?(x=w495, y=u16 2) -> (x = y?=w499:bool)
    n2176 = Equal?(x=w494, y=u16 2) -> (x = y?=w498:bool)
    n2177 = Equal?(x=w508, y=u16 2) -> (x = y?=w513:bool)
    n2178 = Equal?(x=w507, y=u16 2) -> (x = y?=w514:bool)
    n2179 = Equal?(x=w506, y=u16 2) -> (x = y?=w515:bool)
    n2180 = Equal?(x=w505, y=u16 2) -> (x = y?=w516:bool)
    n2181 = Equal?(x=w520, y=u16 2) -> (x = y?=w524:bool)
    n2182 = Equal?(x=w519, y=u16 2) -> (x = y?=w523:bool)
    n2183 = Equal?(x=w518, y=u16 2) -> (x = y?=w522:bool)
    n2184 = Equal?(x=w517, y=u16 2) -> (x = y?=w521:bool)
    n2185 = local read "Ring 17"() -> (w659:u16)
    n2186 = local read "Ring 22"() -> (w660:u16)
    n2187 = local read "Ring 27"() -> (w661:u16)
    n2188 = local read "Ring 32"() -> (w662:u16)
    n2189 = local read "Ring 22"() -> (w655:u16)
    n2190 = local read "Ring 27"() -> (w656:u16)
    n2191 = local read "Ring 32"() -> (w657:u16)
    n2192 = local read "Ring 37"() -> (w658:u16)
    n2193 = local read "Ring 12"() -> (w651:u16)
    n2194 = local read "Ring 17"() -> (w652:u16)
    n2195 = local read "Ring 22"() -> (w653:u16)
    n2196 = local read "Ring 27"() -> (w654:u16)
    n2197 = Compound Arithmetic op=AND(w493, w500, w499, w498) -> (w417:bool)
    n2198 = Compound Arithmetic op=AND(w513, w514, w515, w516) -> (w416:bool)
    n2199 = Compound Arithmetic op=AND(w524, w523, w522, w521) -> (w415:bool)
    n2200 = local read "Ring 14"() -> (w472:u16)
    n2201 = local read "Ring 21"() -> (w471:u16)
    n2202 = local read "Ring 28"() -> (w470:u16)
    n2203 = local read "Ring 35"() -> (w469:u16)
    n2204 = local read "Ring 21"() -> (w476:u16)
    n2205 = local read "Ring 28"() -> (w475:u16)
    n2206 = local read "Ring 35"() -> (w474:u16)
    n2207 = local read "Ring 42"() -> (w473:u16)
    n2208 = local read "Ring 14"() -> (w479:u16)
    n2209 = local read "Ring 21"() -> (w478:u16)
    n2210 = local read "Ring 28"() -> (w477:u16)
    n2211 = local read "Ring 7"() -> (w480:u16)
    n2212 = Equal?(x=w659, y=u16 2) -> (x = y?=w647:bool)
    n2213 = Equal?(x=w660, y=u16 2) -> (x = y?=w650:bool)
    n2214 = Equal?(x=w661, y=u16 2) -> (x = y?=w649:bool)
    n2215 = Equal?(x=w662, y=u16 2) -> (x = y?=w648:bool)
    n2216 = Equal?(x=w655, y=u16 2) -> (x = y?=w646:bool)
    n2217 = Equal?(x=w656, y=u16 2) -> (x = y?=w643:bool)
    n2218 = Equal?(x=w657, y=u16 2) -> (x = y?=w644:bool)
    n2219 = Equal?(x=w658, y=u16 2) -> (x = y?=w645:bool)
    n2220 = Equal?(x=w651, y=u16 2) -> (x = y?=w639:bool)
    n2221 = Equal?(x=w652, y=u16 2) -> (x = y?=w642:bool)
    n2222 = Equal?(x=w653, y=u16 2) -> (x = y?=w641:bool)
    n2223 = Equal?(x=w654, y=u16 2) -> (x = y?=w640:bool)
    n2224 = Compound Arithmetic op=AND(w647, w650, w649, w648) -> (w718:bool)
    n2225 = Compound Arithmetic op=AND(w646, w643, w644, w645) -> (w719:bool)
    n2226 = Compound Arithmetic op=AND(w639, w642, w641, w640) -> (w717:bool)
    n2227 = local read "Ring 18"() -> (w707:u16)
    n2228 = local read "Ring 23"() -> (w708:u16)
    n2229 = local read "Ring 28"() -> (w709:u16)
    n2230 = local read "Ring 33"() -> (w710:u16)
    n2231 = local read "Ring 23"() -> (w703:u16)
    n2232 = local read "Ring 28"() -> (w704:u16)
    n2233 = local read "Ring 33"() -> (w705:u16)
    n2234 = local read "Ring 38"() -> (w706:u16)
    n2235 = local read "Ring 24"() -> (w699:u16)
    n2236 = local read "Ring 29"() -> (w700:u16)
    n2237 = local read "Ring 34"() -> (w701:u16)
    n2238 = local read "Ring 39"() -> (w702:u16)
    n2239 = Equal?(x=w472, y=u16 2) -> (x = y?=w484:bool)
    n2240 = Equal?(x=w471, y=u16 2) -> (x = y?=w481:bool)
    n2241 = Equal?(x=w470, y=u16 2) -> (x = y?=w482:bool)
    n2242 = Equal?(x=w469, y=u16 2) -> (x = y?=w483:bool)
    n2243 = Equal?(x=w476, y=u16 2) -> (x = y?=w485:bool)
    n2244 = Equal?(x=w475, y=u16 2) -> (x = y?=w488:bool)
    n2245 = Equal?(x=w474, y=u16 2) -> (x = y?=w487:bool)
    n2246 = Equal?(x=w473, y=u16 2) -> (x = y?=w486:bool)
    n2247 = Equal?(x=w480, y=u16 2) -> (x = y?=w492:bool)
    n2248 = Equal?(x=w479, y=u16 2) -> (x = y?=w489:bool)
    n2249 = Equal?(x=w478, y=u16 2) -> (x = y?=w490:bool)
    n2250 = Equal?(x=w477, y=u16 2) -> (x = y?=w491:bool)
    n2251 = Compound Arithmetic op=AND(w484, w481, w482, w483) -> (w413:bool)
    n2252 = Compound Arithmetic op=AND(w485, w488, w487, w486) -> (w412:bool)
    n2253 = Compound Arithmetic op=AND(w492, w489, w490, w491) -> (w414:bool)
    n2254 = Equal?(x=w707, y=u16 2) -> (x = y?=w691:bool)
    n2255 = Equal?(x=w708, y=u16 2) -> (x = y?=w694:bool)
    n2256 = Equal?(x=w709, y=u16 2) -> (x = y?=w693:bool)
    n2257 = Equal?(x=w710, y=u16 2) -> (x = y?=w692:bool)
    n2258 = Equal?(x=w703, y=u16 2) -> (x = y?=w683:bool)
    n2259 = Equal?(x=w704, y=u16 2) -> (x = y?=w686:bool)
    n2260 = Equal?(x=w705, y=u16 2) -> (x = y?=w685:bool)
    n2261 = Equal?(x=w706, y=u16 2) -> (x = y?=w684:bool)
    n2262 = Equal?(x=w699, y=u16 2) -> (x = y?=w675:bool)
    n2263 = Equal?(x=w700, y=u16 2) -> (x = y?=w678:bool)
    n2264 = Equal?(x=w701, y=u16 2) -> (x = y?=w677:bool)
    n2265 = Equal?(x=w702, y=u16 2) -> (x = y?=w676:bool)
    n2266 = local read "Ring 13"() -> (w424:u16)
    n2267 = local read "Ring 20"() -> (w423:u16)
    n2268 = local read "Ring 27"() -> (w422:u16)
    n2269 = local read "Ring 34"() -> (w421:u16)
    n2270 = local read "Ring 20"() -> (w428:u16)
    n2271 = local read "Ring 27"() -> (w427:u16)
    n2272 = local read "Ring 34"() -> (w426:u16)
    n2273 = local read "Ring 41"() -> (w425:u16)
    n2274 = local read "Ring 19"() -> (w432:u16)
    n2275 = local read "Ring 26"() -> (w431:u16)
    n2276 = local read "Ring 33"() -> (w430:u16)
    n2277 = local read "Ring 40"() -> (w429:u16)
    n2278 = Compound Arithmetic op=AND(w691, w694, w693, w692) -> (w720:bool)
    n2279 = Compound Arithmetic op=AND(w683, w686, w685, w684) -> (w721:bool)
    n2280 = Compound Arithmetic op=AND(w675, w678, w677, w676) -> (w722:bool)
    n2281 = Equal?(x=w424, y=u16 2) -> (x = y?=w440:bool)
    n2282 = Equal?(x=w423, y=u16 2) -> (x = y?=w437:bool)
    n2283 = Equal?(x=w422, y=u16 2) -> (x = y?=w438:bool)
    n2284 = Equal?(x=w421, y=u16 2) -> (x = y?=w439:bool)
    n2285 = Equal?(x=w428, y=u16 2) -> (x = y?=w448:bool)
    n2286 = Equal?(x=w427, y=u16 2) -> (x = y?=w445:bool)
    n2287 = Equal?(x=w426, y=u16 2) -> (x = y?=w446:bool)
    n2288 = Equal?(x=w425, y=u16 2) -> (x = y?=w447:bool)
    n2289 = Equal?(x=w432, y=u16 2) -> (x = y?=w456:bool)
    n2290 = Equal?(x=w431, y=u16 2) -> (x = y?=w453:bool)
    n2291 = Equal?(x=w430, y=u16 2) -> (x = y?=w454:bool)
    n2292 = Equal?(x=w429, y=u16 2) -> (x = y?=w455:bool)
    n2293 = Compound Arithmetic op=AND(w440, w437, w438, w439) -> (w411:bool)
    n2294 = Compound Arithmetic op=AND(w448, w445, w446, w447) -> (w410:bool)
    n2295 = Compound Arithmetic op=AND(w456, w453, w454, w455) -> (w409:bool)
    n2296 = Compound Arithmetic op=OR(w711, w712, w713, w714, w715, w716, w717, w718, w719, w720, w721, w722) -> (w590:bool)
    n2297 = case shown="True" w590 {
      selector: w590 -> [_ w2197]
      frame False {
      }
      frame True {
        n2298 = property on="Player Rojo" class="DigNum (strict)"() -> ("Value"=w2199:dbl)  [unwired: 2 in, 2 out]
        n2299 = Increment(x=w2199) -> (x+1=w2198:dbl)
        n2300 = call "Display Message to User6"("Enable"=w2197) -> ()  [unwired: 9 in, 2 out]
        n2301 = property on="Player Rojo" class="DigNum (strict)"("Value"=w2198) -> ()  [unwired: 2 in, 2 out]
      }
    }
    n2302 = Compound Arithmetic op=OR(w420, w419, w418, w417, w416, w415, w414, w413, w412, w411, w410, w409) -> (w541:bool)
    n2303 = case shown="True" w541 {
      selector: w541 -> [_ w2194]
      frame False {
      }
      frame True {
        n2304 = property on="Player Rojo" class="DigNum (strict)"() -> ("Value"=w2196:dbl)  [unwired: 2 in, 2 out]
        n2305 = Increment(x=w2196) -> (x+1=w2195:dbl)
        n2306 = call "Display Message to User7"("Enable"=w2194) -> ()  [unwired: 9 in, 2 out]
        n2307 = property on="Player Rojo" class="DigNum (strict)"("Value"=w2195) -> ()  [unwired: 2 in, 2 out]
      }
    }
    n2308 = local read "Ring 19"() -> (w392:u16)
    n2309 = local read "Ring 14"() -> (w390:u16)
    n2310 = local read "Ring 10"() -> (w406:u16)
    n2311 = local read "Ring 15"() -> (w407:u16)
    n2312 = local read "Ring 20"() -> (w408:u16)
    n2313 = local read "Ring 10"() -> (w375:u16)
    n2314 = local read "Ring 15"() -> (w372:u16)
    n2315 = local read "Ring 20"() -> (w373:u16)
    n2316 = local read "Ring 25"() -> (w374:u16)
    n2317 = local read "Ring 9"() -> (w388:u16)
    n2318 = local read "Ring 4"() -> (w386:u16)
    n2319 = local read "Ring 5"() -> (w405:u16)
    n2320 = Equal?(x=w392, y=u16 1) -> (x = y?=w393:bool)
    n2321 = Equal?(x=w390, y=u16 1) -> (x = y?=w394:bool)
    n2322 = Equal?(x=w388, y=u16 1) -> (x = y?=w395:bool)
    n2323 = Equal?(x=w386, y=u16 1) -> (x = y?=w396:bool)
    n2324 = Equal?(x=w405, y=u16 1) -> (x = y?=w401:bool)
    n2325 = Equal?(x=w406, y=u16 1) -> (x = y?=w402:bool)
    n2326 = Equal?(x=w407, y=u16 1) -> (x = y?=w403:bool)
    n2327 = Equal?(x=w408, y=u16 1) -> (x = y?=w404:bool)
    n2328 = Equal?(x=w375, y=u16 1) -> (x = y?=w379:bool)
    n2329 = Equal?(x=w372, y=u16 1) -> (x = y?=w378:bool)
    n2330 = Equal?(x=w373, y=u16 1) -> (x = y?=w377:bool)
    n2331 = Equal?(x=w374, y=u16 1) -> (x = y?=w376:bool)
    n2332 = Compound Arithmetic op=AND(w393, w394, w395, w396) -> (w263:bool)
    n2333 = Compound Arithmetic op=AND(w401, w402, w403, w404) -> (w262:bool)
    n2334 = Compound Arithmetic op=AND(w379, w378, w377, w376) -> (w261:bool)
    n2335 = local read "Ring 10"() -> (w113:u16)
    n2336 = local read "Ring 17"() -> (w115:u16)
    n2337 = local read "Ring 24"() -> (w117:u16)
    n2338 = local read "Ring 16"() -> (w96:u16)
    n2339 = local read "Ring 23"() -> (w95:u16)
    n2340 = local read "Ring 16"() -> (w131:u16)
    n2341 = local read "Ring 23"() -> (w130:u16)
    n2342 = local read "Ring 30"() -> (w129:u16)
    n2343 = local read "Ring 3"() -> (w111:u16)
    n2344 = local read "Ring 2"() -> (w98:u16)
    n2345 = local read "Ring 9"() -> (w97:u16)
    n2346 = local read "Ring 9"() -> (w128:u16)
    n2347 = local read "Ring 11"() -> (w351:u16)
    n2348 = local read "Ring 16"() -> (w350:u16)
    n2349 = local read "Ring 16"() -> (w363:u16)
    n2350 = local read "Ring 21"() -> (w362:u16)
    n2351 = local read "Ring 26"() -> (w361:u16)
    n2352 = local read "Ring 6"() -> (w340:u16)
    n2353 = local read "Ring 11"() -> (w339:u16)
    n2354 = local read "Ring 16"() -> (w338:u16)
    n2355 = local read "Ring 21"() -> (w337:u16)
    n2356 = local read "Ring 21"() -> (w349:u16)
    n2357 = local read "Ring 26"() -> (w348:u16)
    n2358 = local read "Ring 31"() -> (w360:u16)
    n2359 = Equal?(x=w111, y=u16 1) -> (x = y?=w110:bool)
    n2360 = Equal?(x=w113, y=u16 1) -> (x = y?=w109:bool)
    n2361 = Equal?(x=w115, y=u16 1) -> (x = y?=w108:bool)
    n2362 = Equal?(x=w117, y=u16 1) -> (x = y?=w107:bool)
    n2363 = Equal?(x=w98, y=u16 1) -> (x = y?=w102:bool)
    n2364 = Equal?(x=w97, y=u16 1) -> (x = y?=w101:bool)
    n2365 = Equal?(x=w96, y=u16 1) -> (x = y?=w100:bool)
    n2366 = Equal?(x=w95, y=u16 1) -> (x = y?=w99:bool)
    n2367 = Equal?(x=w128, y=u16 1) -> (x = y?=w124:bool)
    n2368 = Equal?(x=w131, y=u16 1) -> (x = y?=w125:bool)
    n2369 = Equal?(x=w130, y=u16 1) -> (x = y?=w126:bool)
    n2370 = Equal?(x=w129, y=u16 1) -> (x = y?=w127:bool)
    n2371 = Equal?(x=w340, y=u16 1) -> (x = y?=w336:bool)
    n2372 = Equal?(x=w339, y=u16 1) -> (x = y?=w343:bool)
    n2373 = Equal?(x=w338, y=u16 1) -> (x = y?=w342:bool)
    n2374 = Equal?(x=w337, y=u16 1) -> (x = y?=w341:bool)
    n2375 = Equal?(x=w351, y=u16 1) -> (x = y?=w356:bool)
    n2376 = Equal?(x=w350, y=u16 1) -> (x = y?=w357:bool)
    n2377 = Equal?(x=w349, y=u16 1) -> (x = y?=w358:bool)
    n2378 = Equal?(x=w348, y=u16 1) -> (x = y?=w359:bool)
    n2379 = Equal?(x=w363, y=u16 1) -> (x = y?=w367:bool)
    n2380 = Equal?(x=w362, y=u16 1) -> (x = y?=w366:bool)
    n2381 = Equal?(x=w361, y=u16 1) -> (x = y?=w365:bool)
    n2382 = Equal?(x=w360, y=u16 1) -> (x = y?=w364:bool)
    n2383 = Compound Arithmetic op=AND(w110, w109, w108, w107) -> (w240:bool)
    n2384 = Compound Arithmetic op=AND(w102, w101, w100, w99) -> (w241:bool)
    n2385 = Compound Arithmetic op=AND(w124, w125, w126, w127) -> (w242:bool)
    n2386 = Compound Arithmetic op=AND(w336, w343, w342, w341) -> (w260:bool)
    n2387 = Compound Arithmetic op=AND(w356, w357, w358, w359) -> (w259:bool)
    n2388 = Compound Arithmetic op=AND(w367, w366, w365, w364) -> (w258:bool)
    n2389 = local read "Ring 15"() -> (w153:u16)
    n2390 = local read "Ring 15"() -> (w140:u16)
    n2391 = local read "Ring 22"() -> (w141:u16)
    n2392 = local read "Ring 29"() -> (w142:u16)
    n2393 = local read "Ring 1"() -> (w163:u16)
    n2394 = local read "Ring 15"() -> (w165:u16)
    n2395 = local read "Ring 22"() -> (w166:u16)
    n2396 = local read "Ring 8"() -> (w152:u16)
    n2397 = local read "Ring 22"() -> (w154:u16)
    n2398 = local read "Ring 29"() -> (w155:u16)
    n2399 = local read "Ring 36"() -> (w143:u16)
    n2400 = local read "Ring 8"() -> (w164:u16)
    n2401 = local read "Ring 17"() -> (w315:u16)
    n2402 = local read "Ring 22"() -> (w314:u16)
    n2403 = local read "Ring 27"() -> (w313:u16)
    n2404 = local read "Ring 32"() -> (w312:u16)
    n2405 = local read "Ring 22"() -> (w319:u16)
    n2406 = local read "Ring 27"() -> (w318:u16)
    n2407 = local read "Ring 32"() -> (w317:u16)
    n2408 = local read "Ring 37"() -> (w316:u16)
    n2409 = local read "Ring 12"() -> (w323:u16)
    n2410 = local read "Ring 17"() -> (w322:u16)
    n2411 = local read "Ring 22"() -> (w321:u16)
    n2412 = local read "Ring 27"() -> (w320:u16)
    n2413 = Equal?(x=w163, y=u16 1) -> (x = y?=w167:bool)
    n2414 = Equal?(x=w164, y=u16 1) -> (x = y?=w160:bool)
    n2415 = Equal?(x=w165, y=u16 1) -> (x = y?=w161:bool)
    n2416 = Equal?(x=w166, y=u16 1) -> (x = y?=w162:bool)
    n2417 = Equal?(x=w152, y=u16 1) -> (x = y?=w147:bool)
    n2418 = Equal?(x=w153, y=u16 1) -> (x = y?=w146:bool)
    n2419 = Equal?(x=w154, y=u16 1) -> (x = y?=w145:bool)
    n2420 = Equal?(x=w155, y=u16 1) -> (x = y?=w144:bool)
    n2421 = Equal?(x=w140, y=u16 1) -> (x = y?=w136:bool)
    n2422 = Equal?(x=w141, y=u16 1) -> (x = y?=w137:bool)
    n2423 = Equal?(x=w142, y=u16 1) -> (x = y?=w138:bool)
    n2424 = Equal?(x=w143, y=u16 1) -> (x = y?=w139:bool)
    n2425 = Equal?(x=w315, y=u16 1) -> (x = y?=w327:bool)
    n2426 = Equal?(x=w314, y=u16 1) -> (x = y?=w324:bool)
    n2427 = Equal?(x=w313, y=u16 1) -> (x = y?=w325:bool)
    n2428 = Equal?(x=w312, y=u16 1) -> (x = y?=w326:bool)
    n2429 = Equal?(x=w319, y=u16 1) -> (x = y?=w328:bool)
    n2430 = Equal?(x=w318, y=u16 1) -> (x = y?=w331:bool)
    n2431 = Equal?(x=w317, y=u16 1) -> (x = y?=w330:bool)
    n2432 = Equal?(x=w316, y=u16 1) -> (x = y?=w329:bool)
    n2433 = Equal?(x=w323, y=u16 1) -> (x = y?=w335:bool)
    n2434 = Equal?(x=w322, y=u16 1) -> (x = y?=w332:bool)
    n2435 = Equal?(x=w321, y=u16 1) -> (x = y?=w333:bool)
    n2436 = Equal?(x=w320, y=u16 1) -> (x = y?=w334:bool)
    n2437 = Compound Arithmetic op=AND(w167, w160, w161, w162) -> (w243:bool)
    n2438 = Compound Arithmetic op=AND(w147, w146, w145, w144) -> (w244:bool)
    n2439 = Compound Arithmetic op=AND(w136, w137, w138, w139) -> (w245:bool)
    n2440 = Compound Arithmetic op=AND(w327, w324, w325, w326) -> (w256:bool)
    n2441 = Compound Arithmetic op=AND(w328, w331, w330, w329) -> (w255:bool)
    n2442 = Compound Arithmetic op=AND(w335, w332, w333, w334) -> (w257:bool)
    n2443 = local read "Ring 14"() -> (w188:u16)
    n2444 = local read "Ring 21"() -> (w189:u16)
    n2445 = local read "Ring 28"() -> (w190:u16)
    n2446 = local read "Ring 35"() -> (w191:u16)
    n2447 = local read "Ring 21"() -> (w184:u16)
    n2448 = local read "Ring 28"() -> (w185:u16)
    n2449 = local read "Ring 35"() -> (w186:u16)
    n2450 = local read "Ring 42"() -> (w187:u16)
    n2451 = local read "Ring 14"() -> (w181:u16)
    n2452 = local read "Ring 21"() -> (w182:u16)
    n2453 = local read "Ring 28"() -> (w183:u16)
    n2454 = local read "Ring 7"() -> (w180:u16)
    n2455 = local read "Ring 18"() -> (w267:u16)
    n2456 = local read "Ring 23"() -> (w266:u16)
    n2457 = local read "Ring 28"() -> (w265:u16)
    n2458 = local read "Ring 33"() -> (w264:u16)
    n2459 = local read "Ring 23"() -> (w271:u16)
    n2460 = local read "Ring 28"() -> (w270:u16)
    n2461 = local read "Ring 33"() -> (w269:u16)
    n2462 = local read "Ring 38"() -> (w268:u16)
    n2463 = local read "Ring 24"() -> (w275:u16)
    n2464 = local read "Ring 29"() -> (w274:u16)
    n2465 = local read "Ring 34"() -> (w273:u16)
    n2466 = local read "Ring 39"() -> (w272:u16)
    n2467 = Equal?(x=w188, y=u16 1) -> (x = y?=w176:bool)
    n2468 = Equal?(x=w189, y=u16 1) -> (x = y?=w179:bool)
    n2469 = Equal?(x=w190, y=u16 1) -> (x = y?=w178:bool)
    n2470 = Equal?(x=w191, y=u16 1) -> (x = y?=w177:bool)
    n2471 = Equal?(x=w184, y=u16 1) -> (x = y?=w175:bool)
    n2472 = Equal?(x=w185, y=u16 1) -> (x = y?=w172:bool)
    n2473 = Equal?(x=w186, y=u16 1) -> (x = y?=w173:bool)
    n2474 = Equal?(x=w187, y=u16 1) -> (x = y?=w174:bool)
    n2475 = Equal?(x=w180, y=u16 1) -> (x = y?=w168:bool)
    n2476 = Equal?(x=w181, y=u16 1) -> (x = y?=w171:bool)
    n2477 = Equal?(x=w182, y=u16 1) -> (x = y?=w170:bool)
    n2478 = Equal?(x=w183, y=u16 1) -> (x = y?=w169:bool)
    n2479 = Equal?(x=w267, y=u16 1) -> (x = y?=w283:bool)
    n2480 = Equal?(x=w266, y=u16 1) -> (x = y?=w280:bool)
    n2481 = Equal?(x=w265, y=u16 1) -> (x = y?=w281:bool)
    n2482 = Equal?(x=w264, y=u16 1) -> (x = y?=w282:bool)
    n2483 = Equal?(x=w271, y=u16 1) -> (x = y?=w291:bool)
    n2484 = Equal?(x=w270, y=u16 1) -> (x = y?=w288:bool)
    n2485 = Equal?(x=w269, y=u16 1) -> (x = y?=w289:bool)
    n2486 = Equal?(x=w268, y=u16 1) -> (x = y?=w290:bool)
    n2487 = Equal?(x=w275, y=u16 2) -> (x = y?=w299:bool)
    n2488 = Equal?(x=w274, y=u16 1) -> (x = y?=w296:bool)
    n2489 = Equal?(x=w273, y=u16 1) -> (x = y?=w297:bool)
    n2490 = Equal?(x=w272, y=u16 1) -> (x = y?=w298:bool)
    n2491 = Compound Arithmetic op=AND(w176, w179, w178, w177) -> (w247:bool)
    n2492 = Compound Arithmetic op=AND(w175, w172, w173, w174) -> (w248:bool)
    n2493 = Compound Arithmetic op=AND(w168, w171, w170, w169) -> (w246:bool)
    n2494 = Compound Arithmetic op=AND(w283, w280, w281, w282) -> (w254:bool)
    n2495 = Compound Arithmetic op=AND(w291, w288, w289, w290) -> (w253:bool)
    n2496 = Compound Arithmetic op=AND(w299, w296, w297, w298) -> (w252:bool)
    n2497 = local read "Ring 13"() -> (w236:u16)
    n2498 = local read "Ring 20"() -> (w237:u16)
    n2499 = local read "Ring 27"() -> (w238:u16)
    n2500 = local read "Ring 34"() -> (w239:u16)
    n2501 = local read "Ring 20"() -> (w232:u16)
    n2502 = local read "Ring 27"() -> (w233:u16)
    n2503 = local read "Ring 34"() -> (w234:u16)
    n2504 = local read "Ring 41"() -> (w235:u16)
    n2505 = local read "Ring 19"() -> (w228:u16)
    n2506 = local read "Ring 26"() -> (w229:u16)
    n2507 = local read "Ring 33"() -> (w230:u16)
    n2508 = local read "Ring 40"() -> (w231:u16)
    n2509 = Equal?(x=w236, y=u16 1) -> (x = y?=w220:bool)
    n2510 = Equal?(x=w237, y=u16 1) -> (x = y?=w223:bool)
    n2511 = Equal?(x=w238, y=u16 1) -> (x = y?=w222:bool)
    n2512 = Equal?(x=w239, y=u16 1) -> (x = y?=w221:bool)
    n2513 = Equal?(x=w232, y=u16 1) -> (x = y?=w212:bool)
    n2514 = Equal?(x=w233, y=u16 1) -> (x = y?=w215:bool)
    n2515 = Equal?(x=w234, y=u16 1) -> (x = y?=w214:bool)
    n2516 = Equal?(x=w235, y=u16 1) -> (x = y?=w213:bool)
    n2517 = Equal?(x=w228, y=u16 1) -> (x = y?=w204:bool)
    n2518 = Equal?(x=w229, y=u16 1) -> (x = y?=w207:bool)
    n2519 = Equal?(x=w230, y=u16 1) -> (x = y?=w206:bool)
    n2520 = Equal?(x=w231, y=u16 1) -> (x = y?=w205:bool)
    n2521 = Compound Arithmetic op=OR(w263, w262, w261, w260, w259, w258, w257, w256, w255, w254, w253, w252) -> (w384:bool)
    n2522 = Compound Arithmetic op=AND(w220, w223, w222, w221) -> (w249:bool)
    n2523 = Compound Arithmetic op=AND(w212, w215, w214, w213) -> (w250:bool)
    n2524 = Compound Arithmetic op=AND(w204, w207, w206, w205) -> (w251:bool)
    n2525 = case shown="True" w384 {
      selector: w384 -> [_ w2191]
      frame False {
      }
      frame True {
        n2526 = property on="Player Verde" class="DigNum (strict)"() -> ("Value"=w2193:dbl)  [unwired: 2 in, 2 out]
        n2527 = Increment(x=w2193) -> (x+1=w2192:dbl)
        n2528 = call "Display Message to User8"("Enable"=w2191) -> ()  [unwired: 9 in, 2 out]
        n2529 = property on="Player Verde" class="DigNum (strict)"("Value"=w2192) -> ()  [unwired: 2 in, 2 out]
      }
    }
    n2530 = Compound Arithmetic op=OR(w240, w241, w242, w243, w244, w245, w246, w247, w248, w249, w250, w251) -> (w119:bool)
    n2531 = case shown="True" w119 {
      selector: w119 -> [_ w2188]
      frame False {
      }
      frame True {
        n2532 = property on="Player Verde" class="DigNum (strict)"() -> ("Value"=w2190:dbl)  [unwired: 2 in, 2 out]
        n2533 = Increment(x=w2190) -> (x+1=w2189:dbl)
        n2534 = call "Display Message to User9"("Enable"=w2188) -> ()  [unwired: 9 in, 2 out]
        n2535 = property on="Player Verde" class="DigNum (strict)"("Value"=w2189) -> ()  [unwired: 2 in, 2 out]
      }
    }
  }
